vi "AlliGator.vi"() -> ()   [LabVIEW 2021, in "AlliGator GUI.lvlib"]
doc: "AlliGator main window.\nSpawned by AlliGator Launcher.vi.\nSpawns AlliGator Action Loop.vi, which handles UI requests from AlliGator.vi"
uses:
  AlliGator GUI.lvlib
  AlliGator Main Window Tabs.ctl
  Phasor/Phasor (g, s).ctl
  Source Image/AlliGator Displayed Image.ctl
  AlliGator State Indicator.ctl
  Phasor/Phasor (m, phi).ctl
  Phasor/Phasor Ratio Type.ctl
  Fits/IRF(X)PSED/Decay Fit Parameters & Derived Quantities List v2.ctl
  Phasor/Phasor Calibration Type.ctl
  Histograms/Linear Histogram Options.ctl
  Histograms/Histogram Bin Option.ctl
  Histograms/Histogram Bin Position.ctl
  Action Engine/AlliGator Q Element.ctl
  Action Engine/AlliGator Q Event.ctl
  AlliGator Dataset Ctrl Refnums.ctl
  AlliGator Other Ctrl Refnums.ctl
  AlliGator Registered Events Ctrl Refnums.ctl
  AlliGator Ctrl Refnums.ctl
  AlliGator Phasor Plot Ctrl Refnums.ctl
  AlliGator Phasor Graph Ctrl Refnums.ctl
  AlliGator Image Histogram Control Refnums.ctl
  Decay Fit Parameter Map/AlliGator Decay Fit Map Control Refnums.ctl
  Parameter Map/AlliGator Parameter Map Control Refnums.ctl
  Globals, Variables, Constants/AlliGator Refnums List.ctl
  Settings/AlliGator Settings List.ctl
  Rich Text Box/Text Format List.ctl
  Globals, Variables, Constants/AlliGator Variables List.ctl
  Palette/Image Palette Information.ctl
  Image/Image Display Palette Type.ctl
  Image/Image Display Event.ctl
  Image/Image Control Refnum.ctl
  <vilib>/Utility/miscctls.llb/LVPoint32TypeDef.ctl
  Decay Fit Parameter Map/AlliGator Decay Parameter Map Update Event Data.ctl
  Graphs/XY Graph/XY Graph Event.ctl
  Utilities/Read-Write.ctl
  Graphs/XY Graph/New Plot Information.ctl
  Graphs/Plot Scales.ctl
  Graphs/LabVIEW Plot Interpolation.ctl
  Graphs/Plot Point Style.ctl
  Graphs/XY Graph/XY Graph Mouse Click Event Data.ctl
  Graphs/XY Graph/XY Graph Refnum.ctl
  Parameter Map/AlliGator Parameter Map Update Event Data.ctl
  ROIs/AlliGator ROI Manager Actions.ctl
  AlliGator Image Mouse Up Event Data.ctl
  Image/Image ROI Descriptor.ctl
  Image/Image Contour Definition.ctl
  Image/Image Contour ID.ctl
  Image/Image ROI Type.ctl
  Parameter Map/AlliGator Parameter Map Display Range Mouse Move Data.ctl
  Image/Image Display User Event Data.ctl
  Action Engine/AlliGator Action Loop.vi
  Variant/Variant to Data/Variant to Boolean.vi
  Phasor/Phasor Abort Parallel Computation.vi
  Fits/Abort Fit Global.vi
  Image/Abort ROI Creation Global.vi
  Globals, Variables, Constants/AlliGator Abort.vi
  Variant/Variant to Data/Variant to [String].vi
  <vilib>/Utility/inputDevices.llb/keyboardAcquire.vi
  <vilib>/Utility/inputDevices.llb/mouseAcquire.vi
  Globals, Variables, Constants/AlliGator Globals.vi
  <vilib>/Utility/inputDevices.llb/closeKeyboard.vi
  <vilib>/Utility/inputDevices.llb/closeMouse.vi
  Action Engine/AlliGator Action Engine.lvlib
  Variant/Variant to Data/Variant to Data.lvlib
  Error/Error.lvlib
  Globals, Variables, Constants/AlliGator Globals, Variables & Constants.lvlib
  Image/Image.lvlib
  Palette/Palette.lvlib
  Notebook/Notebook.lvlib
  Graphs/XY Graph/XY Graph Add-Ons.lvlib
  Settings/AlliGator Settings.lvlib
  Phasor/Phasor.lvlib
  Fits/Fits.lvlib
  Phasor Calibration/AlliGator Phasor Calibration.lvlib
  Phasor Plot/AlliGator Phasor Plot.lvlib
  Source Image/AlliGator Source Image.lvlib
  Phasor Graph/AlliGator Phasor Graph.lvlib
  ROIs/AlliGator ROIs.lvlib
  GUI/GUI.lvlib
  Decay Fit Parameter Map/AlliGator Decay Fit Parameter Map.lvlib
  Python Plugins API/AlliGator Python Plugins.lvlib
  Sound/Sound.lvlib
  Graphs/Graphs.lvlib
  Decay Analysis/Decay Processing/AlliGator Decay Processing.lvlib
  Utilities/Utilities.lvlib
  Parameter Map/AlliGator Parameter Map.lvlib
  Histograms/Histogram Window.lvlib
panel:
  in  "Current ROI Analysis":bool
  in  "Scale Bar":bool
  in  "Refresh Image":bool
  in  "Clear Image Overlay":bool
  in  "Use ROI as Search Area":bool
  in  "Highlight Image ROI":bool
  in  "Phasor Overlay Color":u32(colorbox)=16777216
  in  "Gate Image Slide":u16(slide)=9 min=1 max=135 scale=1.0..201.0
  in  "Dataset File/Folder Path":path caption="File/Folder Path"
  out "Source Image":T1(plugin-control)
  out "True Pixel Value":dbl format="%#_5g"
  in  "Source Image ROI Selection":i32(c297)
  in  "Source Image ROI Color":u32(colorbox)=6618880 caption="ROI Color"
  in  "Time Point Slide":u16(slide)=65535 min=1 step=1 scale=1.0..1.1
  in  "Image Color Scale":dbl(ramp)
  in  "Channel Name":u16(ring) items=["Gate"]
  out "Current Time Stamp":dbl caption="Time Stamp" format="%#_5g"
  out "CPU":dbl[unit] format="%^#_4e"
  in  "Save Source Image":bool caption="Save Image"
  out "Current Data":string="Stained cancer cells" caption="Current Folder"
  in  "Displayed Image":T2=enum."Sum of All Gates"
  in  "Tab Control":T3=enum."Lifetime & Other Parameters"
  in  "Dataset File/Folder Path 2":path caption="File/Folder Path"
  in  "Histogram Lower Percentile":dbl=1.0 caption="Lower Percentile" min=0.0 max=100.0 format="%#.3f"
  in  "Histogram Upper Percentile":dbl=1.0 caption="100 - Upper Percentile" min=0.0 max=100.0 format="%#.3f"
  in  "Image Histogram Options":T4={"Bin Size"=1.0, "Bin Number"=256, "Bin Option"=enum."Bin Number", "Min Value"=-inf, "Max Value"=inf, "Filter NaN & Infinite Values"=TRUE, "Frequency Plot"=FALSE, "Align Bins"=TRUE, "Bin Location"=enum."Left", "Project Outside Values"=FALSE, "Max Histogram Size"=1000000} {"Max Histogram Size" format="%.0e"}
  in  "Auto-Adjust Contrast":bool=TRUE
  out "Lower Percentile":dbl=nan format="%#.3f"
  out "Upper Percentile":dbl=nan caption="100 - Upper Percentile" format="%#.3f"
  in  "Image Histogram Active":bool=TRUE
  in  "Use Image Histogram for Contrast":bool=TRUE
  out "Image Histogram":cluster{"X Array":dbl[], "Y Array":dbl[]}[](graph)
  in  "Dataset File/Folder Path 3":path caption="File/Folder Path"
  out "Decay Graph TipStrip":string caption="Lifetime Graph TipStrip"
  out "Decay Integrated Intensity":dbl=46949635.0 caption="Bkgd-subtracted Intensity" format="%#_5g"
  out "Decay Background":dbl caption="Background" format="%#_5g"
  out "Decay Lifetime":dbl[unit] caption="Lifetime" format="%#_5g"
  out "Decay Graph":cluster{"X Array":dbl[], "Y Array":dbl[]}[](graph)
  in  "Decay Graph Active":bool=TRUE
  in  "Dataset File/Folder Path 4":path caption="File/Folder Path"
  out "Decay Statistics TipStrip":string caption="Lifetime Graph TipStrip"
  out "Decay Statistics Graph":cluster{"X Array":dbl[], "Y Array":dbl[]}[](graph)
  in  "Decay Statistics Bin":i32=1 min=1
  in  "Dataset File/Folder Path 5":path caption="File/Folder Path"
  out "Intensity Time Trace TipStrip":string caption="Lifetime Graph TipStrip"
  in  "Intensity Correction File":path
  in  "Use Intensity Correction File":bool
  in  "Use File Timestamp":bool=TRUE
  out "Intensity Time Trace":cluster{"X Array":dbl[], "Y Array":dbl[]}[](graph)
  in  "Time Step":dbl[unit]=1.0 format="%#_5g"
  out "True Phasor Plot Value":i32
  in  "Dataset File/Folder Path 6":path caption="File/Folder Path"
  in  "Phasor ROI Decay":bool
  in  "Phasor Plot ROI Color":u32(colorbox)=6618880
  out "Phasor Plot Average Lifetime":dbl[unit]=nan caption="<tau>_a" format="%#_4e"
  out "Phasor Plot Phasor Ratio":dbl=nan caption="Amplitude Ratio (a1)" format="%#_4e"
  out "Phasor Plot Modulus Lifetime":dbl[unit]=nan caption="Modulus Lifetime" format="%#_4e"
  out "Phasor Plot Phase Lifetime":dbl[unit]=-9.431404035075279e-09 caption="Phase Lifetime" format="%#_4e"
  out "Phasor at cursor (m, phi)":T7={"m"=1.5330078000581284, "phi"=1.7786862539971595} caption="Phasor at Cursor (m, phi)" {"phi" format="%#_4e"; "m" format="%#_4e"}
  in  "Clear Phasor Overlay":bool
  in  "Phasor Plot ROI Selection":i32(c297)
  in  "Phasor Plot Active":bool
  in  "Phasor Plot Color Scale":dbl(ramp)
  out "Phasor at cursor (g, s)":T8={"g"=-0.31640625, "s"=1.5} caption="Phasor at Cursor" {"s" format="%#.3e"; "g" format="%#_4e"}
  in  "Phasor Plot Display Range":cluster{u32, u32}(slide)={0, 100} scale=0.0..987.0
  in  "Highlight Phasor in Source Image":bool caption="Highlight Phasor ROI"
  in  "Image Overlay Color":u32(colorbox)=16777216
  in  "Refresh Phasor Plot":bool caption="Refresh Phsor Plot"
  in  "Save Phasor Plot":bool
  out "Reference 2 Button":bool caption="Reference"
  out "Reference 1 Button":bool caption="Reference"
  in  "Phasor Plot Frequency":dbl[unit]=80000000.0 caption="Phasor Frequency"
  in  "Overlay Mode":u16(ring)
  out "Phasor Plot Image":T1(plugin-control)
  in  "Dataset File/Folder Path 7":path caption="File/Folder Path"
  out "Phasor Graph TipStrip":string caption="Lifetime Graph TipStrip"
  out "Average Lifetime SDV":dbl[unit]=nan caption="+/-" format="%#.3g"
  out "Phasor Ratio SDV":dbl=nan caption="+/-" format="%#.3g"
  out "Modulus Lifetime SDV":dbl[unit]=nan caption="+/-" format="%#.3g"
  out "Phase Lifetime SDV":dbl[unit]=nan caption="+/-" format="%#.3g"
  in  "Calibration Type":T9
  out "Phasor Graph Average Lifetime":dbl[unit]=nan caption="<tau>_a" format="%#.3g"
  in  "Phasor Graph Active":bool
  in  "Refresh SEPL":bool
  out "Phasor Graph Phasor Ratio":dbl=nan caption="Amplitude Ratio (a1)" format="%#.3g"
  out "Phasor Graph Modulus Lifetime":dbl[unit]=nan caption="Modulus Lifetime" format="%#.3g"
  in  "Phasor Reference 2 Control":dbl(c297)
  in  "Save Phasor Graph Image":bool
  in  "Current Phasor (m, phi)":T7={"m"=nan, "phi"=nan} {"phi" format="%#_4g"; "m" format="%#_4g"}
  in  "Phasor Reference 1 Control":dbl(c297)
  in  "Single Step Phasor":bool
  in  "Phasor Frame Slide":i32(slide) caption="Phasor Frame Slider" min=0 step=1 scale=1.0..1.1
  out "Phase Lifetime 2":dbl[unit]=nan format="%#.3g"
  out "Phase Lifetime 1":dbl[unit]=nan format="%#.3g"
  in  "Show Line":bool
  out "Phasor Graph Phase Lifetime":dbl[unit]=nan caption="Phase Lifetime" format="%#.3g"
  in  "Current Phasor (g, s)":T8={"g"=nan, "s"=nan} caption="Current Phasor" {"s" format="%#_4g"; "g" format="%#_4g"}
  out "Phasor Graph":cluster{"X Array":dbl[], "Y Array":dbl[]}[](graph)
  in  "Phasor Graph Frequency":dbl[unit]=80000000.0 caption="Phasor Frequency"
  in  "Calibration Lifetime":dbl[unit] min=0.0
  in  "Dataset File/Folder Path 8":path caption="File/Folder Path"
  out "Phasor Ratio Graph TipStrip":string caption="Lifetime Graph TipStrip"
  in  "Phasor Ratio Type":T10
  out "Phasor Ratio Graph":cluster{"X Array":dbl[], "Y Array":dbl[]}[](graph)
  in  "Dataset File/Folder Path 9":path caption="File/Folder Path"
  out "Lifetime & Other Parameters Graph TipStrip":string caption="Lifetime Graph TipStrip"
  out "Lifetime & Other Parameters Graph":cluster{"X Array":dbl[], "Y Array":dbl[]}[](graph)
  in  "Dataset File/Folder Path 10":path caption="File/Folder Path"
  in  "Decay Fit Parameter Map ROI Color":u32(colorbox)=6618880
  in  "Overlay Decay Fit Parameter Map":bool
  out "Decay Fit Max Parameter":dbl=1.0 caption="Max Parameter"
  out "Decay Fit Min Parameter":dbl caption="Min Parameter"
  in  "Refresh Decay Fit Parameter Map":bool
  in  "Decay Fit Parameter":T11
  in  "Decay Fit Parameter Map Color Scale":dbl(ramp)
  in  "Decay Fit Parameter Map Display Range":cluster{dbl, dbl}(slide)={0.0, 1.0} scale=0.0..1.0
  out "Decay Parameter Map Value":dbl caption="Map Value"
  out "Decay Parameter Map Y":i32 caption="Y"
  out "Decay Parameter Map X":i32 caption="X"
  out "Decay Fit Parameter Map Image":T1(plugin-control)
  out "Parameter Map X":i32 caption="X"
  out "Parameter Map Y":i32 caption="Y"
  out "Parameter Map Value":dbl caption="Map Value"
  in  "Parameter Map Set":u16(ring)
  in  "Map Parameter":u16(ring)
  in  "Dataset File/Folder Path 11":path caption="File/Folder Path"
  in  "Parameter Map ROI Color":u32(colorbox)=6618880 caption="Decay Fit Parameter Map ROI Color"
  in  "Overlay Parameter Map":bool
  out "Map Max Parameter":dbl=1.0 caption="Max Parameter"
  out "Map Min Parameter":dbl caption="Min Parameter"
  in  "Refresh Parameter Map":bool
  in  "Parameter Map Color Scale":dbl(ramp)
  in  "Parameter Map Display Range":cluster{dbl, dbl}(slide)={0.0, 1.0} scale=0.0..20.0
  out "Parameter Map Image":T1(plugin-control)
  out "Event LED":bool
  out "Message":string
  out "Progress Bar":dbl(slide) scale=0.0..100.0
  in  "Abort ROI Creation":bool
  in  "Abort Fit":bool
  in  "Abort":bool
  out "Animated Busy Icon":bool=TRUE
  out "State Indicators":T12
  # "Drop the content of this VI on AlliGator's diagram\nIn AlliGator, replace the subVI template by a new version"
  # "Drop the content of this VI on AlliGator's diagram\nIn AlliGator, replace the subVI template by a new version"
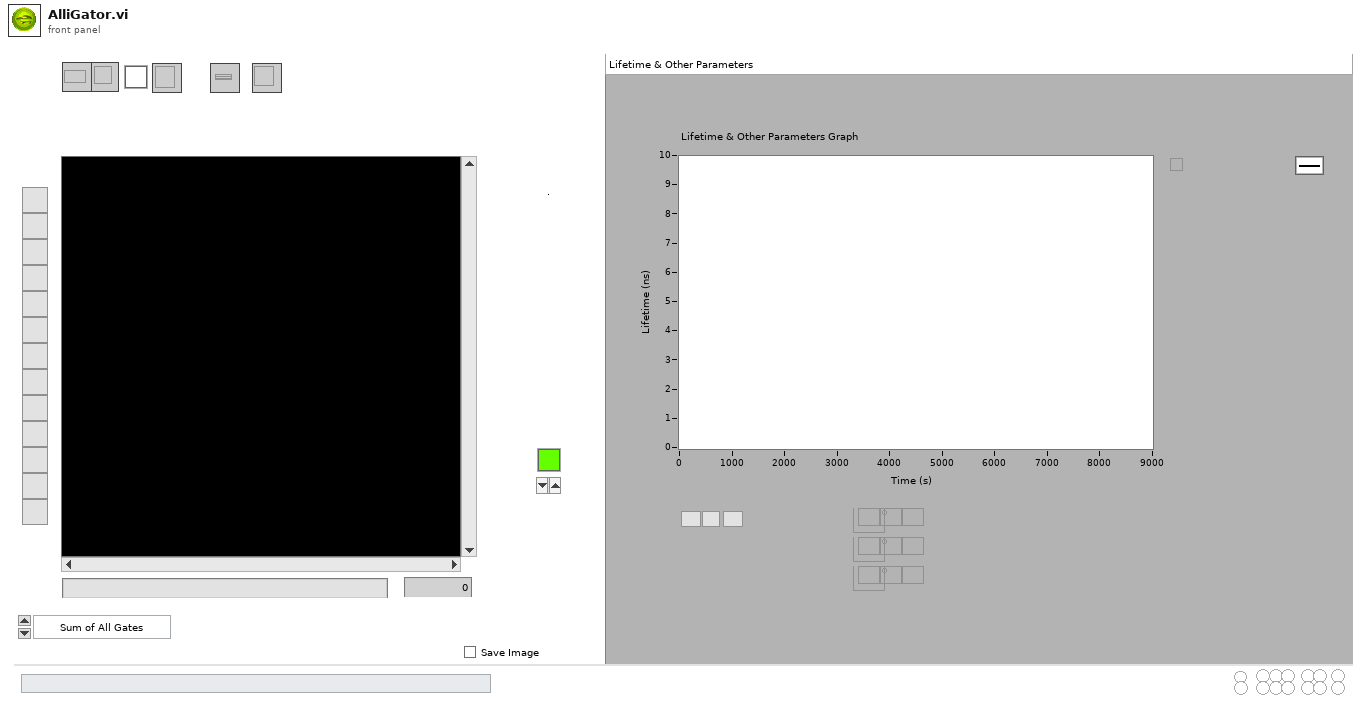
[diagram p1: front panel]
types:
  T1 = typedef "IMAQ Image.ctl" = refnum<image>
  T2 = typedef "AlliGator Source Image.lvlib/AlliGator Displayed Image.ctl" = enum16{"Single Gate", "Sum of All Gates", "Max of All Gates", "Min of All Gates", "-", "White Ligth Image", "Mask Image"}
  T3 = typedef "AlliGator GUI.lvlib/AlliGator Main Window Tabs.ctl" = enum32{"Image Histogram", "Fluorescence Decay", "Fluorescence Decay Statistics", "Intensity Time Trace", "Phasor Plot", "Phasor Graph", "Phasor Ratio", "Lifetime & Other Parameters", "Decay Fit Parameter Map", "Parameter Map"}
  T4 = typedef "Histogram Window.lvlib/Linear Histogram Options.ctl" = cluster{"Bin Size":dbl, "Bin Number":i32, "Bin Option":T5, "Min Value":dbl, "Max Value":dbl, "Filter NaN & Infinite Values":bool, "Frequency Plot":bool, "Align Bins":bool, "Bin Location":T6, "Project Outside Values":bool, "Max Histogram Size":i32}
  T5 = typedef "Histogram Window.lvlib/Histogram Bin Option.ctl" = enum32{"Bin Number", "Bin Size"}
  T6 = typedef "Histogram Window.lvlib/Histogram Bin Position.ctl" = enum16{"Left", "Center", "Right"}
  T7 = typedef "Phasor.lvlib/Phasor (m, phi).ctl" = cluster{"m":dbl, "phi":dbl}
  T8 = typedef "Phasor.lvlib/Phasor (g, s).ctl" = cluster{"g":dbl, "s":dbl}
  T9 = typedef "Phasor.lvlib/Phasor Calibration Type.ctl" = enum16{"None", "Single Phasor", "Phasor Series", "Phasor Map"}
  T10 = typedef "Phasor.lvlib/Phasor Ratio Type.ctl" = enum32{"Intensity-weighted", "Amplitude-weighted"}
  T11 = typedef "Fits.lvlib/Decay Fit Parameters & Derived Quantities List v2.ctl" = enum16{"Offset", "Baseline", "A_1", "tau_1", "A_2", "tau_2", "<tau>_a", "f1_a", "f2_a", "<tau>_i", "f1_i", "f2_i", "-", "R^2", "Chi^2"}
  T12 = typedef "AlliGator GUI.lvlib/AlliGator State Indicator.ctl" = cluster{"Phasor Calibration Defined":bool, "Phasor Calibration Series Defined":bool, "Phasor Calibration Map Defined":bool, "Phasor Ratio Reference 1 Defined":bool, "Phasor Ratio Reference 2 Defined":bool, "Phasor Ratio Lifetime Reference 1 Defined ":bool, "Phasor Ratio Lifetime Reference 2 Defined":bool, "Phasor Calibration Used":bool, "Phasor Calibration Series Used":bool, "Phasor Calibration Map Used":bool, "Dataset Update Needed":bool, "Phasor Plot Update Needed":bool, "Reference/IRF Defined":bool, "Individual IRFs Defined":bool}
  T13 = typedef "AlliGator Globals, Variables & Constants.lvlib/AlliGator Refnums List.ctl" = enum16{"---------- AlliGator Controls ----------", "AlliGator Tab Control Refnum", "---------- AlliGator Indicators ----------", "Source Image Display Refnum", "Phasor Plot Display Refnum", "Decay Fit Parameter Map Refnum", "---------- AlliGator VIs ----------", "AlliGator Refnum", "AlliGator Settings Refnum", "AlliGator Launcher Refnum"}
  T14 = typedef "AlliGator Parameter Map.lvlib/AlliGator Parameter Map Control Refnums.ctl" = cluster{"Parameter Map Color Scale":refnum<vi>, "Map Parameter":refnum<vi>, "Max Parameter":refnum<vi>, "Min Parameter":refnum<vi>, "Parameter Map Display":refnum<vi>, "Parameter Map Display Range":refnum<vi>, "Parameter Map Set":refnum<vi>, "Parameter Map X":refnum<vi>, "Parameter Map Y":refnum<vi>, "Parameter Map Value":refnum<vi>}
  T15 = enum32{"Invalid", "Standard", "Closed", "Hidden", "Minimized", "Maximized"}
  T16 = enum32{"Image Histogram", "Fluorescence Decay", "Fluorescence Decay Statistics", "Intensity Time Trace", "Phasor Plot", "Phasor Graph", "Phasor Ratio", "Lifetime & Other Parameters", "Decay Fit Parameters Map", "Parameter Map"}
  T17 = typedef "AlliGator Decay Fit Parameter Map.lvlib/AlliGator Decay Fit Map Control Refnums.ctl" = cluster{"Decay Fit Parameter Map Color Scale":refnum<vi>, "Decay Fit Parameter":refnum<vi>, "Max Parameter":refnum<vi>, "Min Parameter":refnum<vi>, "Decay Fit Parameter Map Display":refnum<vi>, "Decay Fit Parameter Map Display Range":refnum<vi>, "Decay Parameter Map X":refnum<vi>, "Decay Parameter Map Y":refnum<vi>, "Decay Parameter Map Value":refnum<vi>}
  T18 = typedef "AlliGator GUI.lvlib/AlliGator Image Histogram Control Refnums.ctl" = cluster{"Image Histogram":refnum<vi>, "Image Histogram Options":refnum<vi>, "Image Histogram Active":refnum<vi>, "Image Histogram Upper Percentile":refnum<vi>, "Image Histogram Lower Percentile":refnum<vi>, "Auto-Adjust Contrast":refnum<vi>}
  T19 = typedef "AlliGator GUI.lvlib/AlliGator Phasor Graph Ctrl Refnums.ctl" = cluster{"Phasor Ratio":refnum<vi>, "Modulus Lifetime":refnum<vi>, "Phasor at cursor (m, phi)":refnum<vi>, "Phase Lifetime":refnum<vi>, "Phasor at cursor (g, s)":refnum<vi>, "Phasor Graph Average Lifetime":refnum<vi>, "Phasor Graph Active":refnum<vi>, "Save Phasor Graph":refnum<vi>, "Phasor Frame Slide":refnum<vi>, "Single Step Phasor":refnum<vi>, "Calibration Type":refnum<vi>, "Show Line":refnum<vi>, "Phase Lifetime 1":refnum<vi>, "Phase Lifetime 2":refnum<vi>, "Phasor Graph Frequency":refnum<vi>, "Phasor Reference 1 Control":refnum<vi>, "Phasor Reference 2 Control":refnum<vi>, "Calibration Lifetime":refnum<vi>, "Phase Lifetime SDV":refnum<vi>, "Average Lifetime SDV":refnum<vi>, "Phasor Ratio SDV":refnum<vi>, "Modulus Lifetime SDV":refnum<vi>}
  T20 = typedef "AlliGator GUI.lvlib/AlliGator Phasor Plot Ctrl Refnums.ctl" = cluster{"Phasor Ratio":refnum<vi>, "Modulus Lifetime":refnum<vi>, "Phasor at cursor (m, phi)":refnum<vi>, "Phase Lifetime":refnum<vi>, "Phasor at cursor (g, s)":refnum<vi>, "Phasor Plor Average Lifetime":refnum<vi>, "Phasor Plot Active":refnum<vi>, "Save Phasor Plot":refnum<vi>, "Image Overlay Color":refnum<vi>, "Phasor Plot Color Scale":refnum<vi>, "Reference 1 Button":refnum<vi>, "Reference 2 Button":refnum<vi>, "True Phasor Plot Value":refnum<vi>}
  T21 = typedef "AlliGator GUI.lvlib/AlliGator Ctrl Refnums.ctl" = cluster{"Other AlliGator Ctrl Refnums":T22, "Phasor Plot Ctrl Refnums":T20, "Phasor Graph Ctrl Refnums":T19, "Dataset Control Refnums":T23, "Registered Events Ctrl Refnums":T24, "Image Histogram Ctrl Refnums":T18, "Decay Fit Map Ctrl Refnums":T17, "Parameter Map Ctrl Refnums":T14}
  T22 = typedef "AlliGator GUI.lvlib/AlliGator Other Ctrl Refnums.ctl" = cluster{"State Indicators":refnum<vi>, " Progress Bar":refnum<vi>, "Decay Graph Active":refnum<vi>, "Decay Statistics Bin":refnum<vi>, "Time Step":refnum<vi>, "Use File Timestamp":refnum<vi>, "Tab Control":refnum<vi>, "CPU":refnum<vi>, "Abort Fit":refnum<vi>, "Dataset File/Folder Path":refnum<vi>, "Abort ROI Creation":refnum<vi>, "Event LED":refnum<vi>, "Dataset File/Folder Path 2":refnum<vi>, "Dataset File/Folder Path 3":refnum<vi>, "Dataset File/Folder Path 4":refnum<vi>, "Dataset File/Folder Path 5":refnum<vi>, "Dataset File/Folder Path 6":refnum<vi>, "Dataset File/Folder Path 7":refnum<vi>, "Dataset File/Folder Path 8":refnum<vi>, "Dataset File/Folder Path 9":refnum<vi>, "Dataset File/Folder Path 10":refnum<vi>, "Dataset File/Folder Path 11":refnum<vi>}
  T23 = typedef "AlliGator GUI.lvlib/AlliGator Dataset Ctrl Refnums.ctl" = cluster{"Current Data":refnum<vi>, "Gate Image Slide":refnum<vi>, "Time Point Slide":refnum<vi>, "Current Time Stamp":refnum<vi>, "Save Image":refnum<vi>, "Displayed Image":refnum<vi>, "Overlay Mode":refnum<vi>, "Phasor Overlay Color":refnum<vi>, "Image Color Scale":refnum<vi>, "Use ROI as Search Area":refnum<vi>, "Source Image ROI Color":refnum<vi>, "True Pixel Value":refnum<vi>}
  T24 = typedef "AlliGator GUI.lvlib/AlliGator Registered Events Ctrl Refnums.ctl" = cluster{"Time Point Slider":refnum<vi>, "Phasor Plot Display Range":refnum<vi>, "Decay Graph":refnum<vi>, "Decay Statistics Graph":refnum<vi>, "Intensity Time Trace":refnum<vi>, "Phasor Graph":refnum<vi>, "Phasor Ratio Graph":refnum<vi>, "Lifetime Graph":refnum<vi>, "Phasor Plot Display":refnum<vi>, "Source Image Display":refnum<vi>, "Decay Fit Parameter Map Display Range":refnum<vi>, "Decay Fit Parameter Map Display":refnum<vi>, "Parameter Map Display Range":refnum<vi>, "Parameter Map Display":refnum<vi>, "Phasor Plot Display Range":refnum<vi>}
  T25 = typedef "AlliGator Action Engine.lvlib/AlliGator Q Event.ctl" = enum16{"---- Files ----", "Files:Set Batch Export Files To Save", "Files:Set Dataset Loading & Pre-processing Options", "Files:Check #Frames in Dataset", "Files:Increment Frame Index", "Files:Open Mask Image", "Files:Open White Light Image", "Files:Open Single Dataset", "Files:New Folder of Folders Selected", "Files:Load File (all Types)_Scriptable", "Files:Move Flattened Series to Folders Series", "Files:Select Folder", "Files:Load FLI Dataset", "Files:Load Swiss SPAD 1 Dataset", "Files:Load Swiss SPAD 2 Dataset", "Files:Load .sdt FLI Dataset", "Files:Load .ptu FLI Dataset", "Files:Load .bin FLI Dataset", "Files:Load Single Gate Image Folder", "Files:Load I/m/phi Dataset (deprecated)", "Files:Load Single Image", "Files:Subtract Background File", "Files:Export FLI Dataset", "Files:Load HDF5 FLI Dataset", "Files:Set Destination File Path", "Files:Save Mask Image", "Files:Batch Conversion", "Files:New Folder Selected", "Files:Close FLI Dataset", "Files:Close FLI Dataset Series", "Files:Close White Light Image", "Files:Close Mask Image", "---- FLI Dataset ----", "FLI Dataset:Channel Arithmetic", "FLI Dataset:Export Average Lifetime Map as ASCII", "FLI Dataset:Export User-Defined Quantity Map as ASCII", "FLI Dataset:Python Function FLI Dataset Event", "FLI Dataset:ROI Analysis", "FLI Dataset:Tilted Logistic Square Gated IRF Characteristics Map", "FLI Dataset:Logistic Square Gated IRF Characteristics Map", "FLI Dataset:Square Gated IRF Characteristics Map", "FLI Dataset:Multi-ROI Single-Pixel Phasor Analysis", "FLI Dataset:Multi-ROI Single-Pixel NLSF Analysis", "FLI Dataset:All ROIs IRF Extraction", "FLI Dataset:All ROIs Decay Fit Non-Interactive (Fast + Individual IRF)", "FLI Dataset:All ROIs Phasor Analysis", "FLI Dataset:All ROIs Decay Fit", "FLI Dataset:Fluorescence Decay Statistics", "FLI Dataset:Update Decay Statistics Graph", "FLI Dataset:Get Decay from ROI", "FLI Dataset:All ROIs Average Lifetimes", "FLI Dataset:Save/Load Local IRFs", "FLI Dataset:Clear Local IRFs", "FLI Dataset:Phasor Calibration Maps (# Gates Series) Script", "FLI Dataset:Calibrated Phasor Map Series", "---- FLI Dataset Series ----", "FLI Dataset Series:Sum All Datasets in Series", "FLI Dataset Series:Add Dataset to Accumulated Dataset", "FLI Dataset Series:Display Accumulated Dataset", "FLI Dataset Series:Clear Dataset Series Sum", "FLI Dataset Series:Time-Series Analysis (NLSF)", "FLI Dataset Series:Time-Series Analysis (Phasor)", "---- Image ----", "Image:Update Image Profile Plots", "Image:Image Histogram Cursor Move", "Image:Image Histogram", "Image:Image Contrast", "Image:Set Image Histogram Cursor Move Flag", "Image:Clear Image Overlay", "Image:Use ROI as Search Area", "Image:Set ROI Diameter", "Image:Save Image Data as TIFF", "Image:Save Displayed Image with Overlay", "Image:Save Image Overlay Only", "Image:Save Image as Hot Pixel Mask", "Image:Change Source Image Color Palette", "Image:Copy Image to Clipboard", "Image:Source Image ROI Selection", "Image:Delete All ROIs", "Image:Delete All Unselected ROIs", "Image:Delete ROI", "Image:Merge All ROIs", "Image:Store ROI", "Image:Source Image ROI Storage", "Image:Export ROI Description to Notebook", "Image:Save ROI", "Image:Load ROI", "Image:Paste ROI Definition", "Image:Clear ROI", "Image:Identify ROIs in Mask Image", "Image:Create Complementary ROI", "Image:Create Contour ROI", "Image:Create ROI(s) from Pixels with Peak above Min_Scriptable", "Image:Create ROI(s) from Pixels with Intensity above Min_Scriptable", "Image:Compute ROI Statistics", "Image:Delete ROI(s) based on ROI Characteristics", "Image:Create ROI Grid", "Image:ROI to Individual Pixel ROIs", "Image:Python Function Source Image Event", "Image:Show Phasor Calibration Map ROI Centers", "Image:Convert ROI to Mask Image", "Image:Mouse Move", "Image:Mouse Up", "Image:Set Source Image Mouse Move Flag", "Image:Add Scale Bar Overlay", "Image:Delete Existing ROIs Option", "Image:Overlay ROI Median", "Image:Check Current ROI", "Image:Update True Pixel Value", "---- Decay ----", "Decay:Clear IRF/Reference Plot", "Decay:Add Decay to Graph", "Decay:Smoothen Plot", "Decay:Smoothen Plot Tail", "Decay:Average Selected Plots", "Decay:Extract IRF", "Decay:Optimal IRF Extraction", "Decay:Threshold IRF", "Decay:Fit to Model IRF", "Decay:Fit IRF to Square Gate", "Decay:Fit IRF to Logistic Square Gate", "Decay:Fit IRF to Tilted Logistic Square Gate", "Decay:Create Bounding Cursors Set", "Decay:Export Bounding Cursors Definition to Notebook", "Decay:Denoise Plot", "Decay:Compute Cumulative Function", "Decay:Use as Reference Decay", "Decay:Show Reference Decay/IRF", "Decay:Extrapolate Decay", "Decay:Create Head & Tail Bounding Cursors", "Decay:Store Cursor-defined Head & Tail Fractions", "Decay:Rebin Plot", "Decay:1-Normalize Decay", "Decay:[0-1]-Normalize Plot", "Decay:Straighten Decay", "Decay:Shift Decay", "Decay:Fold Decay", "Decay:Fit Decay", "Decay:Global Fit of Selected Decays", "Decay:Post Global Fit Script", "Decay:Add Global Fit Parameters to Graph", "Decay:Add Decay Parameter(s) to Plot (Graph)", "Decay:Export Decay to Phasor Graph", "Decay:Compute Average Lifetime", "Decay:Plot Convolution", "Decay:Graph Tip Strip Update", "---- Decay Statistics ----", "Decay Statistics:Tip Strip Update", "---- Intensity Time Trace ----", "Intensity Time Trace:Use File Timestamp", "Intensity Time Trace:Load Intensity Corrections File", "Intensity Time Trace:Clear Intensity Corrections File", "Intensity Time Trace:Tip Strip Update", "---- Phasor Plot ----", "Phasor Plot:Build Phasor Plot", "Phasor Plot:Change Phasor Plot Color Palette", "Phasor Plot:Adjust Phasor Plot Display Range", "Phasor Plot:Highlight Image ROI in Phasor Plot", "Phasor Plot:Save Phasor Plot Image with Overlay", "Phasor Plot:Export Complex Phasor Map", "Phasor Plot:Export Phasor Ratio Map", "Phasor Plot:Export Average Lifetime Map", "Phasor Plot:Compute Phase Lifetime Histogram", "Phasor Plot:Compute Phasor Ratio Histogram", "Phasor Plot:Compute Phase Lifetime vs Intensity Scatter Plot", "Phasor Plot:Weber 2-Component Decomposition", "Phasor Plot:Update Phasor Color Map Vertices", "Phasor Plot:Clear Phasor Overlay", "Phasor Plot:Use Segment Extremities as References", "Phasor Plot:Use UC/Segment Intersections as References", "Phasor Plot:Use UC/Principal Axis Intersections as References", "Phasor Plot:Use UC/Linear Fit Intersections as References", "Phasor Plot:Update Phasor Plot Reference", "Phasor Plot:Show Local Phasor Info in Phasor Plot", "Phasor Plot:Update Phasor Plot State", "Phasor Plot:Phasor Plot ROI Storage", "Phasor Plot:Phasor Plot ROI Selection", "Phasor Plot:Python Function Phasor Plot Event", "Phasor Plot:Overlay Phasor ROI, Ratio or Map in Source Image", "Phasor Plot:Compute Decay of Selected Phasors", "Phasor Plot:Phasor at Image Pixel", "Phasor Plot:Mouse Move", "Phasor Plot:Mouse Up", "Phasor Plot:Display Range Mouse Move", "Phasor Plot:Set Mouse Move Flag", "Phasor Plot:Update True Phasor Plot Value", "---- Phasor Graph ----", "Phasor Graph:Get Phasor Value", "Phasor Graph:Create New Phasor Plot Dialog", "Phasor Graph:Update Last Phasor Value", "Phasor Graph:Update Phasor (m, phi)", "Phasor Graph:Remove Single Phasor from Plot", "Phasor Graph:Add Single Phasor to Plot", "Phasor Graph:Remove Phasor Plot", "Phasor Graph:Remove Selected Phasor Plots", "Phasor Graph:Clear Phasor Data", "Phasor Graph:Clear Phasor Graph", "Phasor Graph:Cursor Move", "Phasor Graph:Draw Cursor Connecting Line", "Phasor Graph:Clear Cursor Connecting Line", "Phasor Graph:Find UC Intersection", "Phasor Graph:Use UC/Cursor-Defined Line Intersections", "Phasor Graph:Use Selected Plots Fitted Line/UC Intersections", "Phasor Graph:Use Selected Plots Principal Axis/UC Intersections", "Phasor Graph:Show Single Phasor", "Phasor Graph:Save Single Phasor Plot", "Phasor Graph:Save All Phasor Plots", "Phasor Graph:Load Phasor Plot(s)", "Phasor Graph:Phasor Multiplication", "Phasor Graph:Compute Average Phasor", "Phasor Graph:Compute Multiple Average Phasors (Selected Plots)", "Phasor Graph:Export Single Phasor Plot Phase Lifetimes", "Phasor Graph:Parameter 2 vs Parameter 1 Scatter Plot", "Phasor Graph:Use Cursor n Location", "Phasor Graph:Set Reference n to Current Phase Lifetime Value", "Phasor Graph:Set Reference n to Lifetime Value", "Phasor Graph:Set Cursor n Location", "Phasor Graph:Save Phasor Graph Image", "Phasor Graph:Update SEPL Plot", "Phasor Graph:Export Single Phasor Plot Data", "Phasor Graph:Export Selected Phasor Plots Data", "Phasor Graph:Python Function Phasor Graph Event", "Phasor Graph:Tip Strip Update", "---- Calibration ----", "Calibration:Set Calibration Type", "Calibration:Load/Save Phasor Calibration", "Calibration:Load/Save Phasor Calibration Series", "Calibration:Load/Save Phasor Calibration Map", "Calibration:Use as Calibration", "Calibration:Compute Optimal Calibration from Phasor References", "Calibration:Clear Phasor Calibration", "Calibration:Single Phasor Calibration Information", "Calibration:Use as Calibration Series", "Calibration:Use as Calibration Map", "Calibration:Clear Calibration Series", "Calibration:Phasor Calibration Series Information", "Calibration:Clear Calibration Map", "Calibration:Phasor Calibration Map Information", "Calibration:Apply Phasor Calibration", "Calibration:Update Single Plot Calibration", "Calibration:Update Multiple Plots Calibration", "Calibration:Clear Single Plot Calibration", "Calibration:Clear All Plots Calibrations", "Calibration:Clear Plot(s) Calibration(s)?", "---- Phasor Ratio ----", "Phasor Ratio:Clear Reference n", "Phasor Ratio:Toggle Selected Plot(s)  Lock to Reference 1", "Phasor Ratio:Use as Reference n", "Phasor Ratio:Send Reference n to Notebook", "Phasor Ratio:Toggle Selected Plot(s)  Lock to Reference 2", "Phasor Ratio:Compute Phasor Ratio at Mouse Location", "Phasor Ratio:Compute Phasor Plot's Average Phasor Ratio", "Phasor Ratio:Compute Time-Series Phasor Ratios", "Phasor Ratio:Fit Line to Phasor Ratio Plot", "Phasor Ratio:Save References", "Phasor Ratio:Load References", "Phasor Ratio:Update Phasor Reference 1", "Phasor Ratio:Update Phasor Reference 2", "Phasor Ratio:Move Cursor n to Reference n", "Phasor Ratio:Use as Phasor Reference 1 Lifetime", "Phasor Ratio:Use as Phasor Reference 2 Lifetime", "Phasor Ratio:Export Phasor Ratio Map as ASCII", "Phasor Ratio:Tip Strip Update", "---- Lifetime & Other Parameters Graph ----", "Lifetime:Compute Sliced Mean, SDV and CV Plots", "Lifetime:Plot Decay Shifts", "Lifetime:Plot Histogram", "---- Decay Fit Parameter Map ----", "Decay Fit Parameter Map:Export ROI NLSF Data as ASCII", "Decay Fit Parameter Map:Set Decay Fit Parameter Map Selection", "Decay Fit Parameter Map:Build Decay Fit Parameter Map", "Decay Fit Parameter Map:Change Decay Fit Parameter Map Color Palette", "Decay Fit Parameter Map:Export Decay Fit Parameter Map Data as ASCII", "Decay Fit Parameter Map:Export All Decay Fit Parameter Maps Data as ASCII", "Decay Fit Parameter Map:Selected Parameter Scatterplot", "Decay Fit Parameter Map:Parameter 2 vs Parameter 1 Scatterplot", "Decay Fit Parameter Map:Save Decay Fit Parameter Map Image", "Decay Fit Parameter Map:Save-Load IRFs & Fit Data", "Decay Fit Parameter Map:Update Local Decay Plots", "Decay Fit Parameter Map:Python Function Decay Fit Parameters Map Event", "Decay Fit Parameter Map:Overlay Decay Fit Parameter Map in Source Image", "Decay Fit Parameter Map:Selected Parameter vs Intensity Scatterplot", "Decay Fit Parameter Map:Mouse Up", "Decay Fit Parameter Map:Mouse Move", "Decay Fit Parameter Map:Display Range Mouse Move", "Decay Fit Parameter Map:Change Map Resolution", "Decay Fit Parameter Map:Variance Significance Maps", "Decay Fit Parameter Map:Fit Result Constraints Window", "---- Parameter Map ----", "Parameter Map:Export ROI Parameters Data as ASCII", "Parameter Map:Delete Parameter Map Set", "Parameter Map:Update Parameter List", "Parameter Map:Build Parameter Map", "Parameter Map:Change Parameter Map Color Palette", "Parameter Map:Export Parameter Map Data as ASCII", "Parameter Map:Export All Parameter Maps Data as ASCII", "Parameter Map:Selected Parameter Scatterplot", "Parameter Map:Parameter 2 vs Parameter 1 Scatterplot", "Parameter Map:Selected Parameter vs Intensity Scatterplot", "Parameter Map:Save Parameter Map Image", "Parameter Map:Save-Load IRFs & Parameter Maps (TODO)", "Parameter Map:Set Parameter Map Selection", "Parameter Map:Python Function Parameter Map Event", "Parameter Map:Overlay Parameter Map in Source Image", "Parameter Map:Update Local Decay Plots", "Parameter Map:Mouse Up", "Parameter Map:Mouse Move", "Parameter Map:Display Range Mouse Move", "---- Generic Graph ----", "Generic Graph:Generic XY Graph Event", "Generic Graph:Python Function XY Graph Event", "Generic Graph:New Plot", "Generic Graph:Save Plot", "Generic Graph:XY Plot Histogram", "Generic Graph:Set XY Graph Plot Name", "Generic Graph:Set Last Cursor Style", "Generic Graph:Tip Strip Update", "---- GUI ----", "GUI:Start Script", "GUI:Type of Displayed Image Changed", "GUI:Gate Image Slide Changed", "GUI:Show Busy Icon", "GUI:Show Busy Icon & Abort Button", "GUI:Hide Busy Icon", "GUI:Hide Busy Icon & Abort Button", "GUI:Abort", "GUI:End Script", "GUI:Start Timing", "GUI:End Timing", "GUI:Set State Indicator", "GUI:Send Parameters JSON Strings to Clipboard", "GUI:Set Gate Step", "GUI:Idle", "GUI:Initialization", "GUI:Quit", "GUI:Increment Dataset Index", "GUI:Set Dataset Index to -1", "GUI:Time Series Slider Moved", "GUI:Time Series Slider Changed", "GUI:Toggle Playback or Loop", "GUI:Playback Script", "GUI:Set Phasor Frequency", "GUI:Open Window", "GUI:Start Test Script", "GUI:End Test Script", "GUI:Set Verbose Mode", "GUI:Set Verbose Settings Mode", "DEBUG"}
  T26 = typedef "AlliGator Action Engine.lvlib/AlliGator Q Element.ctl" = cluster{"AlliGator Q Event":T25, "Data":variant}
  T27 = typedef "AlliGator GUI.lvlib/AlliGator Events Registration.ctl" = cluster{"Phasor Plot Display Event":refnum<event-registration>, "Source Image Display Event":refnum<event-registration>, "Phasor Display Range Event":refnum<event-registration>, "Time Point Slider Event":refnum<event-registration>, "Other Events":refnum<event-registration>, "Decay Fit Parameter Map Display Range Event":refnum<event-registration>, "Decay Fit Parameter Map Display Event":refnum<event-registration>, "Parameter Map Display Range Event":refnum<event-registration>, "Parameter Map Display Event":refnum<event-registration>, "Phasor Plot Display Range Event":refnum<event-registration>, "Decay Graph TipStrip Event":refnum<event-registration>, "Decay Graph Statistics TipStrip Event":refnum<event-registration>, "Intensity Time Trace TipStrip Event":refnum<event-registration>, "Phasor Graph TipStrip Event":refnum<event-registration>, "Phasor Ratio Graph TipStrip Event":refnum<event-registration>, "Lifetime Graph TipStrip Event":refnum<event-registration>}
  T28 = typedef "AlliGator Progress Bar Q Element.ctl" = cluster{"Action":string, "Value":dbl}
  T29 = typedef "Notebook.lvlib/Text Format List.ctl" = enum16{"Message", "Result", "Error", "Setting", "Verbose", "Warning"}
  T30 = typedef "AlliGator Settings.lvlib/AlliGator Settings List.ctl" = enum16{"GUI:Visible Settings Tab", "GUI:Last Run Version", "Source Image:Use Image Histogram for Contrast", "Source Image:Low Count Pixels Rejection Options", "Source Image:High Count Pixels Rejection Options", "Source Image:Use Image Brightness", "Source Image:Blend Overlay with Image Background", "Source Image:Use Fixed ROI Diameter", "Source Image:ROI Diameter", "Source Image:ROI Center Color", "Source Image:Peak Threshold", "Source Image:Intensity Threshold", "Source Image:Image Binning Options", "Source Image:Image Smoothing Options", "Source Image:Image Histogram Active", "Source Image:Invert Binary Mask", "Source Image:Hot Pixel Removal", "Source Image:Overlay Analyzed ROI Center", "Source Image:Auto-Adjust Contrast", "Source Image:Histogram Lower Percentile", "Source Image:Histogram Upper Percentile", "Source Image:Save Source Image", "Source Image:Scale Bar Options", "Source Image:Image Resolution (Pixel Size)", "Source Image:Flatfield Correction", "Source Image:Show Dead Left Columns Correction", "Source Image:Dead Left Columns Correction", "Source Image:Image Pre-Processing Operations Order", "Source Image:Overlay ROI Median", "Source Image:Median Overlay Color", "Data Information:Gate Width", "Data Information:Nanotime Gate Separation", "Data Information:Macrotime Gate Separation", "Data Information:Gate Step", "Data Information:# Gates", "Data Information:Gate Image Exposure", "Data Information:Gate Image Integration", "Data Information:Gates to Skip", "Data Information:Gates to Keep", "Data Information:Define Gates to", "Data Information:Channel Name", "Data Information:Available Channel Names", "Data Information:Channel Arithmetic", "Data Information:Background File Subtraction", "Data Information:Background File", "Data Information:Background Scaling Factor", "Data Information:Background Pile-up Correction", "Data Information:Background Pixel Well Capacity", "Data Information:Laser Period", "Data Information:SYNC Period", "Data Information:Pile-up Correction", "Data Information:Pixel Well Capacity", "Data Information:Dataset Scaling Factor", "Fluorescence Decay_Decay Pre-Processing:Reverse Gates", "Fluorescence Decay_Decay Pre-Processing:Verbose Decay Pre-Processing", "Fluorescence Decay_Decay Pre-Processing:Use Decay Pre-Processing", "Fluorescence Decay_Decay Pre-Processing:Background Subtraction", "Fluorescence Decay_Decay Pre-Processing:Background Definition Range", "Fluorescence Decay_Decay Pre-Processing:Baseline Subtraction Method", "Fluorescence Decay_Decay Pre-Processing:Decay Pre-Processing Operations Order", "Fluorescence Decay_Decay Pre-Processing:Smoothing Parameter", "Fluorescence Decay_Decay Pre-Processing:Shift Decay", "Fluorescence Decay_Decay Pre-Processing:Decay Shift Parameters", "Fluorescence Decay_Decay Pre-Processing:Fold Decay", "Fluorescence Decay_Decay Pre-Processing:# Folds", "Fluorescence Decay_Decay Pre-Processing:1-Normalize Decay", "Fluorescence Decay_Decay Pre-Processing:[0-1]-Normalize Decay", "Fluorescence Decay_Decay Pre-Processing:Smoothen Decay", "Fluorescence Decay_Decay Pre-Processing:Extrapolate Decay", "Fluorescence Decay_Decay Pre-Processing:Use Periodicity", "Fluorescence Decay_Decay Pre-Processing:Use Cursors", "Fluorescence Decay_Decay Pre-Processing:Tail Fraction", "Fluorescence Decay_Decay Pre-Processing:Head Fraction", "Fluorescence Decay_Decay Pre-Processing:Additional Points", "Fluorescence Decay_Decay Pre-Processing:Straighten Decay", "Fluorescence Decay_Decay Pre-Processing:Constant Background", "Fluorescence Decay_Decay Pre-Processing:Pixel-Normalize Decay", "Fluorescence Decay_Advanced Analysis:Extract IRF instead of Decay", "Fluorescence Decay_Advanced Analysis:IRF Extraction Options", "Fluorescence Decay_Advanced Analysis:IRF Optimization Options", "Fluorescence Decay_Advanced Analysis:Square Pulse Options", "Fluorescence Decay_Advanced Analysis:IRF Order", "Fluorescence Decay_Advanced Analysis:IRF Time Constants", "Fluorescence Decay_Advanced Analysis:Wavelet Analysis Options", "Fluorescence Decay_Advanced Analysis:Average Lifetime Options", "Fluorescence Decay_Fit Options:Fit Options", "Fluorescence Decay_Fit Options:Use Legacy Fitting Approach", "Fluorescence Decay_Fit Options:Use Data Information Laser Period", "Fluorescence Decay_Fit Parameters:Displayed Fit Parameters", "Fluorescence Decay_Fit Parameters:Fit Parameter Constraints", "Fluorescence Decay_Fit Parameters:Export Tabulated Results", "Fluorescence Decay_Fit Parameters:MLE Baseline Offset Type", "Fluorescence Decay_Fit Parameters:MLE Baseline Offset", "Fluorescence Decay_Fit Parameters:Guess Parameter Names", "Fluorescence Decay_Fit Parameters:Guess Parameter Values", "Fluorescence Decay_Fit Parameters:Guess Parameters Options", "Fluorescence Decay_Fit Parameters:Optimal Offset Selection Criterion", "Fluorescence Decay_Styles:Show Last Decay Only", "Fluorescence Decay_Styles:Decay Graph Color Array", "Fluorescence Decay:Decay Graph Active", "Fluorescence Decay Statistics:Min Peak Value", "Fluorescence Decay Statistics:Reject Low Decay Peak Pixels", "Fluorescence Decay Statistics:Reject High Decay Peak Pixels", "Fluorescence Decay Statistics:Max Peak Value", "Time Traces:Use File Timestamp", "Time Traces:Time Step", "Time Traces:Use Intensity Correction File", "Time Traces:Intensity Correction File", "Phasor Plot:Phasor Plot Smoothing Options", "Phasor Plot:Phasor Plot Size", "Phasor Plot:Phasor Plot Graphics Options", "Phasor Plot:Cumulative Phasor Plot", "Phasor Plot:Use Phasor Brightness", "Phasor Plot:Blend Overlay with Phasor Background", "Phasor Plot:Save Phasor Plot", "Phasor Plot:Show References", "Phasor Plot:Phasor Ratio Decay Range", "Phasor Plot:Exponential Fading", "Phasor Plot:Phasor Ratio Reference Colors", "Phasor Plot:Reference Radius", "Phasor Plot:Show Color Map Vertices", "Phasor Plot:Phasor Plot Active", "Phasor Plot:Phasor Ratio Color Map Type", "Phasor Plot:Phasor Ratio Color Map", "Phasor Plot:Phasor Ratio Display Range", "Phasor Plot:Selected Image ROI(s)", "Phasor Plot:All Image ROIs", "Phasor Plot:Selected Phasor Plot ROI(s)", "Phasor Plot:All Phasor Plot ROIs", "Phasor Plot:Phasor Ratio Color-Coded Quantity", "Phasor Plot:Store Phasor Harmonics", "Phasor Plot:Draw Reference Segment", "Phasor Plot:User-Defined Quantity", "Phasor Plot:Color Scale High Color", "Phasor Plot:Color Scale Low Color", "Phasor Plot:Intensity-weighted Phasor Plot", "Phasor Graph:Phasor Frequency", "Phasor Graph:Phasor Ratio Type", "Phasor Graph:Pixel-level Phasor Computation", "Phasor Graph:Save Phasor Graph", "Phasor Graph:Phasor Graph Active", "Phasor Graph:Phasor SDV Options", "Phasor Graph:Intensity-weighted Phasor Graph", "Phasor Graph:Define Shortest Lifetime as", "Phasor Calibration:Use Backup Calibration if needed", "Phasor Calibration:Backup Calibration Type", "Phasor Calibration:Calibration Type", "Phasor Calibration:Calibration Lifetime", "Phasor Calibration:Calibration Map Algorithm", "Single-Exponential Phasor Locus (SEPL):Gate Parameters", "Single-Exponential Phasor Locus (SEPL):User-defined Gate", "Single-Exponential Phasor Locus (SEPL):User-defined IRF", "Single-Exponential Phasor Locus (SEPL):Phasor Parameters", "Single-Exponential Phasor Locus (SEPL):Decay & IRF Parameters", "Single-Exponential Phasor Locus (SEPL):Display Parameters", "Lifetime Analysis:Decay Analysis Parameters", "Lifetime Analysis:Lifetime Map Active", "Plugins:Python Settings", "Miscellaneous:Verbose Mode", "Miscellaneous:Beep after Script", "Miscellaneous:Saved Image File Format", "Miscellaneous:Exported Gate Image Settings", "Miscellaneous:Include Loading in Timing", "Miscellaneous:Verbose Settings Mode", "Miscellaneous:Histogram Options", "Miscellaneous:Beep on Error", "Miscellaneous:# Logical Processors Used", "Miscellaneous:ROI Description Max Characters", "Miscellaneous:Verbose Error Mode", "Miscellaneous:Transparent Mask Color"}
  T31 = typedef "Palette.lvlib/Image Palette Information.ctl" = cluster{"Palette Name [# Colors,int?,inv?]":string, "Palette Type":T32, "Palette Colors":u32[], "Interpolate?":bool}
  T32 = typedef "Image.lvlib/Image Display Palette Type.ctl" = u32
  T33 = typedef "AlliGator Globals, Variables & Constants.lvlib/AlliGator Variables List.ctl" = enum16{"---- GUI ----", "GUI:Initialization Status", "GUI:State Indicators Refnum", "GUI:Original AlliGator Menu Items", "GUI:Current Action Loop State", "GUI:Script in progress", "GUI:Playback", "GUI:Loop Playback", "GUI:Search ROI Used", "GUI:Search ROI", "Decay Graph Max Legend Size", "Intensity Graph Max Legend Size", "Decay Statistics Graph Max Legend Size", "Phasor Graph Max Legend Size", "Phasor Ratio Graph Max Legend Size", "Lifetime Graph Max Legend Size", "---- Files ----", "Files:Export Dataset Frames as Individual Files", "Files:Show Batch Export Help Balloons", "Files:Frames in Dataset", "Files:ptu File Frame Start Indices", "Files:Current Frame in Dataset", "Files:Current Frame Timestamp", "Files:Dataset Loaded", "Files:Dataset Metadata", "Files:Dataset Channel", "Files:Dataset Data Description", "Files:Background Dataset Metadata", "Files:Background Dataset Channel", "Files:Background Dataset Data Description", "Files:Background File Subtraction", "Files:Background File Path", "Files:Background File Pile-up Correction", "Files:Background File Pixel Well Capacity", "Files:Background File Scaling Factor", "Files:Current Dataset Load Settings", "Files:Dataset Path", "Files:ICCD-specific Information", "Files:Macrotime Gate Separation", "------ Python Plugins ------", "Python Plugins:Information", "Python Plugins:Python Session", "Python Plugins:Valid Python Session?", "---- Source Image ----", "Source Image:ROIs", "Source Image:Current ROI", "Source Image:ROI Event Refnum", "X_Source Image:Display Range", "X_Source Image:Palette Information", "X_Source Image:Type of Displayed Image", "X_Time Gate Slider", "Source Image:Palette List", "Source Image:Scale", "Source Image:ROI Overlay Color", "Source Image:Overlay to Erase", "Source Image:Is Displayed Image Accumulated", "Source Image:White Light Image Modified", "Source Image:Mask Image Modified", "---- Image Profile Window ----", "Image Profile:Window Event Refnum", "Image Profile:IntensityType", "Image Profile:Intensity Average Type", "Image Profile:Intensity-weighted SDV", "Image Profile:Box Profile Type", "Image Profile:Window Open", "Image Profile:Plotted Fit Parameter", "------ Phasor Graph -------", "Phasor Graph:Show Line", "---- Phasor Plot ---", "Phasor Plot:Parameters Changed", "Phasor Plot:FLI Dataset Modified since last Calculation", "Phasor Harmonics Data", "Selected Phasor Harmonics", "Phasor Harmonic Manager Event Refnum", "Phasor Plot:ROIs", "Phasor Plot:Current ROI", "Phasor Plot:ROI Event Refnum", "Phasor Plot:Image Reference Points", "Phasor Plot:Computed", "Phasor Plot:Palette Information", "Phasor Plot:Palette List", "Phasor Plot:Phasor Ratio Palette Information", "Phasor Plot:Phasor Ratio Palette List", "Phasor Plot:Image Scale", "Phasor Plot:Image Overlay to Erase", "Phasor Plot:Image Elements to Update", "Phasor Plot:Current Calculation Parameters", "Phasor Plot:Current Calibration Options", "Phasor Plot:Reset Cumulated Phasor Plot", "Phasor Plot:Reference 1", "Phasor Plot:Lifetime Reference 1", "Phasor Plot:Reference 1 Frequency", "Phasor Plot:Reference 2", "Phasor Plot:Lifetime Reference 2", "Phasor Plot:Reference 2 Frequency", "---- Decay Analysis ----", "Number of Selected Decays to Fit", "LS Fit Results", "LAR Fit Results", "BS Fit Results", "Last Decay Max - Min", "Best Fit Parameters", "Best Fit Parameter Names", "Actual Size X", "Actual Size Y", "Binning X", "Binning Y", "Actual # Gates", "Dataset Number", "Gates to...", "Gates Skipped", "Gates to keep", "Gate Step", "Gate Separation", "Reversed Gates", "Pile-up Correction", "Pixel Well Capacity", "Background Subtracted", "Background Subtraction Method", "Background Definition Range", "Background File (deprecated)", "Number of Dataset Accumulated", "Array of Accumulated Dataset Paths", "Do Averaged Datasets", "Destination File Path", "Process Plot Target", "Use 1/D as Phasor Frequency", "---- Decay Fit Parameter Map -----", "Decay Fit Parameter Map:Palette Information", "Decay Fit Parameter Map:Palette List", "Decay Fit Parameter Map:X Resolution", "Decay Fit Parameter Map:Y Resolution", "Decay Fit Parameter Map:Use Decay Fit Result Constraints", "Decay Fit Parameter Map:Decay Fit Result Constraints", "Decay Fit Parameter Map:Decay Fit Result Constraints Applied", "---- Parameter Map ----", "Parameter Map:Palette Information", "Parameter Map:Palette List", "------- Local Decay Window ---------", "Local Decay Graph Window:Event Refnum", "Local Decay Graph Window:Use normalized IRF for convolution", "----- Miscellaneous ----", "Misc:Skippable Dialog Windows Status"}
  T34 = enum16{"0", "1", "2", "3", "4", "5", "6", "7", "8", "9", "A", "B", "C", "D", "E", "F", "G", "H", "I", "J", "K", "L", "M", "N", "O", "P", "Q", "R", "S", "T", "U", "V", "W", "X", "Y", "Z", "F1", "F2", "F3", "F4", "F5", "F6", "F7", "F8", "F9", "F10", "F11", "F12", "F13", "F14", "F15", "ADD", "BACK", "BACKSLASH", "CAPITAL", "COMMA", "DECIMAL", "DELETE", "DIVIDE", "DOWN", "END", "EQUALS", "ESCAPE", "GRAVE (`)", "HOME", "INSERT", "LBRACKET", "LCONTROL", "LEFT", "L ALT", "LSHIFT", "LWIN", "MINUS", "MULTIPLY", "NEXT", "NUMLOCK", "NUMPAD_0", "NUMPAD_1", "NUMPAD_2", "NUMPAD_3", "NUMPAD_4", "NUMPAD_5", "NUMPAD_6", "NUMPAD_7", "NUMPAD_8", "NUMPAD_9", "PAUSE", "PERIOD", "PRIOR (PG UP)", "RBRACKET", "RCONTROL", "RETURN", "RIGHT", "R ALT", "RSHIFT", "RWIN", "SCROLL", "SEMICOLON", "SLASH", "SPACE", "SUBTRACT", "TAB", "UP", "ENTER (num pad)", "' (quote)"}
  T35 = typedef "Image.lvlib/Image Display Event.ctl" = cluster{"Item Tag":string, "Image Control Refnum":T36, "Coords":T37, "Item Path":string}
  T36 = typedef "Image.lvlib/Image Control Refnum.ctl" = refnum<vi>
  T37 = typedef "LVPoint32TypeDef.ctl" = cluster{"Horizontal":i32, "Vertical":i32}
  T38 = typedef "AlliGator Decay Fit Parameter Map.lvlib/AlliGator Decay Parameter Map Update Event Data.ctl" = cluster{"Parameter":T11, "Parameter changed":bool}
  T39 = typedef "XY Graph Add-Ons.lvlib/XY Graph Event.ctl" = cluster{"Item Tag":string, "XY Graph Refnum":refnum<vi>, "Coords":T37, "Item Path":string}
  T40 = typedef "Utilities.lvlib/Read-Write.ctl" = enum16{"Read", "Write"}
  T41 = typedef "XY Graph Add-Ons.lvlib/XY Graph Mouse Click Event Data.ctl" = cluster{"Multiplot XY Graph":T42, "Mouse Coordinates":T37}
  T42 = typedef "XY Graph Add-Ons.lvlib/XY Graph Refnum.ctl" = refnum<vi>
  T43 = typedef "AlliGator Parameter Map.lvlib/AlliGator Parameter Map Update Event Data.ctl" = cluster{"Parameter":u16, "Parameter changed":bool, "Map Set":u16}
  T44 = typedef "AlliGator ROIs.lvlib/AlliGator ROI Manager Actions.ctl" = enum16{"Undefined", "Delete Current ROI", "Delete All Unselected ROIs", "Delete Multiple ROIs", "Delete All ROIs", "Swap ROIs", "Insert ROI", "Update Current ROI Descriptor", "Rename Current ROI", "Store New ROI", "Store Multiple ROIs", "Select Next ROI", "Select Previous ROI", "Find Selected ROI", "Show All ROIs", "Update ROI Manager Window", "Merge All ROIs", "Unmerge ROI", "Set Selected ROI by ID"}
  T45 = typedef "AlliGator GUI.lvlib/AlliGator Image Mouse Up Event Data.ctl" = cluster{"Current ROI Tool":u32, "ROI Descriptor":T46, "Shift":bool, "Alt":bool, "Image Display Refnum":T36}
  T46 = typedef "Image.lvlib/Image ROI Descriptor.ctl" = cluster{"Global Rectangle":i32[], "Contours":T47[]}
  T47 = typedef "Image.lvlib/Image Contour Definition.ctl" = cluster{"Contour Type":T48, "ROI Type":T49, "Points":i32[]}
  T48 = typedef "Image.lvlib/Image Contour ID.ctl" = enum32{"External", "Internal"}
  T49 = typedef "Image.lvlib/Image ROI Type.ctl" = enum16{"No Selection", "Point", "Line", "Rectangle", "Oval", "Polygon", "Freehand Region", "Annulus", "Unused2", "Unused3", "Broken Line", "Freehand Line", "Rotated Rectangle"}
  T50 = typedef "AlliGator Parameter Map.lvlib/AlliGator Parameter Map Display Range Mouse Move Data.ctl" = cluster{"Parameter Map Set":u16, "Map Parameter":u16}
  T51 = typedef "Image.lvlib/Image Display User Event Data.ctl" = cluster{"Image Control Refnum":T36, "Coords":T37, "button info":cluster{"button 1":bool, "button 2":bool, "button 3":bool, "button 4":bool}, "keys pressed":enum16{"0", "1", "2", "3", "4", "5", "6", "7", "8", "9", "A", "B", "C", "D", "E", "F", "G", "H", "I", "J", "K", "L", "M", "N", "O", "P", "Q", "R", "S", "T", "U", "V", "W", "X", "Y", "Z", "F1", "F2", "F3", "F4", "F5", "F6", "F7", "F8", "F9", "F10", "F11", "F12", "F13", "F14", "F15", "ADD", "BACK", "BACKSLASH", "CAPITAL", "COMMA", "DECIMAL", "DELETE", "DIVIDE", "DOWN", "END", "EQUALS", "ESCAPE", "GRAVE (`)", "HOME", "INSERT", "LBRACKET", "LCONTROL", "LEFT", "L ALT", "LSHIFT", "LWIN", "MINUS", "MULTIPLY", "NEXT", "NUMLOCK", "NUMPAD_0", "NUMPAD_1", "NUMPAD_2", "NUMPAD_3", "NUMPAD_4", "NUMPAD_5", "NUMPAD_6", "NUMPAD_7", "NUMPAD_8", "NUMPAD_9", "PAUSE", "PERIOD", "PRIOR (PG UP)", "RBRACKET", "RCONTROL", "RETURN", "RIGHT", "R ALT", "RSHIFT", "RWIN", "SCROLL", "SEMICOLON", "SLASH", "SPACE", "SUBTRACT", "TAB", "UP", "ENTER (num pad)", "' (quote)"}[]}
  T52 = enum16{"0", "1", "2", "3", "4", "5", "6", "7", "8", "9", "A", "B", "C", "D", "E", "F", "G", "H", "I", "J", "K", "L", "M", "N", "O", "P", "Q", "R", "S", "T", "U", "V", "W", "X", "Y", "Z", "F1", "F2", "F3", "F4", "F5", "F6", "F7", "F8", "F9", "F10", "F11", "F12", "F13", "F14", "F15", "ADD", "BACK", "BACKSLASH", "CAPITAL", "COMMA", "DECIMAL", "DELETE", "DIVIDE", "DOWN", "END", "EQUALS", "ESCAPE", "GRAVE (`)", "HOME", "INSERT", "LBRACKET", "LCONTROL", "LEFT", "L ALT", "LSHIFT", "LWIN", "MINUS", "MULTIPLY", "NEXT", "NUMLOCK", "NUMPAD_0", "NUMPAD_1", "NUMPAD_2", "NUMPAD_3", "NUMPAD_4", "NUMPAD_5", "NUMPAD_6", "NUMPAD_7", "NUMPAD_8", "NUMPAD_9", "PAUSE", "PERIOD", "PRIOR (PG UP)", "RBRACKET", "RCONTROL", "RETURN", "RIGHT", "R ALT", "RSHIFT", "RWIN", "SCROLL", "SEMICOLON", "SLASH", "SPACE", "SUBTRACT", "TAB", "UP", "ENTER (num pad)", "' (quote)"}[]
  T53 = typedef "XY Graph Add-Ons.lvlib/New Plot Information.ctl" = cluster{"Multiplot XY Graph":refnum<vi>, "Plot Name":string, "Plot Scales":T54, "Plot Interpolation":T55, "Point Style":T56, "Plot Color":u32, "Plot Metadata":variant}
  T54 = typedef "XY Graph Add-Ons.lvlib/Plot Scales.ctl" = cluster{"X Scale":u32, "Y Scale":u32}
  T55 = typedef "Graphs.lvlib/LabVIEW Plot Interpolation.ctl" = enum16{"Point (.)", "Stepwise Right (--.)", "Line + Point (\\. /)", "Stepwise Left (.--)", "Stepwise Centered (-.-)", "Stepwise Vertical (|.|)", "Line (-)", "Use Previous Plot's Style"}
  T56 = typedef "Graphs.lvlib/Plot Point Style.ctl" = enum16{"not defined", "None", "Empty Circle", "Filled Circle", "Thick Circle", "Dotted Circle", "Empty Square", "Filled Square", "Thick Square", "Dotted Square", "Small Filled Square", "Dot", "Cross", "Tiny Cross", "Large X", "Small x", "Diamond", "Small Empty Square"}
  T57 = cluster{"Global Rectangle":i32[], "Contours":cluster{"Contour Type":u32, "ROI Type":u32, "Points":i32[]}[]}
  T58 = typedef "AlliGator Settings.lvlib/AlliGator Settings Window Messages.ctl" = enum16{"Idle", "Subscribe", "Unsubscribe", "Refresh Parameter", "Refresh All Parameters", "Quit"}
  T59 = typedef "AlliGator Phasor Plot Color Map.lvlib/AlliGator Phasor Color Map User Event List.ctl" = enum16{"Init", "Vertex Update", "Color Change"}
  T60 = cluster{"button 1":bool, "button 2":bool, "button 3":bool, "button 4":bool}
  T61 = typedef "Rich Text Box.lvlib/Text Formatting.ctl" = cluster{"Font":string, "Text Color":T62, "Background Color":T62, "Style":T63, "Font Size":dbl, "Alignment":T64}
  T62 = typedef "Rich Text Box.lvlib/Text Colors.ctl" = enum16{"Unchanged", "Black", "Blue", "Cyan", "Maroon", "Gray", "Violet", "Green", "Light Green", "Orange", "Yellow", "Magenta", "Red", "White"}
  T63 = typedef "Rich Text Box.lvlib/Text Style.ctl" = enum16{"Regular", "Bold", "Italic", "Underline", "Strikeout"}
  T64 = typedef "Rich Text Box.lvlib/Text Alignment.ctl" = enum16{"Left", "Right", "Center"}
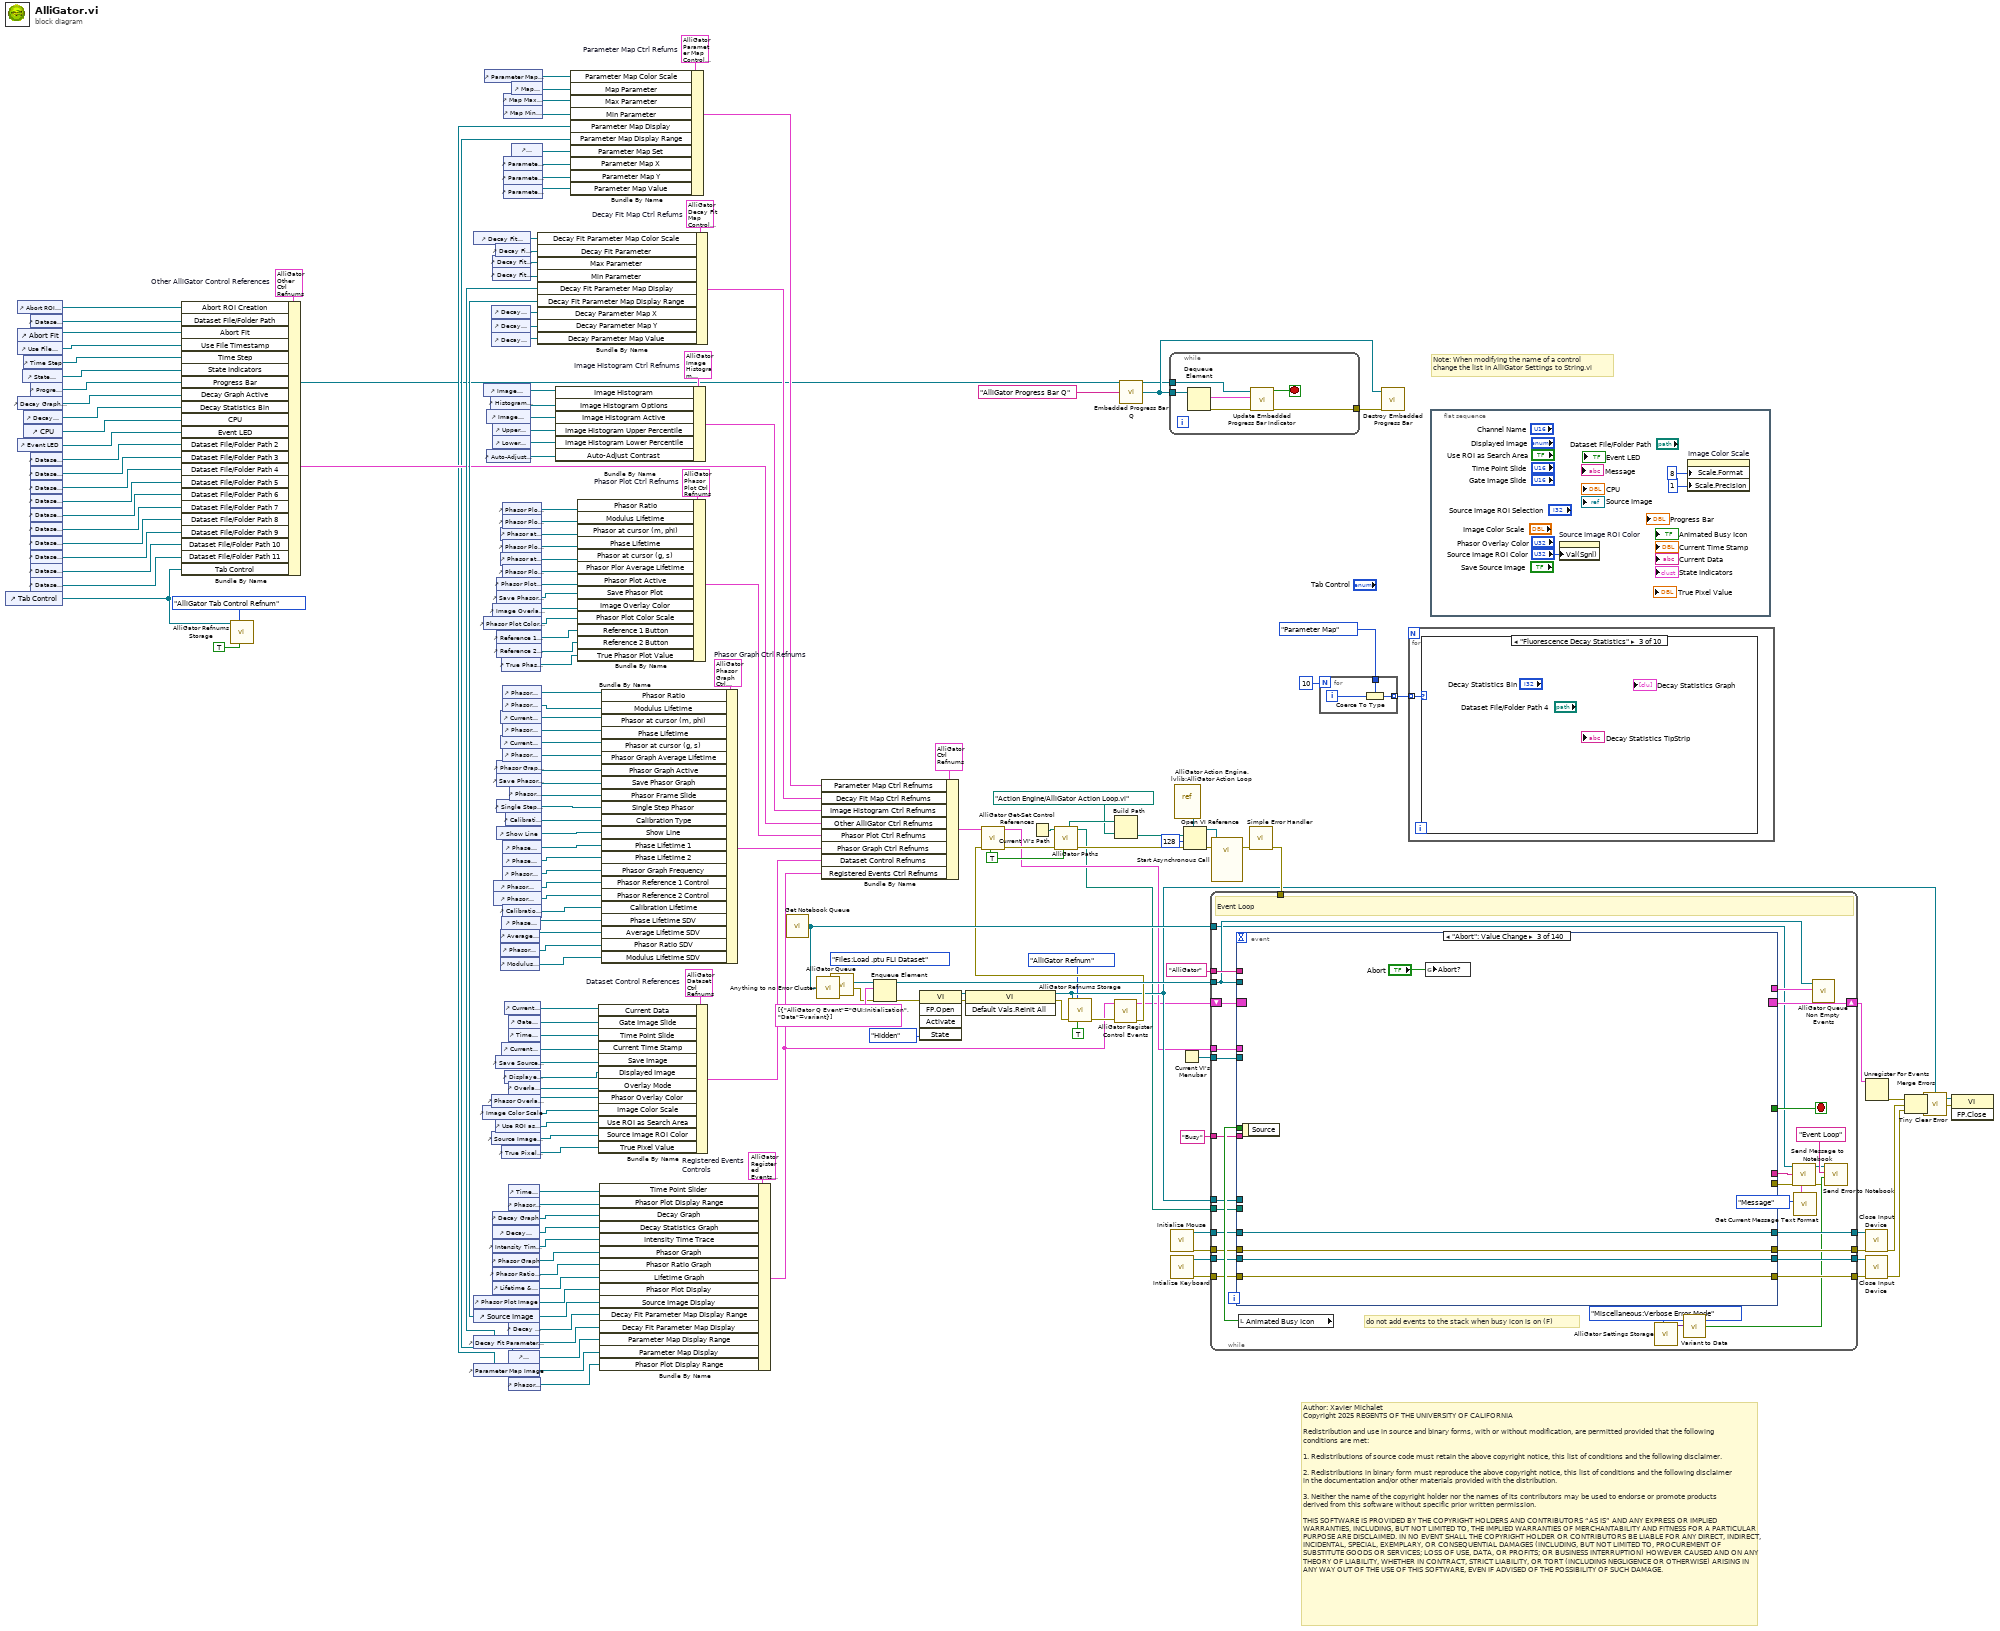
[diagram p0: block diagram]
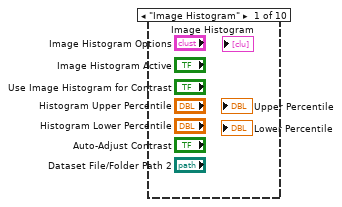
[diagram p2: hidden frame]
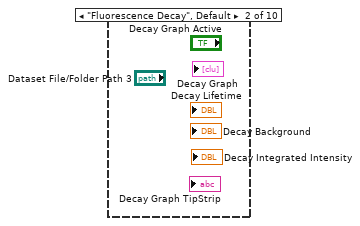
[diagram p3: hidden frame]
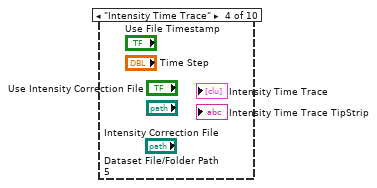
[diagram p4: hidden frame]
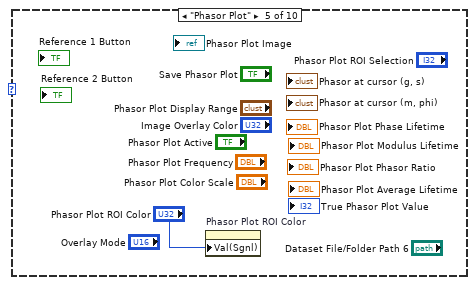
[diagram p5: hidden frame]
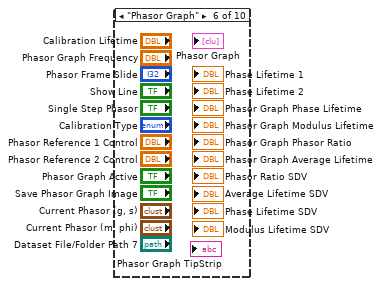
[diagram p6: hidden frame]
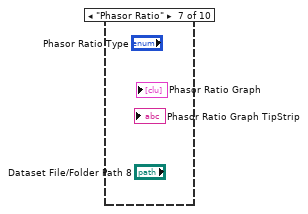
[diagram p7: hidden frame]
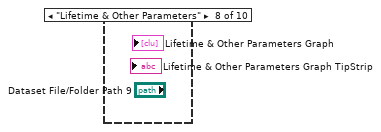
[diagram p8: hidden frame]
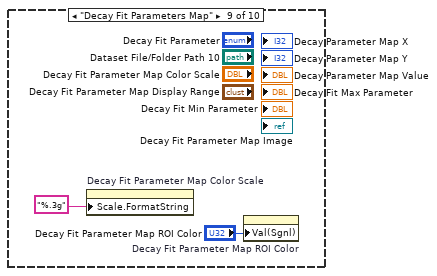
[diagram p9: hidden frame]
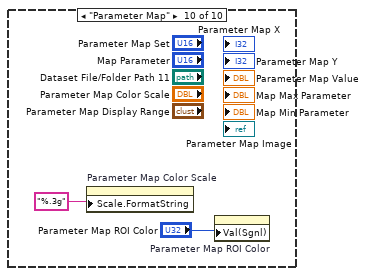
[diagram p10: hidden frame]
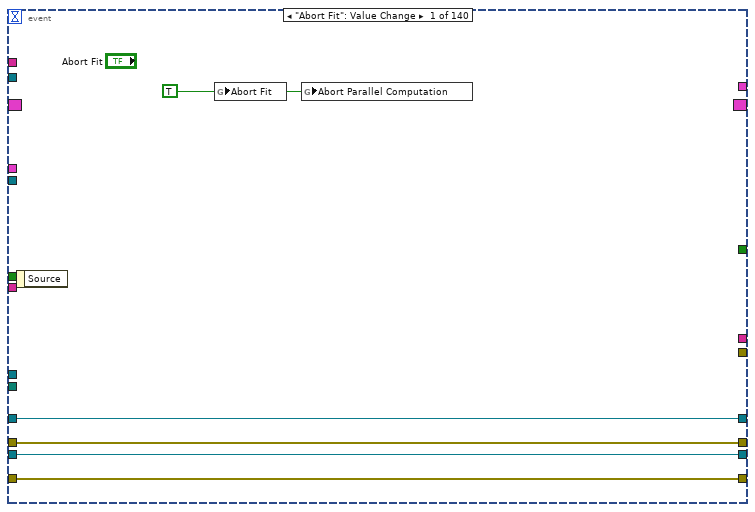
[diagram p11: hidden frame]
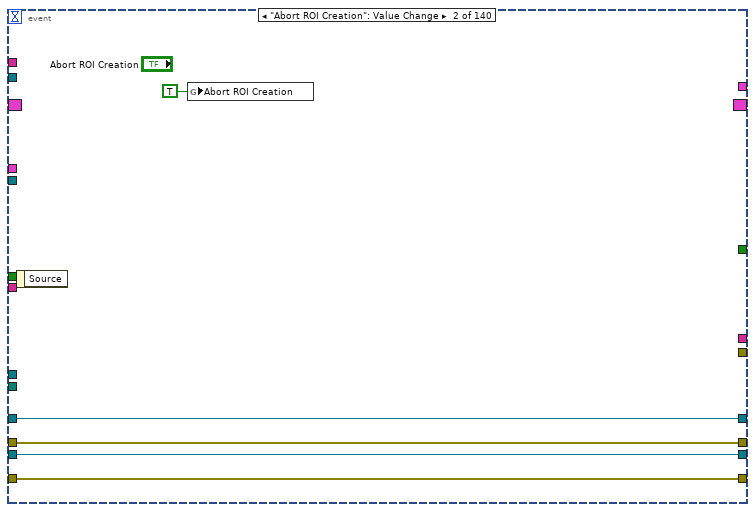
[diagram p12: hidden frame]
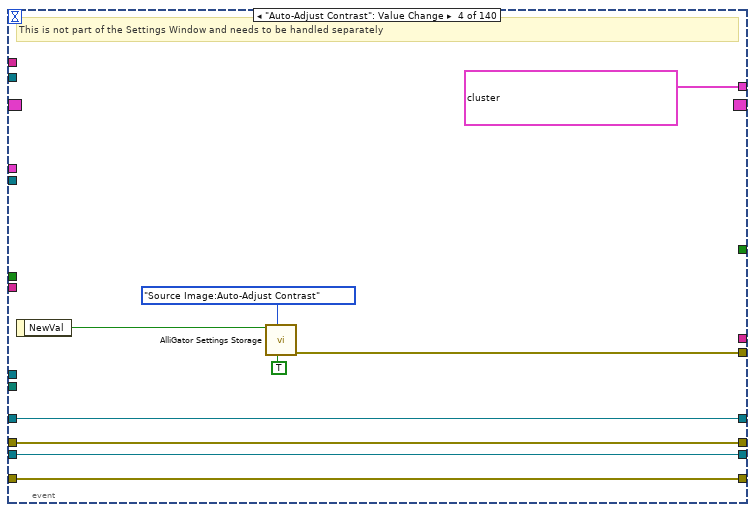
[diagram p13: hidden frame]
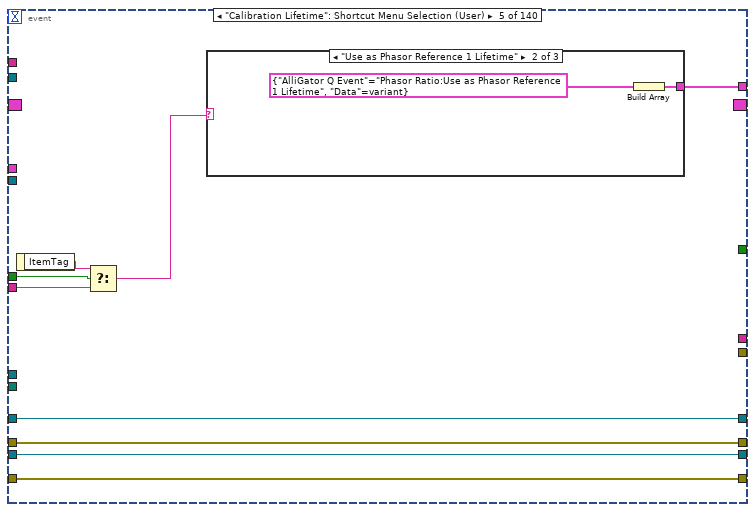
[diagram p14: hidden frame]
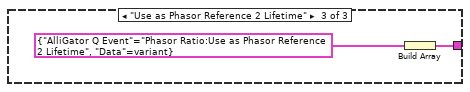
[diagram p16: hidden frame]
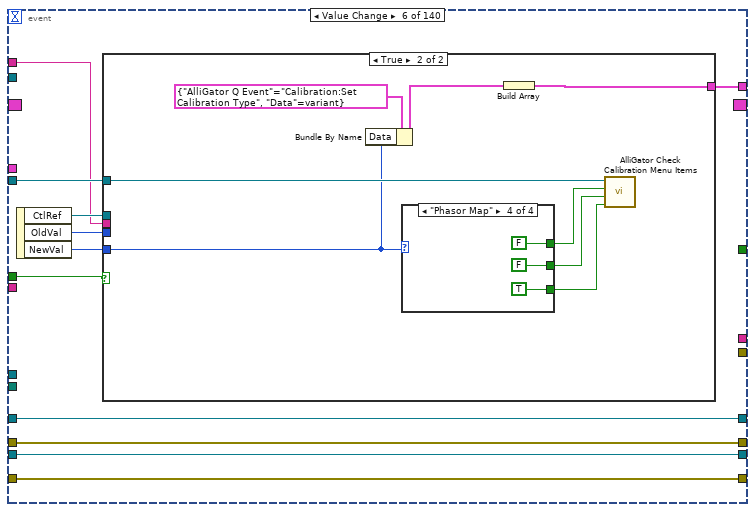
[diagram p17: hidden frame]
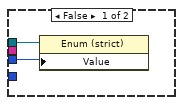
[diagram p18: hidden frame]
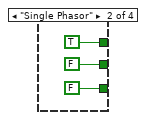
[diagram p20: hidden frame]
diagram:
  w28 = T14 {"Parameter Map Color Scale"=refnum, "Map Parameter"=refnum, "Max Parameter"=refnum, "Min Parameter"=refnum, "Parameter Map Display"=refnum, "Parameter Map Display Range"=refnum, "Parameter Map Set"=refnum, "Parameter Map X"=refnum, "Parameter Map Y"=refnum, "Parameter Map Value"=refnum}  # Parameter Map Ctrl Refums
  w20 = TRUE ("Get(F)/Set")
  w93 = T17 {"Decay Fit Parameter Map Color Scale"=refnum, "Decay Fit Parameter"=refnum, "Max Parameter"=refnum, "Min Parameter"=refnum, "Decay Fit Parameter Map Display"=refnum, "Decay Fit Parameter Map Display Range"=refnum, "Decay Parameter Map X"=refnum, "Decay Parameter Map Y"=refnum, "Decay Parameter Map Value"=refnum}  # Decay Fit Map Ctrl Refums
  w97 = T18 {"Image Histogram"=refnum, "Image Histogram Options"=refnum, "Image Histogram Active"=refnum, "Image Histogram Upper Percentile"=refnum, "Image Histogram Lower Percentile"=refnum, "Auto-Adjust Contrast"=refnum}  # Image Histogram Ctrl Refnums
  w116 = T19 {"Phasor Ratio"=refnum, "Modulus Lifetime"=refnum, "Phasor at cursor (m, phi)"=refnum, "Phase Lifetime"=refnum, "Phasor at cursor (g, s)"=refnum, "Phasor Graph Average Lifetime"=refnum, "Phasor Graph Active"=refnum, "Save Phasor Graph"=refnum, "Phasor Frame Slide"=refnum, "Single Step Phasor"=refnum, "Calibration Type"=refnum, "Show Line"=refnum, "Phase Lifetime 1"=refnum, "Phase Lifetime 2"=refnum, "Phasor Graph Frequency"=refnum, "Phasor Reference 1 Control"=refnum, "Phasor Reference 2 Control"=refnum, "Calibration Lifetime"=refnum, "Phase Lifetime SDV"=refnum, "Average Lifetime SDV"=refnum, "Phasor Ratio SDV"=refnum, "Modulus Lifetime SDV"=refnum}  # Phasor Graph Ctrl Refnums
  w117 = T20 {"Phasor Ratio"=refnum, "Modulus Lifetime"=refnum, "Phasor at cursor (m, phi)"=refnum, "Phase Lifetime"=refnum, "Phasor at cursor (g, s)"=refnum, "Phasor Plor Average Lifetime"=refnum, "Phasor Plot Active"=refnum, "Save Phasor Plot"=refnum, "Image Overlay Color"=refnum, "Phasor Plot Color Scale"=refnum, "Reference 1 Button"=refnum, "Reference 2 Button"=refnum, "True Phasor Plot Value"=refnum}  # Phasor Plot Ctrl Refnums
  (unwired) AlliGator_Q_Event."Files:Load .ptu FLI Dataset" ("AlliGator Q Event")
  w160 = T24 {"Time Point Slider"=refnum, "Phasor Plot Display Range"=refnum, "Decay Graph"=refnum, "Decay Statistics Graph"=refnum, "Intensity Time Trace"=refnum, "Phasor Graph"=refnum, "Phasor Ratio Graph"=refnum, "Lifetime Graph"=refnum, "Phasor Plot Display"=refnum, "Source Image Display"=refnum, "Decay Fit Parameter Map Display Range"=refnum, "Decay Fit Parameter Map Display"=refnum, "Parameter Map Display Range"=refnum, "Parameter Map Display"=refnum, "Phasor Plot Display Range"=refnum}  # Registered Events Controls
  w142 = T22 {"State Indicators"=refnum, " Progress Bar"=refnum, "Decay Graph Active"=refnum, "Decay Statistics Bin"=refnum, "Time Step"=refnum, "Use File Timestamp"=refnum, "Tab Control"=refnum, "CPU"=refnum, "Abort Fit"=refnum, "Dataset File/Folder Path"=refnum, "Abort ROI Creation"=refnum, "Event LED"=refnum, "Dataset File/Folder Path 2"=refnum, "Dataset File/Folder Path 3"=refnum, "Dataset File/Folder Path 4"=refnum, "Dataset File/Folder Path 5"=refnum, "Dataset File/Folder Path 6"=refnum, "Dataset File/Folder Path 7"=refnum, "Dataset File/Folder Path 8"=refnum, "Dataset File/Folder Path 9"=refnum, "Dataset File/Folder Path 10"=refnum, "Dataset File/Folder Path 11"=refnum}  # Other AlliGator Control References
  w168 = T23 {"Current Data"=refnum, "Gate Image Slide"=refnum, "Time Point Slide"=refnum, "Current Time Stamp"=refnum, "Save Image"=refnum, "Displayed Image"=refnum, "Overlay Mode"=refnum, "Phasor Overlay Color"=refnum, "Image Color Scale"=refnum, "Use ROI as Search Area"=refnum, "Source Image ROI Color"=refnum, "True Pixel Value"=refnum}  # Dataset Control References
  # "Author: Xavier Michalet\nCopyright 2025 REGENTS OF THE UNIVERSITY OF CALIFORNIA\n\nRedistribution and use in source and binary forms, with or without modification, are permitted provided that the following conditions are met:\n\n1. Redistributions of source code must retain the above copyright notice, this list of conditions and the following disclaimer.\n\n2. Redistributions in binary form must reproduce the above copyright notice, this list of conditions and the following disclaimer in the documentation and/or other materials provided with the distribution.\n\n3. Neither the name of the copyright holder nor the names of its contributors may be used to endorse or promote products derived from this software without specific prior written permission.\n\nTHIS SOFTWARE IS PROVIDED BY THE COPYRIGHT HOLDERS AND CONTRIBUTORS “AS IS” AND ANY EXPRESS OR IMPLIED WARRANTIES, INCLUDING, BUT NOT LIMITED TO, THE IMPLIED WARRANTIES OF MERCHANTABILITY AND FITNESS FOR A PARTICULAR PURPOSE ARE DISCLAIMED. IN NO EVENT SHALL THE COPYRIGHT HOLDER OR CONTRIBUTORS BE LIABLE FOR ANY DIRECT, INDIRECT, INCIDENTAL, SPECIAL, EXEMPLARY, OR CONSEQUENTIAL DAMAGES (INCLUDING, BUT NOT LIMITED TO, PROCUREMENT OF SUBSTITUTE GOODS OR SERVICES; LOSS OF USE, DATA, OR PROFITS; OR BUSINESS INTERRUPTION) HOWEVER CAUSED AND ON ANY THEORY OF LIABILITY, WHETHER IN CONTRACT, STRICT LIABILITY, OR TORT (INCLUDING NEGLIGENCE OR OTHERWISE) ARISING IN ANY WAY OUT OF THE USE OF THIS SOFTWARE, EVEN IF ADVISED OF THE POSSIBILITY OF SUCH DAMAGE."
  # "Note: When modifying the name of a control\nchange the list in AlliGator Settings to String.vi"
  n1 = control-ref of="Tab Control"() -> (w33:refnum<vi>)
  n2 = control-ref of="Abort ROI Creation"() -> (w102:refnum<vi>)
  n3 = control-ref of="Abort Fit"() -> (w105:refnum<vi>)
  n4 = control-ref of="Use File Timestamp"() -> (w118:refnum<vi>)
  n5 = control-ref of="Decay Graph Active"() -> (w126:refnum<vi>)
  n6 = control-ref of="Event LED"() -> (w61:refnum<vi>)
  n7 = control-ref of="State Indicators"() -> (w143:refnum<vi>)
  n8 = control-ref of="Time Step"() -> (w119:refnum<vi>)
  n9 = control-ref of="Decay Statistics Bin"() -> (w121:refnum<vi>)
  n10 = control-ref of="CPU"() -> (w106:refnum<vi>)
  n11 = control-ref of="Dataset File/Folder Path"() -> (w104:refnum<vi>)
  n12 = control-ref of="Progress Bar"() -> (w3:refnum<vi>)
  n13 = control-ref of="Dataset File/Folder Path 2"() -> (w45:refnum<vi>)
  n14 = control-ref of="Dataset File/Folder Path 3"() -> (w44:refnum<vi>)
  n15 = control-ref of="Dataset File/Folder Path 4"() -> (w43:refnum<vi>)
  n16 = control-ref of="Dataset File/Folder Path 5"() -> (w42:refnum<vi>)
  n17 = control-ref of="Dataset File/Folder Path 6"() -> (w41:refnum<vi>)
  n18 = control-ref of="Dataset File/Folder Path 7"() -> (w40:refnum<vi>)
  n19 = control-ref of="Dataset File/Folder Path 8"() -> (w39:refnum<vi>)
  n20 = control-ref of="Dataset File/Folder Path 9"() -> (w38:refnum<vi>)
  n21 = control-ref of="Dataset File/Folder Path 10"() -> (w37:refnum<vi>)
  n22 = control-ref of="Dataset File/Folder Path 11"() -> (w34:refnum<vi>)
  n23 = Bundle By Name(cluster=w142, "Abort ROI Creation"=w102, "Dataset File/Folder Path"=w104, "Abort Fit"=w105, "Use File Timestamp"=w118, "Time Step"=w119, "State Indicators"=w143, "Progress Bar"=w3, "Decay Graph Active"=w126, "Decay Statistics Bin"=w121, "CPU"=w106, "Event LED"=w61, "Dataset File/Folder Path 2"=w45, "Dataset File/Folder Path 3"=w44, "Dataset File/Folder Path 4"=w43, "Dataset File/Folder Path 5"=w42, "Dataset File/Folder Path 6"=w41, "Dataset File/Folder Path 7"=w40, "Dataset File/Folder Path 8"=w39, "Dataset File/Folder Path 9"=w38, "Dataset File/Folder Path 10"=w37, "Dataset File/Folder Path 11"=w34, "Tab Control"=w33) -> (w36:T22)
  n24 = call "AlliGator Refnums Storage.vi"("Get(F)/Set"=TRUE, "AlliGator Refnum List"=AlliGator_Refnums_List."AlliGator Tab Control Refnum", "Data in"=w33) -> ()  [unwired: 7 in, 2 out]
  n25 = control-ref of="Decay Fit Parameter Map Color Scale"() -> (w92:refnum<vi>)
  n26 = control-ref of="Phasor Plot Image"() -> (w173:refnum<vi>)
  n27 = control-ref of="Source Image"() -> (w172:refnum<vi>)
  n28 = control-ref of="Decay Fit Parameter Map Display"() -> (w90:refnum<vi>)
  n29 = control-ref of="Parameter Map Image"() -> (w25:refnum<vi>)
  n30 = control-ref of="Image Color Scale"() -> (w108:refnum<vi>)
  n31 = control-ref of="Image Histogram"() -> (w101:refnum<vi>)
  n32 = control-ref of="Phasor Plot Color Scale"() -> (w109:refnum<vi>)
  n33 = control-ref of="Parameter Map Color Scale"() -> (w29:refnum<vi>)
  n34 = control-ref of="Image Histogram Active"() -> (w100:refnum<vi>)
  n35 = control-ref of="Auto-Adjust Contrast"() -> (w57:refnum<vi>)
  n36 = control-ref of="Histogram Options"() -> (w54:refnum<vi>)
  n37 = control-ref of="Decay Parameter Map X"() -> (w6:refnum<vi>)
  n38 = control-ref of="Decay Parameter Map Y"() -> (w5:refnum<vi>)
  n39 = control-ref of="Decay Parameter Map Value"() -> (w4:refnum<vi>)
  n40 = control-ref of="Phasor Overlay Color"() -> (w122:refnum<vi>)
  n41 = control-ref of="Source Image ROI Color"() -> (w58:refnum<vi>)
  n42 = control-ref of="Decay Fit Max Parameter"() -> (w87:refnum<vi>)
  n43 = control-ref of="Decay Fit Min Parameter"() -> (w88:refnum<vi>)
  n44 = control-ref of="Upper Percentile"() -> (w99:refnum<vi>)
  n45 = control-ref of="Lower Percentile"() -> (w98:refnum<vi>)
  n46 = control-ref of="Image Overlay Color"() -> (w120:refnum<vi>)
  n47 = control-ref of="Decay Graph"() -> (w165:refnum<vi>)
  n48 = control-ref of="Decay Statistics Graph"() -> (w164:refnum<vi>)
  n49 = control-ref of="Intensity Time Trace"() -> (w163:refnum<vi>)
  n50 = control-ref of="Phasor Graph"() -> (w75:refnum<vi>)
  n51 = control-ref of="Phasor Ratio Graph"() -> (w162:refnum<vi>)
  n52 = control-ref of="Lifetime & Other Parameters Graph"() -> (w161:refnum<vi>)
  n53 = control-ref of="Phasor Reference 1 Control"() -> (w107:refnum<vi>)
  n54 = control-ref of="Phasor Reference 2 Control"() -> (w95:refnum<vi>)
  n55 = control-ref of="Decay Fit Parameter"() -> (w91:refnum<vi>)
  n56 = control-ref of="Save Source Image"() -> (w131:refnum<vi>)
  n57 = control-ref of="Use ROI as Search Area"() -> (w103:refnum<vi>)
  n58 = control-ref of="Phasor Plot Active"() -> (w134:refnum<vi>)
  n59 = control-ref of="Save Phasor Plot"() -> (w79:refnum<vi>)
  n60 = control-ref of="Reference 1 Button"() -> (w49:refnum<vi>)
  n61 = control-ref of="Reference 2 Button"() -> (w48:refnum<vi>)
  n62 = control-ref of="Phasor Graph Active"() -> (w133:refnum<vi>)
  n63 = control-ref of="Save Phasor Graph Image"() -> (w132:refnum<vi>)
  n64 = control-ref of="Single Step Phasor"() -> (w114:refnum<vi>)
  n65 = control-ref of="Show Line"() -> (w113:refnum<vi>)
  n66 = control-ref of="Phasor at cursor (m, phi)"() -> (w151:refnum<vi>)
  n67 = control-ref of="Phasor at cursor (g, s)"() -> (w149:refnum<vi>)
  n68 = control-ref of="Current Phasor (m, phi)"() -> (w146:refnum<vi>)
  n69 = control-ref of="Current Phasor (g, s)"() -> (w144:refnum<vi>)
  n70 = control-ref of="Average Lifetime SDV"() -> (w52:refnum<vi>)
  n71 = control-ref of="Phasor Ratio SDV"() -> (w51:refnum<vi>)
  n72 = control-ref of="Modulus Lifetime SDV"() -> (w50:refnum<vi>)
  n73 = control-ref of="True Phasor Plot Value"() -> (w1:refnum<vi>)
  n74 = control-ref of="Phase Lifetime SDV"() -> (w53:refnum<vi>)
  n75 = control-ref of="Current Time Stamp"() -> (w154:refnum<vi>)
  n76 = control-ref of="True Pixel Value"() -> (w2:refnum<vi>)
  n77 = control-ref of="Phasor Plot Phasor Ratio"() -> (w153:refnum<vi>)
  n78 = control-ref of="Phasor Plot Modulus Lifetime"() -> (w152:refnum<vi>)
  n79 = control-ref of="Phasor Plot Phase Lifetime"() -> (w150:refnum<vi>)
  n80 = control-ref of="Phasor Plot Average Lifetime"() -> (w135:refnum<vi>)
  n81 = control-ref of="Phasor Graph Phasor Ratio"() -> (w148:refnum<vi>)
  n82 = control-ref of="Phasor Graph Modulus Lifetime"() -> (w147:refnum<vi>)
  n83 = control-ref of="Phasor Graph Phase Lifetime"() -> (w145:refnum<vi>)
  n84 = control-ref of="Phasor Graph Average Lifetime"() -> (w136:refnum<vi>)
  n85 = control-ref of="Phase Lifetime 1"() -> (w112:refnum<vi>)
  n86 = control-ref of="Phase Lifetime 2"() -> (w111:refnum<vi>)
  n87 = control-ref of="Phasor Graph Frequency"() -> (w110:refnum<vi>)
  n88 = control-ref of="Calibration Lifetime"() -> (w94:refnum<vi>)
  n89 = control-ref of="Map Max Parameter"() -> (w32:refnum<vi>)
  n90 = control-ref of="Map Min Parameter"() -> (w31:refnum<vi>)
  n91 = control-ref of="Parameter Map X"() -> (w9:refnum<vi>)
  n92 = control-ref of="Parameter Map Y"() -> (w8:refnum<vi>)
  n93 = control-ref of="Parameter Map Value"() -> (w7:refnum<vi>)
  n94 = control-ref of="Current Data"() -> (w170:refnum<vi>)
  n95 = control-ref of="Displayed Image"() -> (w130:refnum<vi>)
  n96 = control-ref of="Calibration Type"() -> (w63:refnum<vi>)
  n97 = control-ref of="Time Point Slide"() -> (w167:refnum<vi>)
  n98 = control-ref of="Phasor Plot Display Range"() -> (w166:refnum<vi>)
  n99 = control-ref of="Decay Fit Parameter Map Display Range"() -> (w86:refnum<vi>)
  n100 = control-ref of="Parameter Map Display Range"() -> (w26:refnum<vi>)
  n101 = control-ref of="Gate Image Slide"() -> (w169:refnum<vi>)
  n102 = control-ref of="Time Point Slide"() -> (w155:refnum<vi>)
  n103 = control-ref of="Overlay Mode"() -> (w123:refnum<vi>)
  n104 = control-ref of="Phasor Plot Display Range"() -> (w19:refnum<vi>)
  n105 = control-ref of="Phasor Frame Slide"() -> (w115:refnum<vi>)
  n106 = control-ref of="Map Parameter"() -> (w30:refnum<vi>)
  n107 = control-ref of="Parameter Map Set"() -> (w27:refnum<vi>)
  n108 = Bundle By Name(cluster=w93, "Decay Fit Parameter Map Color Scale"=w92, "Decay Fit Parameter"=w91, "Max Parameter"=w87, "Min Parameter"=w88, "Decay Fit Parameter Map Display"=w90, "Decay Fit Parameter Map Display Range"=w86, "Decay Parameter Map X"=w6, "Decay Parameter Map Y"=w5, "Decay Parameter Map Value"=w4) -> (w89:T17)
  n109 = Bundle By Name(cluster=w97, "Image Histogram"=w101, "Image Histogram Options"=w54, "Image Histogram Active"=w100, "Image Histogram Upper Percentile"=w99, "Image Histogram Lower Percentile"=w98, "Auto-Adjust Contrast"=w57) -> (w96:T18)
  n110 = Bundle By Name(cluster=w28, "Parameter Map Color Scale"=w29, "Map Parameter"=w30, "Max Parameter"=w32, "Min Parameter"=w31, "Parameter Map Display"=w25, "Parameter Map Display Range"=w26, "Parameter Map Set"=w27, "Parameter Map X"=w9, "Parameter Map Y"=w8, "Parameter Map Value"=w7) -> (w24:T14)
  n111 = Bundle By Name(cluster=w117, "Phasor Ratio"=w153, "Modulus Lifetime"=w152, "Phasor at cursor (m, phi)"=w151, "Phase Lifetime"=w150, "Phasor at cursor (g, s)"=w149, "Phasor Plor Average Lifetime"=w135, "Phasor Plot Active"=w134, "Save Phasor Plot"=w79, "Image Overlay Color"=w120, "Phasor Plot Color Scale"=w109, "Reference 1 Button"=w49, "Reference 2 Button"=w48, "True Phasor Plot Value"=w1) -> (w129:T20)
  n112 = Bundle By Name(cluster=w168, "Current Data"=w170, "Gate Image Slide"=w169, "Time Point Slide"=w155, "Current Time Stamp"=w154, "Save Image"=w131, "Displayed Image"=w130, "Overlay Mode"=w123, "Phasor Overlay Color"=w122, "Image Color Scale"=w108, "Use ROI as Search Area"=w103, "Source Image ROI Color"=w58, "True Pixel Value"=w2) -> (w128:T23)
  n113 = Bundle By Name(cluster=w160, "Time Point Slider"=w167, "Phasor Plot Display Range"=w166, "Decay Graph"=w165, "Decay Statistics Graph"=w164, "Intensity Time Trace"=w163, "Phasor Graph"=w75, "Phasor Ratio Graph"=w162, "Lifetime Graph"=w161, "Phasor Plot Display"=w173, "Source Image Display"=w172, "Decay Fit Parameter Map Display Range"=w86, "Decay Fit Parameter Map Display"=w90, "Parameter Map Display Range"=w26, "Parameter Map Display"=w25, "Phasor Plot Display Range"=w19) -> (w12:T24)
  n114 = Bundle By Name(cluster=w116, "Phasor Ratio"=w148, "Modulus Lifetime"=w147, "Phasor at cursor (m, phi)"=w146, "Phase Lifetime"=w145, "Phasor at cursor (g, s)"=w144, "Phasor Graph Average Lifetime"=w136, "Phasor Graph Active"=w133, "Save Phasor Graph"=w132, "Phasor Frame Slide"=w115, "Single Step Phasor"=w114, "Calibration Type"=w63, "Show Line"=w113, "Phase Lifetime 1"=w112, "Phase Lifetime 2"=w111, "Phasor Graph Frequency"=w110, "Phasor Reference 1 Control"=w107, "Phasor Reference 2 Control"=w95, "Calibration Lifetime"=w94, "Phase Lifetime SDV"=w53, "Average Lifetime SDV"=w52, "Phasor Ratio SDV"=w51, "Modulus Lifetime SDV"=w50) -> (w64:T19)
  n115 = call "Get Notebook Queue.vi"() -> ("Notebook Queue"=w82:refnum<queue>)  [unwired: 9 in]
  n116 = call "Anything to no Error Cluster.vi"("Variant"=w82) -> ("Error Out"=w81:errorcluster)  [unwired: 8 in]
  n117 = Bundle By Name(cluster=T21 {"Other AlliGator Ctrl Refnums"={"State Indicators"=refnum, " Progress Bar"=refnum, "Decay Graph Active"=refnum, "Decay Statistics Bin"=refnum, "Time Step"=refnum, "Use File Timestamp"=refnum, "Tab Control"=refnum, "CPU"=refnum, "Abort Fit"=refnum, "Dataset File/Folder Path"=refnum, "Abort ROI Creation"=refnum, "Event LED"=refnum, "Dataset File/Folder Path 2"=refnum, "Dataset File/Folder Path 3"=refnum, "Dataset File/Folder Path 4"=refnum, "Dataset File/Folder Path 5"=refnum, "Dataset File/Folder Path 6"=refnum, "Dataset File/Folder Path 7"=refnum, "Dataset File/Folder Path 8"=refnum, "Dataset File/Folder Path 9"=refnum, "Dataset File/Folder Path 10"=refnum, "Dataset File/Folder Path 11"=refnum}, "Phasor Plot Ctrl Refnums"={"Phasor Ratio"=refnum, "Modulus Lifetime"=refnum, "Phasor at cursor (m, phi)"=refnum, "Phase Lifetime"=refnum, "Phasor at cursor (g, s)"=refnum, "Phasor Plor Average Lifetime"=refnum, "Phasor Plot Active"=refnum, "Save Phasor Plot"=refnum, "Image Overlay Color"=refnum, "Phasor Plot Color Scale"=refnum, "Reference 1 Button"=refnum, "Reference 2 Button"=refnum, "True Phasor Plot Value"=refnum}, "Phasor Graph Ctrl Refnums"={"Phasor Ratio"=refnum, "Modulus Lifetime"=refnum, "Phasor at cursor (m, phi)"=refnum, "Phase Lifetime"=refnum, "Phasor at cursor (g, s)"=refnum, "Phasor Graph Average Lifetime"=refnum, "Phasor Graph Active"=refnum, "Save Phasor Graph"=refnum, "Phasor Frame Slide"=refnum, "Single Step Phasor"=refnum, "Calibration Type"=refnum, "Show Line"=refnum, "Phase Lifetime 1"=refnum, "Phase Lifetime 2"=refnum, "Phasor Graph Frequency"=refnum, "Phasor Reference 1 Control"=refnum, "Phasor Reference 2 Control"=refnum, "Calibration Lifetime"=refnum, "Phase Lifetime SDV"=refnum, "Average Lifetime SDV"=refnum, "Phasor Ratio SDV"=refnum, "Modulus Lifetime SDV"=refnum}, "Dataset Control Refnums"={"Current Data"=refnum, "Gate Image Slide"=refnum, "Time Point Slide"=refnum, "Current Time Stamp"=refnum, "Save Image"=refnum, "Displayed Image"=refnum, "Overlay Mode"=refnum, "Phasor Overlay Color"=refnum, "Image Color Scale"=refnum, "Use ROI as Search Area"=refnum, "Source Image ROI Color"=refnum, "True Pixel Value"=refnum}, "Registered Events Ctrl Refnums"={"Time Point Slider"=refnum, "Phasor Plot Display Range"=refnum, "Decay Graph"=refnum, "Decay Statistics Graph"=refnum, "Intensity Time Trace"=refnum, "Phasor Graph"=refnum, "Phasor Ratio Graph"=refnum, "Lifetime Graph"=refnum, "Phasor Plot Display"=refnum, "Source Image Display"=refnum, "Decay Fit Parameter Map Display Range"=refnum, "Decay Fit Parameter Map Display"=refnum, "Parameter Map Display Range"=refnum, "Parameter Map Display"=refnum, "Phasor Plot Display Range"=refnum}, "Image Histogram Ctrl Refnums"={"Image Histogram"=refnum, "Image Histogram Options"=refnum, "Image Histogram Active"=refnum, "Image Histogram Upper Percentile"=refnum, "Image Histogram Lower Percentile"=refnum, "Auto-Adjust Contrast"=refnum}, "Decay Fit Map Ctrl Refnums"={"Decay Fit Parameter Map Color Scale"=refnum, "Decay Fit Parameter"=refnum, "Max Parameter"=refnum, "Min Parameter"=refnum, "Decay Fit Parameter Map Display"=refnum, "Decay Fit Parameter Map Display Range"=refnum, "Decay Parameter Map X"=refnum, "Decay Parameter Map Y"=refnum, "Decay Parameter Map Value"=refnum}, "Parameter Map Ctrl Refnums"={"Parameter Map Color Scale"=refnum, "Map Parameter"=refnum, "Max Parameter"=refnum, "Min Parameter"=refnum, "Parameter Map Display"=refnum, "Parameter Map Display Range"=refnum, "Parameter Map Set"=refnum, "Parameter Map X"=refnum, "Parameter Map Y"=refnum, "Parameter Map Value"=refnum}} ("AlliGator Ctrl Refnums"), "Parameter Map Ctrl Refnums"=w24, "Decay Fit Map Ctrl Refnums"=w89, "Image Histogram Ctrl Refnums"=w96, "Other AlliGator Ctrl Refnums"=w36, "Phasor Plot Ctrl Refnums"=w129, "Phasor Graph Ctrl Refnums"=w64, "Dataset Control Refnums"=w128, "Registered Events Ctrl Refnums"=w12) -> (w84:T21)
  n118 = call "AlliGator Queue.vi"("Error In"=w81) -> ("Error Out"=w171:errorcluster, "AlliGator Q"=w179:refnum<queue>)  [unwired: 7 in]
  n119 = Enqueue Element(queue=w179, element=T26[] [{"AlliGator Q Event"=enum."GUI:Initialization", "Data"=variant}] ("Named Q Element"), error in (no error)=w171) -> (queue out=w178:refnum<queue>, error out=w73:errorcluster)  [unwired: 1 in, 1 out]
  n120 = invoke class="VI" method="FP.Open"(error in=w73, "State"=T15."Hidden" ("Front Panel Window:State")) -> (reference out=w65:refnum<vi>, error out=w56:errorcluster)  [unwired: 3 in, 3 out]
  n121 = invoke class="VI" method="Default Vals.Reinit All"(reference=w65, error in=w56) -> (reference out=w18:refnum<vi>, error out=w17:errorcluster)  [unwired: 1 in, 1 out]
  n122 = Current VI's Path() -> (path=w70:path)
  n123 = call "AlliGator Refnums Storage.vi"("Get(F)/Set"=TRUE, "AlliGator Refnum List"=AlliGator_Refnums_List."AlliGator Refnum", "Error In"=w17, "Data in"=w18) -> ("Error Out"=w16:errorcluster)  [unwired: 6 in, 1 out]
  n124 = call "AlliGator Register Control Events.vi"("Error In"=w16, "AlliGator Control References"=w12) -> ("Error Out"=w46:errorcluster, "AlliGator Events Registration"=w10:T27)  [unwired: 8 in]
  n125 = call "AlliGator Get-Set Control References.vi"("Get(F)/Set"=w20, "Error In"=w46, "AlliGator Ctrl Refnums in"=w84) -> ("Error Out"=w47:errorcluster, "AlliGator Ctrl Refnums out"=w13:T21)  [unwired: 7 in]
  n126 = call "AlliGator Paths.vi"("Get(F)/Set"=w20, "error in (no error)"=w47, "AlliGator.vi Path"=w70) -> ("error out"=w68:errorcluster, "GUI Folder"=w11:path, "AlliGator Folder"=w23:path)  [unwired: 4 in, 2 out]
  n127 = Build Path(base path=w23, name or relative path=path "Action Engine/AlliGator Action Loop.vi") -> (appended path=w21:path)
  n128 = call "Embedded Progress Bar Q.vi"("Progress Bar Queue Name"="AlliGator Progress Bar Q") -> ("Progress Bar Queue"=w59:refnum<queue>)  [unwired: 6 in]
  n129 = while {
    tunnel: w59 -> [w185]
    tunnel: w3 -> [w183]
    tunnel: [w180] -> w60
    stop <- w181 stop-if-true
    n130 = Dequeue Element(queue=w185) -> (element=w184:T28, error out=w182:errorcluster)  [unwired: 2 in, 2 out]
    n131 = call "Update Embedded Progress Bar Indicator.vi"("Error In"=w182, "Progress Bar Event"=w184, "Progress Bar Refnum"=w183) -> ("Error Out"=w180:errorcluster, "Quit?"=w181:bool)  [unwired: 7 in]
  }
  n132 = call <vilib>:"Initialize Mouse.vi"() -> ("error out"=w158:errorcluster, "device ID"=w159:refnum<k1>)  [unwired: 10 in]
  n133 = call <vilib>:"Intialize Keyboard.vi"() -> ("error out"=w139:errorcluster, "device ID"=w140:refnum<k1>)  [unwired: 10 in]
  n134 = vi-ref "AlliGator Action Engine.lvlib:AlliGator Action Loop.vi"() -> (w69:refnum<vi>)
  n135 = Current VI's Menubar() -> (w176:refnum<k9>)
  n136 = Open VI Reference(type specifier VI Refnum (for type only)=w69, vi path=w21, options=128, error in (no error)=w68) -> (vi reference=w35:refnum<vi>, error out=w85:errorcluster)  [unwired: 2 in]
  n137 = call-by-ref "Start Asynchronous Call"(reference=w35, error in=w85) -> (error out=w62:errorcluster)  [unwired: 11 in, 2 out]
  n138 = while {
    tunnel: w178 -> [w190]
    tunnel: w176 -> [w216]
    shift-right: [w215] -> w175
    shift-left: w10 -> [w214]
    tunnel: "AlliGator" ("Sender") -> [w213]
    tunnel: w82 -> [w189]
    tunnel: w159 -> [w211]
    tunnel: w158 -> [w210]
    tunnel: [w209] -> w157
    tunnel: [w208] -> w156
    tunnel: w140 -> [w207]
    tunnel: w139 -> [w206]
    tunnel: [w205] -> w138
    tunnel: [w204] -> w137
    tunnel: w62 -> [_]
    tunnel: w18 -> [w199]
    tunnel: "Busy" ("t") -> [w191]
    tunnel: w13 -> [w188]
    tunnel: w11 -> [w187]
    stop <- w192 stop-if-true
    # "do not add events to the stack when busy icon is on (F)"
    # "Event Loop"
    n139 = local read "Animated Busy Icon"() -> (w212:bool)
    n140 = event shown="[2] \"Abort\": Value Change" {
      selector: w214 -> [_ _ _ _ _ _ _ _ _ _ _ _ _ _ _ _ _ _ _ _ _ _ _ _ _ _ _ _ _ _ _ _ _ _ _ _ _ _ _ _ _ _ _ _ _ _ _ _ _ _ _ _ _ _ _ _ _ _ _ _ _ _ _ _ _ _ _ _ _ _ _ _ _ _ _ _ _ _ _ _ _ _ w1509 w1526 _ _ w1574 w1585 w1591 w1606 w1614 _ w1632 w1640 _ w1658 w1666 _ w1684 w1692 _ _ _ w1768 w1785 _ _ w1833 w1844 w1850 w1874 w1880 w1899 w1904 w1912 _ w1936 w1964 w1981 _ w2058 w2098 w2109 w2115 w2128 w2136 _ w2158 w2186 w2203 _ w2269 w2297 _ w2333 _ _ _ _ _]
      dyn-events: [_ _ _ _ _ _ _ _ _ _ _ _ _ _ _ _ _ _ _ _ _ _ _ _ _ _ _ _ _ _ _ _ _ _ _ _ _ _ _ _ _ _ _ _ _ _ _ _ _ _ _ _ _ _ _ _ _ _ _ _ _ _ _ _ _ _ _ _ _ _ _ _ _ _ _ _ _ _ _ _ _ _ w1510 w1527 _ _ w1575 w1586 w1591 w1604 w1612 _ w1630 w1638 _ w1656 w1664 _ w1682 w1690 _ _ _ w1769 w1786 _ _ w1834 w1845 w1850 w1875 w1880 w1900 w1902 w1910 _ w1935 w1965 w1982 _ w2057 w2099 w2110 w2115 w2126 w2134 _ w2159 w2187 w2204 _ w2268 w2298 _ w2334 _ _ _ _ _] -> w215
      timeout: _ -> [_ _ _ _ _ _ _ _ _ _ _ _ _ _ _ _ _ _ _ _ _ _ _ _ _ _ _ _ _ _ _ _ _ _ _ _ _ _ _ _ _ _ _ _ _ _ _ _ _ _ _ _ _ _ _ _ _ _ _ _ _ _ _ _ _ _ _ _ _ _ _ _ _ _ _ _ _ _ _ _ _ _ _ _ _ _ _ _ _ _ _ _ _ _ _ _ _ _ _ _ _ _ _ _ _ _ _ _ _ _ _ _ _ _ _ _ _ _ _ _ _ _ _ _ _ _ _ _ _ _ _ _ _ _ _ _ _ _ _ _]
      tunnel: [_ _ _ _ _ _ _ _ _ _ _ _ _ _ _ _ _ _ _ _ _ _ _ _ _ _ _ _ _ _ _ _ _ _ _ _ _ _ _ _ _ _ _ _ _ _ _ _ _ _ _ _ _ _ _ _ _ _ _ _ _ _ _ _ _ _ _ _ _ _ _ _ _ _ _ _ _ _ _ _ _ _ _ _ _ _ _ _ _ _ _ _ _ _ _ _ _ _ _ _ _ _ _ _ _ _ _ _ _ _ _ _ _ _ _ _ _ _ _ _ _ _ _ _ _ _ _ _ _ _ _ _ _ _ _ _ w2381 _ _ w2407] -> w192
      tunnel: w190 -> [_ _ _ _ _ _ _ _ _ _ _ _ _ _ _ _ _ _ _ _ _ _ _ _ _ _ _ _ _ _ _ _ _ _ _ _ _ _ _ _ _ _ _ _ _ _ _ _ _ _ _ _ _ _ _ _ _ _ _ w1148 w1165 _ w1186 w1200 w1209 _ _ _ _ _ _ _ _ _ _ _ _ _ _ _ _ w1495 _ _ _ _ _ _ _ _ _ _ _ _ _ _ _ _ _ _ _ _ _ _ _ _ _ _ _ _ _ _ _ _ _ _ _ _ _ _ _ _ _ _ _ _ _ _ _ _ _ _ _ _ _ _ _ _ _ _]
      tunnel: w216 -> [_ _ _ _ _ w264 _ _ _ _ _ _ _ _ _ _ _ _ _ _ _ _ _ _ _ _ _ _ _ _ _ _ _ _ _ _ _ _ _ _ _ _ _ _ _ _ _ _ _ _ _ _ _ _ _ _ _ _ _ _ _ _ _ _ _ _ _ _ _ _ _ _ _ _ _ _ _ _ _ _ _ _ _ _ _ _ _ _ _ _ _ _ _ _ _ _ _ _ _ _ _ _ _ _ _ _ _ _ _ _ _ _ _ _ _ _ _ _ _ _ _ _ _ _ _ _ _ _ _ _ _ _ _ _ _ _ _ _ _ _]
      tunnel: w213 -> [_ _ _ _ _ w261 _ _ _ _ _ _ _ _ _ _ _ _ _ _ _ _ _ _ _ _ _ _ _ _ _ _ _ _ w625 _ _ _ _ _ _ _ _ _ _ w851 _ _ _ _ _ _ _ _ _ _ _ _ _ _ _ _ _ _ _ _ _ _ _ _ w1264 _ _ _ _ _ _ _ w1431 _ w1464 _ _ _ _ _ _ _ _ _ _ _ _ _ _ _ _ _ _ _ _ w1713 _ _ _ _ _ _ _ _ _ _ _ _ _ _ _ _ _ _ _ _ _ _ _ _ _ _ _ _ _ _ _ _ _ _ _ _ _ w2413]
      tunnel: w212 -> [_ _ _ _ w249 w260 _ _ w301 _ _ w320 w330 w337 w353 w360 w366 _ _ w410 _ w464 _ w484 w508 w519 w534 w549 w556 _ w580 _ w596 _ w623 _ w676 w720 w735 w742 _ w772 w810 w826 _ _ _ w930 w947 w961 _ _ _ w1006 _ w1047 _ _ w1109 w1146 w1163 w1173 w1185 w1199 w1208 _ _ w1236 w1244 w1252 w1262 w1284 _ w1313 _ _ w1373 w1411 _ w1444 w1461 w1493 w1508 w1525 w1541 w1553 _ _ w1594 _ _ _ _ _ _ _ _ _ _ _ _ _ w1756 w1767 w1784 w1800 w1812 _ _ w1853 _ w1883 _ _ _ _ w1927 w1957 w1980 w1994 w2060 _ _ w2118 _ _ _ w2152 w2179 w2202 w2220 w2262 w2296 w2314 w2332 w2354 w2378 _ _ w2414]
      tunnel: w191 -> [_ _ _ _ w246 _ _ _ _ _ _ _ w327 _ w351 _ _ _ _ _ _ _ _ _ _ _ _ _ _ _ _ _ _ _ _ _ w674 _ _ _ _ _ _ _ _ _ _ _ _ _ _ _ _ _ _ _ _ _ w1107 _ _ _ _ _ _ _ _ _ _ _ _ _ _ _ _ _ _ _ _ _ _ _ _ _ _ _ _ _ _ _ _ _ _ _ _ _ _ _ _ _ _ _ _ _ _ _ _ _ _ _ _ _ _ _ _ _ _ _ _ _ _ _ _ _ _ _ _ _ _ _ _ _ _ _ _ _ w2391 _ _ _]
      tunnel: w211 -> [w221 w225 w231 w237 w245 w258 w288 w294 w300 w307 w313 w319 w326 w336 w350 w359 w371 w380 w393 w420 w457 w463 w477 w500 w505 w516 w531 w548 w555 w566 w579 w587 w595 w608 w622 w657 w673 w719 w734 w741 w755 w782 w815 w823 w838 w853 w914 w935 w946 w963 w981 w990 w997 w1005 w1020 w1050 w1088 w1095 w1106 w1143 w1160 w1178 w1184 w1198 w1207 w1222 w1229 w1235 w1243 w1251 w1260 w1281 w1305 w1310 w1335 w1348 w1376 w1409 w1428 w1441 w1459 w1490 w1506 w1523 w1537 w1549 w1571 w1582 w1593 w1611 w1620 w1628 w1637 w1646 w1654 w1663 w1672 w1680 w1689 w1698 w1706 w1712 w1755 w1765 w1782 w1796 w1808 w1830 w1841 w1852 w1869 w1882 w1896 w1909 w1918 w1926 w1932 w1962 w1978 w2001 w2055 w2095 w2106 w2117 w2133 w2142 w2150 w2156 w2184 w2200 w2223 w2267 w2294 w2313 w2330 w2353 w2390 w2397 w2406 w2412]
      tunnel: w210 -> [w220 w224 w230 w236 w244 w257 w287 w293 w299 w306 w312 w318 w325 w335 w349 w358 w370 w379 w392 w419 w456 w462 w476 w499 w504 w515 w530 w547 w554 w565 w578 w586 w594 w607 w621 w656 w672 w718 w733 w740 w754 w781 w814 w822 w837 w852 w913 w934 w945 w962 w980 w989 w996 w1004 w1019 w1049 w1087 w1094 w1105 w1142 w1159 w1177 w1183 w1197 w1206 w1221 w1228 w1234 w1242 w1250 w1259 w1280 w1304 w1309 w1334 w1347 w1375 w1408 w1427 w1440 w1458 w1489 w1505 w1522 w1536 w1548 w1570 w1581 w1592 w1610 w1619 w1627 w1636 w1645 w1653 w1662 w1671 w1679 w1688 w1697 w1705 w1711 w1754 w1764 w1781 w1795 w1807 w1829 w1840 w1851 w1868 w1881 w1895 w1908 w1917 w1925 w1931 w1961 w1977 w2002 w2054 w2094 w2105 w2116 w2132 w2141 w2149 w2155 w2183 w2199 w2222 w2266 w2293 w2312 w2329 w2352 w2389 w2396 w2405 w2411]
      tunnel: [w221 w225 w231 w237 w245 w258 w288 w294 w300 w307 w313 w319 w326 w336 w350 w359 w371 w380 w393 w420 w457 w463 w477 w500 w505 w516 w531 w548 w555 w566 w579 w587 w595 w608 w622 w657 w673 w719 w734 w741 w755 w782 w815 w823 w838 w853 w914 w935 w946 w963 w981 w990 w997 w1005 w1020 w1050 w1088 w1095 w1106 w1143 w1160 w1178 w1184 w1198 w1207 w1222 w1229 w1235 w1243 w1251 w1260 w1281 w1305 w1310 w1335 w1348 w1376 w1409 w1428 w1441 w1459 w1490 w1506 w1523 w1537 w1549 w1571 w1582 w1593 w1611 w1620 w1628 w1637 w1646 w1654 w1663 w1672 w1680 w1689 w1698 w1706 w1712 w1755 w1765 w1782 w1796 w1808 w1830 w1841 w1852 w1869 w1882 w1896 w1909 w1918 w1926 w1932 w1962 w1978 w2000 w2055 w2095 w2106 w2117 w2133 w2142 w2150 w2156 w2184 w2200 w2223 w2267 w2294 w2313 w2330 w2353 w2390 w2397 w2406 w2412] -> w209
      tunnel: [w220 w224 w230 w236 w244 w257 w287 w293 w299 w306 w312 w318 w325 w335 w349 w358 w370 w379 w392 w419 w456 w462 w476 w499 w504 w515 w530 w547 w554 w565 w578 w586 w594 w607 w621 w656 w672 w718 w733 w740 w754 w781 w814 w822 w837 w852 w913 w934 w945 w962 w980 w989 w996 w1004 w1019 w1049 w1087 w1094 w1105 w1142 w1159 w1177 w1183 w1197 w1206 w1221 w1228 w1234 w1242 w1250 w1259 w1280 w1304 w1309 w1334 w1347 w1375 w1408 w1427 w1440 w1458 w1489 w1505 w1522 w1536 w1548 w1570 w1581 w1592 w1610 w1619 w1627 w1636 w1645 w1653 w1662 w1671 w1679 w1688 w1697 w1705 w1711 w1754 w1764 w1781 w1795 w1807 w1829 w1840 w1851 w1868 w1881 w1895 w1908 w1917 w1925 w1931 w1961 w1977 w1999 w2054 w2094 w2105 w2116 w2132 w2141 w2149 w2155 w2183 w2199 w2222 w2266 w2293 w2312 w2329 w2352 w2389 w2396 w2405 w2411] -> w208
      tunnel: [_ _ _ w233 _ _ w284 w290 _ w303 w309 _ _ _ _ _ _ _ w382 w408 _ _ w473 w482 _ _ _ _ _ w562 _ w583 _ _ w618 w651 _ _ _ _ w744 w770 _ _ w834 w845 w910 _ _ w950 w977 w985 _ _ w1013 w1039 _ _ _ _ _ _ _ _ _ w1218 w1225 _ _ _ w1256 _ _ _ _ w1338 w1364 w1405 w1434 w1437 w1455 _ w1502 w1519 _ _ w1565 w1576 _ _ _ _ _ _ _ _ _ _ _ _ _ w1710 _ w1761 w1778 _ _ w1824 w1835 _ w1865 _ w1890 _ _ _ w1930 w1958 w1974 _ w2052 w2090 w2100 _ _ _ _ w2151 w2180 w2196 _ w2259 w2290 _ w2326 w2349 w2375 _ _ _] -> w196
      tunnel: w207 -> [w218 w223 w229 w235 w243 w256 w286 w292 w298 w305 w311 w317 w324 w334 w348 w357 w368 w377 w391 w414 w454 w460 w475 w494 w503 w514 w529 w546 w553 w564 w577 w585 w592 w610 w620 w655 w671 w717 w732 w739 w753 w776 w812 w821 w836 w849 w912 w933 w944 w955 w979 w988 w995 w1003 w1018 w1044 w1085 w1092 w1104 w1141 w1158 w1175 w1182 w1196 w1205 w1220 w1227 w1233 w1241 w1249 w1258 w1279 w1302 w1308 w1333 w1346 w1370 w1407 w1426 w1439 w1457 w1488 w1504 w1521 w1540 w1552 w1567 w1578 w1590 w1608 w1617 w1625 w1634 w1643 w1651 w1660 w1669 w1677 w1686 w1695 w1703 w1709 w1753 w1763 w1780 w1799 w1811 w1826 w1837 w1849 w1867 w1879 w1892 w1906 w1915 w1923 w1929 w1960 w1976 w1995 w2051 w2092 w2102 w2114 w2130 w2139 w2147 w2154 w2182 w2198 w2216 w2265 w2292 w2310 w2328 w2351 w2387 w2394 w2403 w2410]
      tunnel: w206 -> [w217 w222 w228 w234 w242 w255 w285 w291 w297 w304 w310 w316 w323 w333 w347 w356 w369 w378 w390 w415 w455 w459 w474 w492 w502 w513 w528 w545 w552 w563 w576 w584 w593 w609 w619 w654 w670 w716 w731 w738 w752 w777 w813 w820 w835 w848 w911 w932 w943 w956 w978 w987 w994 w1002 w1017 w1045 w1086 w1093 w1103 w1140 w1157 w1176 w1181 w1195 w1204 w1219 w1226 w1232 w1240 w1248 w1257 w1278 w1303 w1307 w1332 w1345 w1368 w1406 w1425 w1438 w1456 w1487 w1503 w1520 w1539 w1551 w1566 w1577 w1589 w1609 w1618 w1626 w1635 w1644 w1652 w1661 w1670 w1678 w1687 w1696 w1704 w1708 w1752 w1762 w1779 w1798 w1810 w1825 w1836 w1848 w1866 w1878 w1891 w1907 w1916 w1924 w1928 w1959 w1975 w1997 w2050 w2091 w2101 w2113 w2131 w2140 w2148 w2153 w2181 w2197 w2219 w2264 w2291 w2309 w2327 w2350 w2386 w2395 w2404 w2409]
      tunnel: [w217 w222 w228 w234 w242 w255 w285 w291 w297 w304 w310 w316 w323 w333 w347 w356 w369 w378 w390 w413 w455 w459 w474 w493 w502 w513 w528 w545 w552 w563 w576 w584 w593 w609 w619 w654 w670 w716 w731 w738 w752 w775 w813 w820 w835 w848 w911 w932 w943 w953 w978 w987 w994 w1002 w1017 w1041 w1086 w1093 w1103 w1140 w1157 w1176 w1181 w1195 w1204 w1219 w1226 w1232 w1240 w1248 w1257 w1278 w1303 w1307 w1332 w1345 w1369 w1406 w1425 w1438 w1456 w1487 w1503 w1520 w1539 w1551 w1566 w1577 w1589 w1609 w1618 w1626 w1635 w1644 w1652 w1661 w1670 w1678 w1687 w1696 w1704 w1708 w1752 w1762 w1779 w1798 w1810 w1825 w1836 w1848 w1866 w1878 w1891 w1907 w1916 w1924 w1928 w1959 w1975 w1998 w2050 w2091 w2101 w2113 w2131 w2140 w2148 w2153 w2181 w2197 w2218 w2264 w2291 w2309 w2327 w2350 w2385 w2395 w2404 w2409] -> w205
      tunnel: [w218 w223 w229 w235 w243 w256 w286 w292 w298 w305 w311 w317 w324 w334 w348 w357 w368 w377 w391 w412 w454 w460 w475 w495 w503 w514 w529 w546 w553 w564 w577 w585 w592 w610 w620 w655 w671 w717 w732 w739 w753 w774 w812 w821 w836 w849 w912 w933 w944 w954 w979 w988 w995 w1003 w1018 w1043 w1085 w1092 w1104 w1141 w1158 w1175 w1182 w1196 w1205 w1220 w1227 w1233 w1241 w1249 w1258 w1279 w1302 w1308 w1333 w1346 w1371 w1407 w1426 w1439 w1457 w1488 w1504 w1521 w1540 w1552 w1567 w1578 w1590 w1608 w1617 w1625 w1634 w1643 w1651 w1660 w1669 w1677 w1686 w1695 w1703 w1709 w1753 w1763 w1780 w1799 w1811 w1826 w1837 w1849 w1867 w1879 w1892 w1906 w1915 w1923 w1929 w1960 w1976 w1996 w2051 w2092 w2102 w2114 w2130 w2139 w2147 w2154 w2182 w2198 w2217 w2265 w2292 w2310 w2328 w2351 w2384 w2394 w2403 w2410] -> w204
      tunnel: w199 -> [_ _ _ _ _ _ _ _ _ _ _ _ _ _ _ _ _ _ _ _ _ _ _ _ _ _ _ _ _ _ _ _ _ _ _ _ _ _ _ _ _ _ _ _ _ _ _ _ _ _ _ _ _ _ _ _ _ _ _ _ _ _ _ _ _ _ _ _ _ _ _ _ _ _ _ _ _ _ _ _ _ _ _ _ _ _ _ _ _ _ _ _ _ _ _ _ _ _ _ _ _ w1707 _ _ _ _ _ _ _ _ _ _ _ _ _ _ _ _ _ _ _ _ _ _ _ _ _ _ _ _ _ _ _ _ _ w2348 w2371 _ _ _]
      tunnel: [_ _ _ T26[] [{"AlliGator Q Event"=enum."Image:Image Histogram", "Data"=variant}, {"AlliGator Q Event"=enum."Image:Image Contrast", "Data"=variant}] ("AlliGator Actions") w241 w254 _ _ w296 _ _ w315 w322 w332 w344 w355 w367 w374 _ w417 _ w458 _ w491 w501 w512 w527 w544 w551 T26[] [{"AlliGator Q Event"=enum."Image:Image Histogram", "Data"=variant}, {"AlliGator Q Event"=enum."Image:Image Contrast", "Data"=variant}] ("AlliGator Actions") w575 T26[] [{"AlliGator Q Event"=enum."Image:Image Histogram", "Data"=variant}] ("AlliGator Actions") w591 w606 w617 _ w667 w715 w730 w737 _ w779 w809 w819 _ w846 _ w931 w942 w949 _ _ _ w1001 _ w1046 _ w1089 w1100 w1139 w1156 w1174 w1180 w1194 w1203 _ _ w1231 w1239 w1247 w1255 w1277 _ w1306 _ _ w1366 w1404 _ w1436 w1454 w1486 _ _ w1538 w1550 _ _ w1588 _ _ _ _ _ _ _ _ _ _ _ _ _ w1751 _ _ w1797 w1809 _ _ w1847 _ w1876 _ _ _ _ _ _ _ w1993 w2049 _ _ w2112 _ _ _ _ _ _ w2221 w2263 _ w2308 w2325 _ w2370 _ _ w2408] -> w198
      tunnel: [_ _ _ _ _ _ _ _ _ _ _ _ _ _ _ _ _ _ _ w409 _ _ _ w481 _ _ _ _ _ _ _ _ _ _ w616 _ _ _ _ _ _ w771 _ _ _ w844 _ _ _ w951 _ _ _ _ _ w1040 _ _ _ _ _ _ _ _ _ _ _ _ _ _ _ _ _ _ _ _ w1365 _ w1421 _ w1453 _ _ _ _ _ _ _ _ _ _ _ _ _ _ _ _ _ _ _ _ _ _ _ _ _ _ _ _ _ _ _ _ _ _ _ _ _ _ _ _ _ _ _ _ _ _ _ _ _ _ _ _ _ _ _ w2379 _ _ _] -> w193
      tunnel: w188 -> [_ _ _ _ _ _ _ _ _ _ _ _ _ _ _ _ _ _ _ _ _ _ _ _ _ _ _ _ _ _ _ _ _ _ _ _ _ _ _ _ _ _ _ _ _ _ _ _ _ _ _ _ _ _ _ _ _ _ _ _ _ _ _ _ _ _ _ _ _ _ _ _ _ _ _ _ _ _ _ _ _ _ _ _ _ _ _ _ _ _ _ _ _ _ _ _ _ _ _ _ _ _ _ _ _ _ _ _ _ _ _ _ _ _ _ _ _ _ _ _ _ _ _ _ _ _ _ _ _ _ _ _ _ _ _ _ _ w2393 w2398 _]
      tunnel: w187 -> [_ _ _ _ _ _ _ _ _ _ _ _ _ _ _ _ _ _ _ _ _ _ _ _ _ _ _ _ _ _ _ _ _ _ _ _ _ _ _ _ _ _ _ _ _ _ _ _ _ _ _ _ _ _ _ _ _ _ _ _ _ _ _ _ _ _ _ _ _ _ _ _ _ _ _ _ _ _ _ _ _ _ _ _ _ _ _ _ _ _ _ _ _ _ _ _ _ _ _ _ _ _ _ _ _ _ _ _ _ _ _ _ _ _ _ _ _ _ _ _ _ _ _ _ _ _ _ _ _ _ _ _ _ _ _ w2347 _ _ _ _]
      event "Abort Fit": Value Change {
        w219 = TRUE ("Abort?")
        n141 = event-data() -> ()  [unwired: 1 in, 1 out]
        n142 = global write "Abort Fit Global.vi" "Abort Fit"(w219) -> ()
        n143 = global write "Phasor Abort Parallel Computation.vi" "Abort Parallel Computation"(w219) -> ()
      }
      event "Abort ROI Creation": Value Change {
        n144 = event-data() -> ()  [unwired: 1 in, 1 out]
        n145 = global write "Abort ROI Creation Global.vi" "Abort ROI Creation"(TRUE ("Abort?")) -> ()
      }
      event "Abort": Value Change {
        n146 = event-data() -> ()  [unwired: 1 in, 1 out]
        n147 = global write "AlliGator Abort.vi" "Abort?"("Abort") -> ()
      }
      event "Auto-Adjust Contrast": Value Change {
        # "This is not part of the Settings Window and needs to be handled separately"
        n148 = event-data() -> ("NewVal"=w240:bool)  [unwired: 1 in]
        n149 = call "AlliGator Settings Storage.vi"("Get(F)/Set"=TRUE, "AlliGator Settings List"=AlliGator_Settings_List."Source Image:Auto-Adjust Contrast", "Variant Data in"=w240) -> ("Error Out"=w233:errorcluster)  [unwired: 7 in, 1 out]
      }
      event "Calibration Lifetime": Shortcut Menu Selection (User) {
        n150 = event-data() -> ("ItemTag"=w247:string)  [unwired: 1 in]
        n151 = Select(t=w247, s=w249, f=w246) -> (s? t:f=w248:string)
        n152 = case shown="\"Use as Phasor Reference 1 Lifetime\"" w248 {
          tunnel: [_ w250 w252] -> w241
          frame Default {
          }
          frame "Use as Phasor Reference 1 Lifetime" {
            n153 = Build Array(T26 {"AlliGator Q Event"=enum."Phasor Ratio:Use as Phasor Reference 1 Lifetime", "Data"=variant} ("element")) -> (w250:T26[])
          }
          frame "Use as Phasor Reference 2 Lifetime" {
            n154 = Build Array(T26 {"AlliGator Q Event"=enum."Phasor Ratio:Use as Phasor Reference 2 Lifetime", "Data"=variant} ("element")) -> (w252:T26[])
          }
        }
      }
      event Value Change {
        n155 = event-data() -> ("CtlRef"=w263:refnum<vi>, "OldVal"=w262:T9, "NewVal"=w259:T9)  [unwired: 1 in]
        n156 = case shown="True" w260 {
          tunnel: w264 -> [_ w274]
          tunnel: w263 -> [w266 _]
          tunnel: w262 -> [w265 _]
          tunnel: w261 -> [_ _]
          tunnel: w259 -> [_ w271]
          tunnel: [_ w267] -> w254
          frame False {
            n157 = property class="Enum (strict)"(reference=w266, "Value"=w265) -> ()  [unwired: 1 in, 2 out]
          }
          frame True {
            n158 = Bundle By Name(cluster=T26 {"AlliGator Q Event"=enum."Calibration:Set Calibration Type", "Data"=variant} ("element"), "Data"=w271) -> (w272:T26)
            n159 = case shown="\"Phasor Map\"" w271 {
              tunnel: [_ TRUE ("Use Calibration Phasor") FALSE ("Use Calibration Phasor") FALSE ("Use Calibration Phasor")] -> w270
              tunnel: [_ FALSE ("Use Calibration Phasor Curve") TRUE ("Use Calibration Phasor Curve") FALSE ("Use Calibration Phasor Curve")] -> w269
              tunnel: [_ FALSE ("Use Calibration Phasor Map") FALSE ("Use Calibration Phasor Map") TRUE ("Use Calibration Phasor Map")] -> w268
              frame "None", Default {
              }
              frame "Single Phasor" {
              }
              frame "Phasor Series" {
              }
              frame "Phasor Map" {
              }
            }
            n160 = Build Array(w272) -> (w267:T26[])
            n161 = call "AlliGator Check Calibration Menu Items.vi"("Use Calibration Phasor Map"=w268, "Use Calibration Phasor Curve"=w269, "Use Calibration Phasor"=w270, "Menu in"=w274) -> ()  [unwired: 7 in, 1 out]
          }
        }
      }
      event "Clear Image Overlay": Shortcut Menu Activation? {
        n162 = event-data() -> ("MenuRef"=w289:refnum<k9>)  [unwired: 1 in]
        n163 = call "AlliGator Set Check Marks in Source Image Overlay to Erase Button Menu.vi"("Menu in"=w289) -> ("Error Out"=w284:errorcluster)  [unwired: 10 in]
        n164 = event-data() -> ()  [unwired: 2 in, 1 out]
      }
      event "Clear Image Overlay": Shortcut Menu Selection (User) {
        n165 = event-data() -> ("ItemTag"=w295:string)  [unwired: 1 in]
        n166 = call "AlliGator Update Checkmarks in Source Image Overlay to Erase Button Menu.vi"("Source Image Overlay to Erase"=w295) -> ("Error Out"=w290:errorcluster)  [unwired: 10 in]
      }
      event "Clear Image Overlay": Value Change {
        n167 = event-data() -> ()  [unwired: 1 in, 1 out]
        n168 = case shown="True" w301 {
          tunnel: [_ T26[] [{"AlliGator Q Event"=enum."Image:Clear Image Overlay", "Data"=variant}, {"AlliGator Q Event"=enum."Image:Image Contrast", "Data"=variant}] ("element")] -> w296
          frame False {
          }
          frame True {
          }
        }
      }
      event "Clear Phasor Overlay": Shortcut Menu Activation? {
        n169 = event-data() -> ("MenuRef"=w308:refnum<k9>)  [unwired: 1 in]
        n170 = call "AlliGator Set Checkmarks in Phasor Overlay to Erase Button Menu.vi"("Menu in"=w308) -> ("Error Out"=w303:errorcluster)  [unwired: 10 in]
        n171 = event-data() -> ()  [unwired: 2 in, 1 out]
      }
      event "Clear Phasor Overlay": Shortcut Menu Selection (User) {
        n172 = event-data() -> ("ItemTag"=w314:string)  [unwired: 1 in]
        n173 = call "AlliGator Update Checkmarks in Phasor Overlay to Erase Button Menu.vi"("Phasor Plot Overlay to Erase"=w314) -> ("Error Out"=w309:errorcluster)  [unwired: 10 in]
      }
      event "Clear Phasor Overlay": Value Change {
        n174 = event-data() -> ()  [unwired: 1 in, 1 out]
        n175 = case shown="True" w320 {
          tunnel: [_ T26[] [{"AlliGator Q Event"=enum."Phasor Plot:Clear Phasor Overlay", "Data"=variant}] ("element")] -> w315
          frame False {
          }
          frame True {
          }
        }
      }
      event Shortcut Menu Selection (User) {
        n176 = event-data() -> ("ItemTag"=w328:string)  [unwired: 1 in]
        n177 = local read "Current Phasor (g, s)"() -> (w331:T8)
        n178 = Select(t=w328, s=w330, f=w327) -> (s? t:f=w329:string)
        n179 = call "AlliGator Current Phasor (g, s) Custom Menu Actions.vi"("Menu Item Tag"=w329, "Current Phasor"=w331) -> ("AlliGator Actions"=w322:T26[])  [unwired: 9 in]
      }
      event Value Change {
        n180 = event-data() -> ("NewVal"=w338:T8)  [unwired: 1 in]
        n181 = case shown="True" w337 {
          tunnel: w338 -> [_ w341]
          tunnel: [_ w340] -> w332
          frame False {
          }
          frame True {
            n182 = Build Array(w341) -> (w339:T8[])
            n183 = Bundle By Name(cluster=T26 {"AlliGator Q Event"=enum."Phasor Graph:Update Last Phasor Value", "Data"=variant} ("element"), "Data"=w339) -> (w342:T26)
            n184 = Build Array(w342) -> (w340:T26[])
          }
        }
      }
      event Shortcut Menu Selection (User) {
        n185 = event-data() -> ("ItemTag"=w352:string)  [unwired: 1 in]
        n186 = local read "Current Phasor (m, phi)"() -> (w354:T7)
        n187 = Select(t=w352, s=w353, f=w351) -> (s? t:f=w345:string)
        n188 = call "Phasor Convert (m, phi) to (g,s).vi"("Phasor (m, phi)"=w354) -> ("Phasor (g, s)"=w346:T8)  [unwired: 8 in]
        n189 = call "AlliGator Current Phasor (g, s) Custom Menu Actions.vi"("Menu Item Tag"=w345, "Current Phasor"=w346) -> ("AlliGator Actions"=w344:T26[])  [unwired: 9 in]
      }
      event Value Change {
        n190 = event-data() -> ("NewVal"=w361:T7)  [unwired: 1 in]
        n191 = case shown="True" w360 {
          tunnel: w361 -> [_ w363]
          tunnel: [_ w362] -> w355
          frame False {
          }
          frame True {
            n192 = Bundle By Name(cluster=T26 {"AlliGator Q Event"=enum."Phasor Graph:Update Phasor (m, phi)", "Data"=variant} ("element"), "Data"=w363) -> (w364:T26)
            n193 = Build Array(w364) -> (w362:T26[])
          }
        }
      }
      event "Current ROI Analysis": Value Change {
        n194 = event-data() -> ()  [unwired: 1 in, 1 out]
        n195 = case shown="True" w366 {
          tunnel: [_ T26[] [{"AlliGator Q Event"=enum."FLI Dataset:ROI Analysis", "Data"=variant}] ("element")] -> w367
          frame False {
          }
          frame True {
          }
        }
      }
      event "Dataset File/Folder Path", "Dataset File/Folder Path 2", "Dataset File/Folder Path 3", "Dataset File/Folder Path 4", "Dataset File/Folder Path 5", "Dataset File/Folder Path 6", "Dataset File/Folder Path 7", "Dataset File/Folder Path 8", "Dataset File/Folder Path 9", "Dataset File/Folder Path 10", "Dataset File/Folder Path 11": Value Change {
        n196 = event-data() -> ("NewVal"=w375:path)  [unwired: 1 in]
        n197 = Bundle By Name(cluster=T26 {"AlliGator Q Event"=enum."Files:Load File (all Types)_Scriptable", "Data"=variant} ("element"), "Data"=w375) -> (w373:T26)
        n198 = Build Array(w373) -> (w374:T26[])
        n199 = flat-sequence {
          tunnel: w373 -> [_]
          frame #0 {
            w381 = path "" ("File/Folder Path")
            n200 = local write "Dataset File/Folder Path 2"(w381) -> ()
            n201 = local write "Dataset File/Folder Path 3"(w381) -> ()
            n202 = local write "Dataset File/Folder Path 4"(w381) -> ()
            n203 = local write "Dataset File/Folder Path 5"(w381) -> ()
            n204 = local write "Dataset File/Folder Path 6"(w381) -> ()
            n205 = local write "Dataset File/Folder Path 7"(w381) -> ()
            n206 = local write "Dataset File/Folder Path 8"(w381) -> ()
            n207 = local write "Dataset File/Folder Path 9"(w381) -> ()
            n208 = local write "Dataset File/Folder Path 10"(w381) -> ()
            n209 = local write "Dataset File/Folder Path 11"(w381) -> ()
            n210 = local write "Dataset File/Folder Path"(w381) -> ()
          }
        }
      }
      event "Decay Fit Parameter Map Image": Shortcut Menu Activation? {
        w394 = AlliGator_Variables_List."Decay Fit Parameter Map:Palette List" ("Alligator Variable")
        n211 = event-data() -> ("CtlRef"=w385:refnum<vi>, "MenuRef"=w407:refnum<k9>)  [unwired: 1 in]
        n212 = call "Alligator Variables Storage.vi"("Get(F)/Set"=FALSE, "AlliGator Variable"=AlliGator_Variables_List."Decay Fit Parameter Map:Palette Information" ("Alligator Variable")) -> ("Error Out"=w403:errorcluster, "Data out"=w404:variant)  [unwired: 7 in, 1 out]
        n213 = call "Alligator Variables Storage.vi"("Get(F)/Set"=FALSE, "AlliGator Variable"=w394) -> ("Error Out"=w387:errorcluster, "Data out"=w398:variant)  [unwired: 7 in, 1 out]
        n214 = Variant To Data(error in=w403, type=T31 {"Palette Name [# Colors,int?,inv?]"="", "Palette Type"=0, "Palette Colors"=[], "Interpolate?"=FALSE} ("Image Display Palette Information"), Variant=w404) -> (data=w402:T31, error out=w389:errorcluster)
        n215 = call-poly "Variant to Data.vi"("Variant"=w398) -> ("String Array"=w397:string[])  [unwired: 8 in]
        n216 = Unbundle By Name(w402) -> ("Palette Name [# Colors,int?,inv?]"=w400:string)
        n217 = Merge Errors(w389, w387) -> (w388:errorcluster)
        n218 = call "Check Selected Palette in Menu.vi"("Error In"=w388, "Palette List"=w397, "Checked Palette"=w400, "Menu in"=w407) -> ("Error Out"=w386:errorcluster, "Stored Palette List"=w395:string[], "menu reference out"=w384:refnum<k9>)  [unwired: 5 in]
        n219 = call "Alligator Variables Storage.vi"("Get(F)/Set"=TRUE, "AlliGator Variable"=w394, "Error In"=w386, "Data in"=w395) -> ("Error Out"=w383:errorcluster)  [unwired: 5 in, 2 out]
        n220 = call "AlliGator Add Python Functions to Object Menu.vi"("error in (no error)"=w383, "Menu in"=w384, "Object Refnum"=w385) -> ("error out"=w382:errorcluster)  [unwired: 6 in, 2 out]
        n221 = event-data() -> ()  [unwired: 2 in, 1 out]
      }
      event "Decay Fit Parameter Map Image": Shortcut Menu Selection (User) {
        n222 = event-data() -> ("CtlRef"=w422:refnum<vi>, "ItemTag"=w418:string, "ItemPath"=w421:string, "Coords"=w416:T37)  [unwired: 1 in]
        n223 = call-poly <vilib>:"Acquire Input Data.vi"("device ID"=w414, "error in (no error)"=w415) -> ("device ID"=w412:refnum<k1>, "keys pressed"=w411:T52, "error out"=w413:errorcluster)  [unwired: 15 in]
        n224 = case shown="True" w410 {
          tunnel: w422 -> [_ w433]
          tunnel: w421 -> [_ w432]
          tunnel: w418 -> [_ w431]
          tunnel: [_ w430] -> w417
          tunnel: w416 -> [_ w429]
          tunnel: w411 -> [_ w425]
          tunnel: [_ w424] -> w409
          tunnel: [_ w423] -> w408
          frame False {
          }
          frame True {
            n225 = Index Array(array=w425) -> (element=w428:T34)  [unwired: 1 in]
            n226 = Equal?(x=w428, y=T34."H" ("element")) -> (x = y?=w426:bool)
            n227 = case shown="False" w426 {
              tunnel: w433 -> [w440 w446]
              tunnel: w432 -> [w438 _]
              tunnel: w431 -> [w439 w445]
              tunnel: [w442 _] -> w430
              tunnel: w429 -> [w437 _]
              tunnel: [_ w444] -> w424
              tunnel: [w435 w443] -> w423
              frame False {
                n228 = local read "Decay Fit Parameter"() -> (w434:T11)
                n229 = Bundle By Name(cluster=T35 {"Item Tag"="", "Image Control Refnum"=refnum, "Coords"={"Horizontal"=0, "Vertical"=0}, "Item Path"=""} ("Image Event Data"), "Image Control Refnum"=w440, "Item Tag"=w439, "Item Path"=w438, "Coords"=w437) -> (w436:T35)
                n230 = call "AlliGator Decay Fit Parameter Map Context Menu Handler.vi"("Decay Fit Parameter"=w434, "Image Event Data"=w436) -> ("Error Out"=w435:errorcluster, "AlliGator Actions"=w442:T26[])  [unwired: 8 in]
              }
              frame True {
                n231 = property class="ImageControl"(reference=w446) -> ("Label.Text"=w447:string)  [unwired: 1 in, 2 out]
                n232 = call "AlliGator Send Python Function Doc String to Notebook.vi"("Item Tag"=w445, "Target"=w447) -> ("Error Out"=w443:errorcluster, "Message"=w444:string)  [unwired: 8 in]
              }
            }
          }
        }
      }
      event "Decay Fit Parameter Map ROI Color": Value Change {
        n233 = event-data() -> ("NewVal"=w448:u32)  [unwired: 1 in]
        n234 = call <vilib>:"Color to RGB.vi"("Color"=w448) -> ("R"=w451:u8, "G"=w452:u8, "B"=w453:u8)  [unwired: 1 out]
        n235 = Bundle By Name(cluster=cluster{"Red":u8, "Green":u8, "Blue":u8} {"Red"=0, "Green"=0, "Blue"=0} ("ROI Color"), "Red"=w451, "Green"=w452, "Blue"=w453) -> (w450:cluster{"Red":u8, "Green":u8, "Blue":u8})
        n236 = property on="Decay Fit Parameter Map Image" class="ImageControl"("ROI Color"=w450) -> ()  [unwired: 2 in, 2 out]
      }
      event Value Change {
        n237 = event-data() -> ("NewVal"=w461:T11)  [unwired: 1 in]
        n238 = case shown="True" w464 {
          tunnel: w461 -> [_ w470]
          tunnel: [_ w465] -> w458
          frame False {
          }
          frame True {
            w467 = TRUE  # Parameter changed
            n239 = Bundle(cluster=T38 {"Parameter"=enum."Offset", "Parameter changed"=FALSE} ("output cluster"), "Parameter"=w470, "Parameter changed"=w467) -> (w468:T38)
            n240 = Bundle By Name(cluster=T26 {"AlliGator Q Event"=enum."Decay Fit Parameter Map:Build Decay Fit Parameter Map", "Data"=variant} ("Time-Gated Phasor Q Element"), "Data"=w468) -> (w471:T26)
            n241 = Build Array(w471, T26 {"AlliGator Q Event"=enum."Image:Update Image Profile Plots", "Data"=variant} ("Time-Gated Phasor Q Element")) -> (w465:T26[])
          }
        }
      }
      event "Decay Graph Active": Value Change {
        n242 = event-data() -> ("NewVal"=w480:bool)  [unwired: 1 in]
        n243 = call "AlliGator Settings Storage.vi"("Get(F)/Set"=TRUE, "AlliGator Settings List"=AlliGator_Settings_List."Fluorescence Decay:Decay Graph Active", "Variant Data in"=w480) -> ("Error Out"=w473:errorcluster)  [unwired: 7 in, 1 out]
      }
      event "Decay Graph", "Decay Statistics Graph", "Intensity Time Trace", "Image Histogram": Shortcut Menu Selection (User) {
        # "Shortcut Menu (User)"
        n244 = event-data() -> ("CtlRef"=w486:refnum<vi>, "Coords"=w489:T37, "ItemTag"=w488:string, "ItemPath"=w487:string)  [unwired: 1 in]
        n245 = call-poly <vilib>:"Acquire Input Data.vi"("device ID"=w494, "error in (no error)"=w492) -> ("device ID"=w495:refnum<k1>, "keys pressed"=w496:T52, "error out"=w493:errorcluster)  [unwired: 15 in]
        n246 = Index Array(array=w496) -> (element=w498:T34)  [unwired: 1 in]
        n247 = Equal?(x=w498, y=T34."H" ("element")) -> (x = y?=w483:bool)
        n248 = Bundle By Name(cluster=T39 {"Item Tag"="", "XY Graph Refnum"=refnum, "Coords"={"Horizontal"=0, "Vertical"=0}, "Item Path"=""} ("XY Graph Event"), "XY Graph Refnum"=w486, "Coords"=w489, "Item Tag"=w488, "Item Path"=w487) -> (w485:T39)
        n249 = call "AlliGator Special Graph Menu Actions.vi"("Help?"=w483, "Animated Busy Icon"=w484, "XY Graph Event"=w485) -> ("Error Out"=w482:errorcluster, "Message"=w481:string, "AlliGator Actions"=w491:T26[])  [unwired: 6 in]
      }
      event "Decay Statistics Bin": Value Change {
        n250 = event-data() -> ("CtlRef"=w507:refnum<vi>, "OldVal"=w506:i32)  [unwired: 1 in]
        n251 = case shown="True" w508 {
          tunnel: w507 -> [w510 _]
          tunnel: w506 -> [w509 _]
          tunnel: [_ T26[] [{"AlliGator Q Event"=enum."FLI Dataset:Update Decay Statistics Graph", "Data"=variant}] ("element")] -> w501
          frame False {
            n252 = property class="DigNum (strict)"(reference=w510, "Value"=w509) -> ()  [unwired: 1 in, 2 out]
          }
          frame True {
          }
        }
      }
      event Value Change {
        n253 = event-data() -> ("CtlRef"=w517:refnum<vi>, "NewVal"=w518:T2)  [unwired: 1 in]
        n254 = case shown="True" w519 {
          tunnel: w518 -> [w521 w523]
          tunnel: w517 -> [w520 _]
          tunnel: [_ w522] -> w512
          frame False {
            n255 = property class="Enum (strict)"(reference=w520, "Value"=w521) -> ()  [unwired: 1 in, 2 out]
          }
          frame True {
            n256 = Bundle By Name(cluster=T26 {"AlliGator Q Event"=enum."GUI:Type of Displayed Image Changed", "Data"=variant} ("array"), "Data"=w523) -> (w524:T26)
            n257 = Build Array (concatenate)(w524, T26[] [{"AlliGator Q Event"=enum."Image:Image Histogram", "Data"=variant}, {"AlliGator Q Event"=enum."Image:Image Contrast", "Data"=variant}] ("element")) -> (w522:T26[])
          }
        }
      }
      event "Gate Image Slide": Value Change {
        n258 = event-data() -> ("CtlRef"=w533:refnum<vi>, "OldVal"=w532:u16, "NewVal"=w535:u16)  [unwired: 1 in]
        n259 = case shown="False" w534 {
          tunnel: w535 -> [_ w539]
          tunnel: w533 -> [w537 _]
          tunnel: w532 -> [w536 _]
          tunnel: [_ w538] -> w527
          frame False {
            n260 = property class="Slide (strict)"(reference=w537, "Value"=w536) -> ()  [unwired: 1 in, 2 out]
          }
          frame True {
            n261 = Bundle By Name(cluster=T26 {"AlliGator Q Event"=enum."GUI:Gate Image Slide Changed", "Data"=variant} ("element"), "Data"=w539) -> (w540:T26)
            n262 = Build Array(w540, T26 {"AlliGator Q Event"=enum."Image:Image Histogram", "Data"=variant} ("element"), T26 {"AlliGator Q Event"=enum."Image:Image Contrast", "Data"=variant} ("element")) -> (w538:T26[])
          }
        }
      }
      event "Highlight Image ROI": Value Change {
        n263 = event-data() -> ()  [unwired: 1 in, 1 out]
        n264 = case shown="True" w549 {
          tunnel: [_ T26[] [{"AlliGator Q Event"=enum."Phasor Plot:Highlight Image ROI in Phasor Plot", "Data"=variant}] ("element")] -> w544
          frame False {
          }
          frame True {
          }
        }
      }
      event "Highlight Phasor in Source Image": Value Change {
        n265 = event-data() -> ()  [unwired: 1 in, 1 out]
        n266 = case shown="True" w556 {
          tunnel: [_ T26[] [{"AlliGator Q Event"=enum."Phasor Plot:Overlay Phasor ROI, Ratio or Map in Source Image", "Data"=variant}] ("element")] -> w551
          frame False {
          }
          frame True {
          }
        }
      }
      event "Histogram Upper Percentile", "Histogram Lower Percentile": Value Change {
        # "This is not part of the Settings Window and needs to be handled separately"
        n267 = event-data() -> ("CtlRef"=w561:refnum<vi>, "NewVal"=w559:dbl)  [unwired: 1 in]
        n268 = property class="DigNum (strict)"(reference=w561) -> ("Label.Text"=w560:string)  [unwired: 1 in, 2 out]
        n269 = case shown="\"Histogram Upper Percentile\"" w560 {
          tunnel: [_ w568 w572] -> w562
          tunnel: w559 -> [_ w567 w571]
          frame "", Default {
          }
          frame "Histogram Lower Percentile" {
            n270 = local write "Lower Percentile"(w567) -> ()
            n271 = call "AlliGator Settings Storage.vi"("Get(F)/Set"=TRUE, "AlliGator Settings List"=AlliGator_Settings_List."Source Image:Histogram Lower Percentile", "Variant Data in"=w567) -> ("Error Out"=w568:errorcluster)  [unwired: 7 in, 1 out]
          }
          frame "Histogram Upper Percentile" {
            n272 = local write "Upper Percentile"(w571) -> ()
            n273 = call "AlliGator Settings Storage.vi"("Get(F)/Set"=TRUE, "AlliGator Settings List"=AlliGator_Settings_List."Source Image:Histogram Upper Percentile", "Variant Data in"=w571) -> ("Error Out"=w572:errorcluster)  [unwired: 7 in, 1 out]
          }
        }
      }
      event "Image Color Scale": Mouse Up {
        n274 = event-data() -> ()  [unwired: 1 in, 1 out]
        n275 = case shown="True" w580 {
          tunnel: [_ T26[] [{"AlliGator Q Event"=enum."Image:Image Contrast", "Data"=variant}] ("element")] -> w575
          frame False {
          }
          frame True {
          }
        }
      }
      event "Image Histogram Active": Value Change {
        n276 = event-data() -> ("NewVal"=w590:bool)  [unwired: 1 in]
        n277 = call "AlliGator Settings Storage.vi"("Get(F)/Set"=TRUE, "AlliGator Settings List"=AlliGator_Settings_List."Source Image:Image Histogram Active", "Variant Data in"=w590) -> ("Error Out"=w583:errorcluster)  [unwired: 7 in, 1 out]
      }
      event Value Change {
        n278 = event-data() -> ()  [unwired: 1 in, 1 out]
        n279 = case shown="True" w596 {
          tunnel: [_ w597] -> w591
          frame False {
          }
          frame True {
            n280 = Build Array(T26 {"AlliGator Q Event"=enum."Image:Image Histogram", "Data"=variant} ("element")) -> (w597:T26[])
          }
        }
      }
      event "Image Histogram": Cursor Move {
        w600 = T26 {"AlliGator Q Event"=enum."Image:Image Histogram Cursor Move", "Data"=variant} ("Time-Gated Phasor Q Element")
        n281 = event-data() -> ("Time"=w599:u32)  [unwired: 1 in]
        n282 = property on="Auto-Adjust Contrast" class="Bool (strict)"() -> ("Value"=w602:bool)  [unwired: 2 in, 2 out]
        n283 = case shown="True" w602 {
          frame False {
          }
          frame True {
            n284 = property on="Auto-Adjust Contrast" class="Bool (strict)"("Val(Sgnl)"=FALSE ("Auto-Adjust Contrast")) -> ()  [unwired: 2 in, 2 out]
          }
        }
        n285 = call "AlliGator Filter Event.vi"("Time"=w599, "Time-Gated Phasor Q Element"=w600) -> ("Filter Event?"=w601:bool)  [unwired: 8 in, 1 out]
        n286 = call "AlliGator Image Contrast Status.vi"("Read/Write"=Read-Write."Read") -> ("Flag (out)"=w603:bool)  [unwired: 8 in]
        n287 = Or(x=w601, y=w603) -> (x .or. y?=w604:bool)
        n288 = case shown="False" w604 {
          tunnel: w600 -> [w615 _]
          tunnel: [w614 _] -> w606
          frame False {
            # "event not filtered out"
            n289 = call "AlliGator Image Contrast Status.vi"("Flag (in)"=TRUE, "Read/Write"=Read-Write."Write") -> ()  [unwired: 7 in, 1 out]
            n290 = Build Array(w615) -> (w614:T26[])
          }
          frame True {
          }
        }
      }
      event "Intensity Correction File": Value Change {
        n291 = event-data() -> ("NewVal"=w626:path, "CtlRef"=w624:refnum<vi>)  [unwired: 1 in]
        n292 = case shown="True" w623 {
          tunnel: w626 -> [_ w629]
          tunnel: w625 -> [_ w634]
          tunnel: w624 -> [_ w632]
          tunnel: [_ w630] -> w618
          tunnel: [_ w628] -> w617
          tunnel: [_ w627] -> w616
          frame False {
          }
          frame True {
            n293 = property class="Path"(reference=w632) -> (reference out=w635:refnum<vi>, error out=w633:errorcluster, "Label.Text"=w636:string)  [unwired: 1 in]
            n294 = Empty String/Path?(string/path=w629) -> (empty?=w637:bool)
            n295 = case shown="False" w637 {
              selector: w637 -> [_ w643]
              tunnel: w629 -> [w639 _]
              tunnel: [w638 _] -> w628
              frame False {
                n296 = Bundle By Name(cluster=T26 {"AlliGator Q Event"=enum."Intensity Time Trace:Load Intensity Corrections File", "Data"=variant} ("Time-Gated Phasor Q Element"), "Data"=w639) -> (w640:T26)
                n297 = Build Array(w640) -> (w638:T26[])
              }
              frame True {
                n298 = Not(x=w643) -> (.not. x?=w642:bool)
                n299 = property on="Use Intensity Correction File" class="Bool (strict)"("Val(Sgnl)"=w642) -> ()  [unwired: 2 in, 2 out]
              }
            }
            n300 = call "AlliGator Get Control Notebook String.vi"("error in (no error)"=w633, "Value"=w629, "Control Label"=w636) -> ("error out"=w631:errorcluster, "Notebook String"=w627:string)  [unwired: 7 in]
            n301 = call "AlliGator Update Settings & Control.vi"("Error In"=w631, "Value"=w629, "Sender"=w634, "CtlRef"=w635) -> ("Error Out"=w630:errorcluster)  [unwired: 7 in]
          }
        }
      }
      event "Lifetime & Other Parameters Graph", "Phasor Ratio Graph", "Decay Graph", "Phasor Graph", "Decay Statistics Graph", "Intensity Time Trace", "Image Histogram": Shortcut Menu Activation? {
        # "Shortcut Menu Activation"
        n302 = event-data() -> ("CtlRef"=w659:refnum<vi>, "MenuRef"=w658:refnum<k9>)  [unwired: 1 in]
        n303 = call "XY Graph Check-Uncheck Menu Items.vi"("Menu in"=w658, "XY Graph Refnum"=w659) -> ("Error Out (dup)"=w653:errorcluster, "Menu out"=w647:refnum<k9>, "XY Graph Refnum dup"=w645:T42)  [unwired: 6 in, 1 out]
        n304 = call "XY Graph Get Label.vi"("XYGraph"=w645) -> ("Graph Label"=w644:string)  [unwired: 8 in]
        n305 = case shown="\"Decay Graph\"" w644 {
          tunnel: w653 -> [w660 w666]
          tunnel: [w660 w665] -> w648
          tunnel: w647 -> [w661 w664]
          tunnel: [w661 w663] -> w646
          frame "", Default {
          }
          frame "Decay Graph" {
            n306 = call "AlliGator Decay Graph Get-Set Process Plot Target.vi"("Get (F)/Set"=FALSE, "Error In"=w666, "Menu"=w664) -> ("Error Out (dup)"=w665:errorcluster, "Menu"=w663:refnum<k9>)  [unwired: 6 in, 1 out]
          }
        }
        n307 = call "AlliGator Add Python Functions to Object Menu.vi"("error in (no error)"=w648, "Menu in"=w646, "Object Refnum"=w645) -> ("error out"=w652:errorcluster, "Menu out"=w650:refnum<k9>, "Object Refnum dup"=w649:refnum<vi>)  [unwired: 6 in]
        n308 = call "AlliGator Grayed out Menu Items.vi"("error in (no error)"=w652, "Menu in"=w650, "Object Refnum"=w649) -> ("error out"=w651:errorcluster)  [unwired: 7 in, 1 out]
        n309 = event-data() -> ()  [unwired: 2 in, 1 out]
      }
      event "Lifetime & Other Parameters Graph": Shortcut Menu Selection (User) {
        n310 = event-data() -> ("ItemPath"=w668:string, "CtlRef"=w678:refnum<vi>, "Coords"=w677:T37, "ItemTag"=w669:string)  [unwired: 1 in]
        n311 = Select(t=w669, s=w676, f=w674) -> (s? t:f=w675:string)
        n312 = case shown="\"Plot Histogram\"" w675 {
          selector: w675 -> [_ w681 _ _ _ _ _]
          tunnel: w678 -> [_ w683 _ _ _ w704 w711]
          tunnel: w677 -> [_ w682 _ _ _ w703 w710]
          tunnel: w668 -> [_ w680 _ _ _ _ _]
          tunnel: [_ w679 _ w689 w699 w706 w713] -> w667
          frame "", "Busy" {
          }
          frame Default {
            n313 = Bundle By Name(cluster=T39 {"Item Tag"="", "XY Graph Refnum"=refnum, "Coords"={"Horizontal"=0, "Vertical"=0}, "Item Path"=""} ("XY Graph Event"), "Item Path"=w680, "XY Graph Refnum"=w683, "Coords"=w682, "Item Tag"=w681) -> (w686:T39)
            n314 = Bundle By Name(cluster=T26 {"AlliGator Q Event"=enum."Generic Graph:Generic XY Graph Event", "Data"=variant} ("element"), "Data"=w686) -> (w684:T26)
            n315 = Build Array(w684) -> (w679:T26[])
          }
          frame "-----------------" {
          }
          frame "New Plot" {
            w688 = T53 {"Multiplot XY Graph"=refnum, "Plot Name"="", "Plot Scales"={"X Scale"=0, "Y Scale"=0}, "Plot Interpolation"=enum."Use Previous Plot's Style", "Point Style"=enum."not defined", "Plot Color"=15781887, "Plot Metadata"=variant} ("New Plot Information")
            w693 = T26 {"AlliGator Q Event"=enum."Generic Graph:New Plot", "Data"=variant} ("Time-Gated Phasor Q Element")
            n316 = control-ref of="Lifetime & Other Parameters Graph"() -> (w690:refnum<vi>)
            n317 = control-ref of="Phasor Ratio Graph"() -> (w691:refnum<vi>)
            n318 = Bundle By Name(cluster=w688, "Multiplot XY Graph"=w691, "Plot Name"="Phasor Ratio") -> (w697:T53)
            n319 = Bundle By Name(cluster=w688, "Multiplot XY Graph"=w690, "Plot Name"="Lifetime") -> (w694:T53)
            n320 = Bundle By Name(cluster=w693, "Data"=w697) -> (w698:T26)
            n321 = Bundle By Name(cluster=w693, "Data"=w694) -> (w692:T26)
            n322 = Build Array(w698, w692) -> (w689:T26[])
          }
          frame "Plot Decay Shifts" {
            n323 = Build Array(T26 {"AlliGator Q Event"=enum."Lifetime:Plot Decay Shifts", "Data"=variant} ("element")) -> (w699:T26[])
          }
          frame "Compute Sliced Mean, SDV and CV Plots" {
            n324 = Bundle By Name(cluster=T41 {"Multiplot XY Graph"=refnum, "Mouse Coordinates"={"Horizontal"=0, "Vertical"=0}} ("Mouse Click Event Data"), "Multiplot XY Graph"=w704, "Mouse Coordinates"=w703) -> (w701:T41)
            n325 = Bundle By Name(cluster=T26 {"AlliGator Q Event"=enum."Lifetime:Compute Sliced Mean, SDV and CV Plots", "Data"=variant} ("element"), "Data"=w701) -> (w705:T26)
            n326 = Build Array(w705) -> (w706:T26[])
          }
          frame "Plot Histogram" {
            n327 = Bundle By Name(cluster=T41 {"Multiplot XY Graph"=refnum, "Mouse Coordinates"={"Horizontal"=0, "Vertical"=0}} ("Mouse Click Event Data"), "Multiplot XY Graph"=w711, "Mouse Coordinates"=w710) -> (w708:T41)
            n328 = Bundle By Name(cluster=T26 {"AlliGator Q Event"=enum."Lifetime:Plot Histogram", "Data"=variant} ("element"), "Data"=w708) -> (w712:T26)
            n329 = Build Array(w712) -> (w713:T26[])
          }
        }
      }
      event "Map Parameter", "Parameter Map Set": Value Change {
        n330 = event-data() -> ()  [unwired: 1 in, 1 out]
        n331 = case shown="True" w720 {
          tunnel: [_ w723] -> w715
          frame False {
          }
          frame True {
            w725 = TRUE  # Parameter changed
            n332 = local read "Parameter Map Set"() -> (w722:u16)
            n333 = local read "Map Parameter"() -> (w721:u16)
            n334 = Bundle By Name(cluster=T43 {"Parameter"=0, "Parameter changed"=FALSE, "Map Set"=0} ("output cluster"), "Parameter"=w721, "Parameter changed"=w725, "Map Set"=w722) -> (w726:T43)
            n335 = Bundle By Name(cluster=T26 {"AlliGator Q Event"=enum."Parameter Map:Build Parameter Map", "Data"=variant} ("Time-Gated Phasor Q Element"), "Data"=w726) -> (w728:T26)
            n336 = Build Array(w728, T26 {"AlliGator Q Event"=enum."Image:Update Image Profile Plots", "Data"=variant} ("Time-Gated Phasor Q Element")) -> (w723:T26[])
          }
        }
      }
      event "Overlay Decay Fit Parameter Map": Value Change {
        n337 = event-data() -> ()  [unwired: 1 in, 1 out]
        n338 = case shown="True" w735 {
          tunnel: [_ T26[] [{"AlliGator Q Event"=enum."Decay Fit Parameter Map:Overlay Decay Fit Parameter Map in Source Image", "Data"=variant}] ("element")] -> w730
          frame False {
          }
          frame True {
          }
        }
      }
      event "Overlay Parameter Map": Value Change {
        n339 = event-data() -> ()  [unwired: 1 in, 1 out]
        n340 = case shown="True" w742 {
          tunnel: [_ T26[] [{"AlliGator Q Event"=enum."Parameter Map:Overlay Parameter Map in Source Image", "Data"=variant}] ("element")] -> w737
          frame False {
          }
          frame True {
          }
        }
      }
      event "Parameter Map Image": Shortcut Menu Activation? {
        w756 = AlliGator_Variables_List."Parameter Map:Palette List" ("Alligator Variable")
        n341 = event-data() -> ("CtlRef"=w747:refnum<vi>, "MenuRef"=w769:refnum<k9>)  [unwired: 1 in]
        n342 = call "Alligator Variables Storage.vi"("Get(F)/Set"=FALSE, "AlliGator Variable"=AlliGator_Variables_List."Parameter Map:Palette Information" ("Alligator Variable")) -> ("Error Out"=w765:errorcluster, "Data out"=w766:variant)  [unwired: 7 in, 1 out]
        n343 = call "Alligator Variables Storage.vi"("Get(F)/Set"=FALSE, "AlliGator Variable"=w756) -> ("Error Out"=w749:errorcluster, "Data out"=w760:variant)  [unwired: 7 in, 1 out]
        n344 = Variant To Data(error in=w765, type=T31 {"Palette Name [# Colors,int?,inv?]"="", "Palette Type"=0, "Palette Colors"=[], "Interpolate?"=FALSE} ("Image Display Palette Information"), Variant=w766) -> (data=w764:T31, error out=w751:errorcluster)
        n345 = call-poly "Variant to Data.vi"("Variant"=w760) -> ("String Array"=w759:string[])  [unwired: 8 in]
        n346 = Unbundle By Name(w764) -> ("Palette Name [# Colors,int?,inv?]"=w762:string)
        n347 = Merge Errors(w751, w749) -> (w750:errorcluster)
        n348 = call "Check Selected Palette in Menu.vi"("Error In"=w750, "Palette List"=w759, "Checked Palette"=w762, "Menu in"=w769) -> ("Error Out"=w748:errorcluster, "Stored Palette List"=w757:string[], "menu reference out"=w746:refnum<k9>)  [unwired: 5 in]
        n349 = call "Alligator Variables Storage.vi"("Get(F)/Set"=TRUE, "AlliGator Variable"=w756, "Error In"=w748, "Data in"=w757) -> ("Error Out"=w745:errorcluster)  [unwired: 5 in, 2 out]
        n350 = call "AlliGator Add Python Functions to Object Menu.vi"("error in (no error)"=w745, "Menu in"=w746, "Object Refnum"=w747) -> ("error out"=w744:errorcluster)  [unwired: 6 in, 2 out]
        n351 = event-data() -> ()  [unwired: 2 in, 1 out]
      }
      event "Parameter Map Image": Shortcut Menu Selection (User) {
        n352 = event-data() -> ("CtlRef"=w784:refnum<vi>, "ItemTag"=w780:string, "ItemPath"=w783:string, "Coords"=w778:T37)  [unwired: 1 in]
        n353 = call-poly <vilib>:"Acquire Input Data.vi"("device ID"=w776, "error in (no error)"=w777) -> ("device ID"=w774:refnum<k1>, "keys pressed"=w773:T52, "error out"=w775:errorcluster)  [unwired: 15 in]
        n354 = case shown="True" w772 {
          tunnel: w784 -> [_ w795]
          tunnel: w783 -> [_ w794]
          tunnel: w780 -> [_ w793]
          tunnel: [_ w792] -> w779
          tunnel: w778 -> [_ w791]
          tunnel: w773 -> [_ w787]
          tunnel: [_ w786] -> w771
          tunnel: [_ w785] -> w770
          frame False {
          }
          frame True {
            n355 = Index Array(array=w787) -> (element=w790:T34)  [unwired: 1 in]
            n356 = Equal?(x=w790, y=T34."H" ("element")) -> (x = y?=w788:bool)
            n357 = case shown="False" w788 {
              tunnel: w795 -> [w801 w807]
              tunnel: w794 -> [w799 _]
              tunnel: w793 -> [w800 w806]
              tunnel: [w803 _] -> w792
              tunnel: w791 -> [w798 _]
              tunnel: [_ w805] -> w786
              tunnel: [w796 w804] -> w785
              frame False {
                n358 = Bundle By Name(cluster=T35 {"Item Tag"="", "Image Control Refnum"=refnum, "Coords"={"Horizontal"=0, "Vertical"=0}, "Item Path"=""} ("Image Event Data"), "Image Control Refnum"=w801, "Item Tag"=w800, "Item Path"=w799, "Coords"=w798) -> (w797:T35)
                n359 = call "AlliGator Parameter Map Context Menu Handler.vi"("Image Event Data"=w797) -> ("Error Out"=w796:errorcluster, "AlliGator Actions"=w803:T26[])  [unwired: 9 in]
              }
              frame True {
                n360 = property class="ImageControl"(reference=w807) -> ("Label.Text"=w808:string)  [unwired: 1 in, 2 out]
                n361 = call "AlliGator Send Python Function Doc String to Notebook.vi"("Item Tag"=w806, "Target"=w808) -> ("Error Out"=w804:errorcluster, "Message"=w805:string)  [unwired: 8 in]
              }
            }
          }
        }
      }
      event "Parameter Map Set": Shortcut Menu Selection (User) {
        n362 = event-data() -> ("ItemTag"=w811:string)  [unwired: 1 in]
        n363 = case shown="True" w810 {
          tunnel: w811 -> [_ w817]
          tunnel: [_ w816] -> w809
          frame False {
          }
          frame True {
            n364 = case shown="\"Delete Parameter Map Set\"" w817 {
              tunnel: [_ T26[] [{"AlliGator Q Event"=enum."Parameter Map:Delete Parameter Map Set", "Data"=variant}] ("AlliGator Actions")] -> w816
              frame "", Default {
              }
              frame "Delete Parameter Map Set" {
              }
            }
          }
        }
      }
      event "Phasor Frame Slide": Value Change {
        n365 = event-data() -> ("CtlRef"=w825:refnum<vi>, "OldVal"=w824:i32, "NewVal"=w827:i32)  [unwired: 1 in]
        n366 = case shown="True" w826 {
          tunnel: w827 -> [_ w831]
          tunnel: w825 -> [w829 _]
          tunnel: w824 -> [w828 _]
          tunnel: [_ w830] -> w819
          frame False {
            n367 = property class="Slide (strict)"(reference=w829, "Value"=w828) -> ()  [unwired: 1 in, 2 out]
          }
          frame True {
            n368 = Bundle By Name(cluster=T26 {"AlliGator Q Event"=enum."Phasor Graph:Show Single Phasor", "Data"=variant} ("element"), "Data"=w831) -> (w832:T26)
            n369 = Build Array(w832) -> (w830:T26[])
          }
        }
      }
      event "Phasor Graph Active": Value Change {
        n370 = event-data() -> ("NewVal"=w841:bool)  [unwired: 1 in]
        n371 = call "AlliGator Settings Storage.vi"("Get(F)/Set"=TRUE, "AlliGator Settings List"=AlliGator_Settings_List."Phasor Graph:Phasor Graph Active", "Variant Data in"=w841) -> ("Error Out"=w834:errorcluster)  [unwired: 7 in, 1 out]
      }
      event "Phasor Graph Frequency", "Calibration Lifetime", "Save Phasor Plot", "Save Phasor Graph Image", "Phasor Plot Frequency", "Save Source Image", "Use Image Histogram for Contrast": Value Change {
        # "Each new control duplicated in the Settings Window needs to be added to this case\nunless it has its own event case\nThe labels of the controls need to be identical (in the Main AlliGator window and in the Settings window)"
        n372 = event-data() -> ("CtlRef"=w856:refnum<vi>)  [unwired: 1 in]
        n373 = property class="Ctl"(reference=w856) -> (reference out=w843:refnum<vi>, error out=w855:errorcluster, "Label.Text"=w842:string, "Value"=w850:variant)  [unwired: 1 in]
        n374 = case shown="\"Phasor Graph Frequency\"" w842 {
          tunnel: w855 -> [w857 w858 w860 w874 w895]
          tunnel: [w857 w858 w861 w878 w898] -> w854
          tunnel: [_ T26[] [{"AlliGator Q Event"=enum."Image:Image Histogram", "Data"=variant}, {"AlliGator Q Event"=enum."Image:Image Contrast", "Data"=variant}] ("AlliGator Actions") _ T26[] [{"AlliGator Q Event"=enum."Phasor Graph:Update SEPL Plot", "Data"=variant}] ("element") T26[] [{"AlliGator Q Event"=enum."Phasor Graph:Update SEPL Plot", "Data"=variant}] ("element")] -> w846
          tunnel: w851 -> [_ _ _ w881 w900]
          tunnel: w850 -> [_ _ _ w876 w896]
          frame "", Default {
            # "only updates the corresponding Settings window control"
          }
          frame "Use Image Histogram for Contrast" {
          }
          frame "Calibration Lifetime" {
            n375 = disable-structure shown="Disabled" {
              disable-tunnel: [w864 _] -> w861
              disable-tunnel: w860 -> [w863 _]
              frame Disabled {
                n376 = call "Alligator Variables Storage.vi"("AlliGator Variable"=AlliGator_Variables_List."Phasor Plot:Computed" ("Alligator Variable"), "Error In"=w863) -> ("Error Out"=w862:errorcluster, "Data out"=w866:variant)  [unwired: 7 in, 1 out]
                n377 = call-poly "Variant to Data.vi"("Variant"=w866) -> ("Value"=w865:bool)  [unwired: 8 in]
                n378 = case shown="True" w865 {
                  tunnel: w862 -> [w868 w871]
                  tunnel: [w868 w869] -> w864
                  frame False {
                  }
                  frame True {
                    n379 = call "AlliGator Set Phasor Plot Update LED.vi"("error in (no error)"=w871, "Off/On"=TRUE) -> ("error out"=w869:errorcluster)  [unwired: 9 in]
                  }
                }
              }
              frame Enabled {
              }
            }
          }
          frame "Phasor Plot Frequency" {
            # "Need to update TWO controls"
            n380 = Variant To Data(error in=w874, type=dbl[unit] 0.0 ("Calibration Phasor Frequency"), Variant=w876) -> (data=w872:dbl[unit], error out=w873:errorcluster)
            n381 = control-ref of="Phasor Graph Frequency"() -> (w880:refnum<vi>)
            n382 = call "Alligator Variables Storage.vi"("AlliGator Variable"=AlliGator_Variables_List."Phasor Plot:Computed" ("Alligator Variable"), "Error In"=w874) -> ("Error Out"=w879:errorcluster, "Data out"=w884:variant)  [unwired: 7 in, 1 out]
            n383 = local write "Phasor Graph Frequency"(w872) -> ()
            n384 = call "AlliGator Update Settings & Control.vi"("Error In"=w873, "Value"=w872, "Sender"=w881, "CtlRef"=w880) -> ("Error Out"=w877:errorcluster)  [unwired: 7 in]
            n385 = call-poly "Variant to Data.vi"("Variant"=w884) -> ("Value"=w883:bool)  [unwired: 8 in]
            n386 = case shown="True" w883 {
              tunnel: w879 -> [w887 w890]
              tunnel: [w887 w888] -> w886
              frame False {
              }
              frame True {
                n387 = call "AlliGator Set Phasor Plot Update LED.vi"("error in (no error)"=w890, "Off/On"=TRUE) -> ("error out"=w888:errorcluster)  [unwired: 9 in]
              }
            }
            n388 = Merge Errors(w886, w877) -> (w878:errorcluster)
          }
          frame "Phasor Graph Frequency" {
            # "Need to update TWO controls"
            n389 = control-ref of="Phasor Plot Frequency"() -> (w899:refnum<vi>)
            n390 = Variant To Data(error in=w895, type=dbl[unit] 0.0 ("Phasor Plot Frequency"), Variant=w896) -> (data=w891:dbl[unit], error out=w894:errorcluster)
            n391 = call "Alligator Variables Storage.vi"("AlliGator Variable"=AlliGator_Variables_List."Phasor Plot:Computed" ("Alligator Variable"), "Error In"=w895) -> ("Error Out"=w893:errorcluster, "Data out"=w903:variant)  [unwired: 7 in, 1 out]
            n392 = call-poly "Variant to Data.vi"("Variant"=w903) -> ("Value"=w902:bool)  [unwired: 8 in]
            n393 = local write "Phasor Plot Frequency"(w891) -> ()
            n394 = call "AlliGator Update Settings & Control.vi"("Error In"=w894, "Value"=w891, "Sender"=w900, "CtlRef"=w899) -> ("Error Out"=w897:errorcluster)  [unwired: 7 in]
            n395 = case shown="True" w902 {
              tunnel: w893 -> [w906 w909]
              tunnel: [w906 w907] -> w905
              frame False {
              }
              frame True {
                n396 = call "AlliGator Set Phasor Plot Update LED.vi"("error in (no error)"=w909, "Off/On"=TRUE) -> ("error out"=w907:errorcluster)  [unwired: 9 in]
              }
            }
            n397 = Merge Errors(w905, w897) -> (w898:errorcluster)
          }
        }
        n398 = call "AlliGator Update Settings & Control.vi"("Error In"=w854, "Value"=w850, "Sender"=w851, "CtlRef"=w843) -> ("Error Out"=w847:errorcluster)  [unwired: 7 in]
        n399 = call "AlliGator Get Control Notebook String.vi"("error in (no error)"=w847, "Value"=w850, "Control Label"=w842) -> ("error out"=w845:errorcluster, "Notebook String"=w844:string)  [unwired: 7 in]
      }
      event "Phasor Graph Frequency", "Phasor Plot Frequency": Shortcut Menu Selection (User) {
        n400 = event-data() -> ("CtlRef"=w916:refnum<vi>, "ItemTag"=w915:string)  [unwired: 1 in]
        n401 = case shown="\"f = 1/D\"" w915 {
          tunnel: w916 -> [_ w918 w921 w924 w928]
          tunnel: [_ w917 w919 w922 w925] -> w910
          frame "", Default {
          }
          frame "f = 1/T" {
            n402 = call "AlliGator Set Phasor Harmonic.vi"("Phasor Frequency Refnum"=w918) -> ("Error Out"=w917:errorcluster)  [unwired: 10 in]
          }
          frame "f = 1/D" {
            n403 = call "AlliGator Set Phasor Harmonic.vi"("Use n/D"=TRUE, "Phasor Frequency Refnum"=w921) -> ("Error Out"=w919:errorcluster)  [unwired: 9 in]
          }
          frame "f = n/T (n > 1)" {
            n404 = call "AlliGator Set Phasor Harmonic.vi"("Harmonic (1)"=0, "Phasor Frequency Refnum"=w924) -> ("Error Out"=w922:errorcluster)  [unwired: 9 in]
          }
          frame "f = n/D (n > 1)" {
            n405 = call "AlliGator Set Phasor Harmonic.vi"("Use n/D"=TRUE, "Harmonic (1)"=0, "Phasor Frequency Refnum"=w928) -> ("Error Out"=w925:errorcluster)  [unwired: 8 in]
          }
        }
      }
      event "Phasor Graph": Cursor Move {
        n406 = event-data() -> ("Time"=w929:u32)  [unwired: 1 in]
        n407 = case shown="True" w930 {
          tunnel: [_ w939] -> w931
          tunnel: w929 -> [_ w937]
          frame False {
          }
          frame True {
            w938 = T26 {"AlliGator Q Event"=enum."Phasor Graph:Cursor Move", "Data"=variant} ("Time-Gated Phasor Q Element")
            n408 = call "AlliGator Filter Event.vi"("Time"=w937, "Time-Gated Phasor Q Element"=w938) -> ("Filter Event?"=w936:bool)  [unwired: 8 in, 1 out]
            n409 = case shown="False" w936 {
              tunnel: w938 -> [w941 _]
              tunnel: [w940 _] -> w939
              frame False {
                n410 = Build Array(w941) -> (w940:T26[])
              }
              frame True {
              }
            }
          }
        }
      }
      event "Phasor Graph": Scale Range Change; "Phasor Graph": Autoscale Range Change; "Phasor Graph": Cursor Release {
        n411 = event-data() -> ()  [unwired: 1 in, 1 out]
        n412 = case shown="True" w947 {
          tunnel: [_ T26[] [{"AlliGator Q Event"=enum."Phasor Graph:Draw Cursor Connecting Line", "Data"=variant}] ("element")] -> w942
          frame False {
          }
          frame True {
          }
        }
      }
      event "Phasor Graph": Shortcut Menu Selection (User) {
        n413 = event-data() -> ("CtlRef"=w960:refnum<vi>, "Coords"=w959:T37, "ItemTag"=w958:string, "ItemPath"=w957:string)  [unwired: 1 in]
        n414 = call-poly <vilib>:"Acquire Input Data.vi"("device ID"=w955, "error in (no error)"=w956) -> ("device ID"=w954:refnum<k1>, "keys pressed"=w952:T52, "error out"=w953:errorcluster)  [unwired: 15 in]
        n415 = case shown="True" w961 {
          tunnel: w960 -> [_ w976]
          tunnel: w959 -> [_ w975]
          tunnel: w958 -> [_ w974]
          tunnel: w957 -> [_ w973]
          tunnel: w952 -> [_ w969]
          tunnel: [_ w966] -> w951
          tunnel: [_ w965] -> w950
          tunnel: [_ w964] -> w949
          frame False {
          }
          frame True {
            n416 = Index Array(array=w969) -> (element=w968:T34)  [unwired: 1 in]
            n417 = Equal?(x=w968, y=T34."H" ("element")) -> (x = y?=w967:bool)
            n418 = Bundle By Name(cluster=T39 {"Item Tag"="", "XY Graph Refnum"=refnum, "Coords"={"Horizontal"=0, "Vertical"=0}, "Item Path"=""} ("XY Graph Event"), "XY Graph Refnum"=w976, "Coords"=w975, "Item Tag"=w974, "Item Path"=w973) -> (w972:T39)
            n419 = call "AlliGator Phasor Graph Context Menu Handler.vi"("Help?"=w967, "XY Graph Event"=w972) -> ("Error Out"=w965:errorcluster, "Message"=w966:string, "AlliGator Actions"=w964:T26[])  [unwired: 7 in]
          }
        }
      }
      event "Phasor Plot Active": Value Change {
        n420 = event-data() -> ("NewVal"=w984:bool)  [unwired: 1 in]
        n421 = call "AlliGator Settings Storage.vi"("Get(F)/Set"=TRUE, "AlliGator Settings List"=AlliGator_Settings_List."Phasor Plot:Phasor Plot Active", "Variant Data in"=w984) -> ("Error Out"=w977:errorcluster)  [unwired: 7 in, 1 out]
      }
      event "Phasor Plot Color Scale", "Decay Fit Parameter Map Color Scale", "Image Color Scale": Shortcut Menu Activation? {
        w991 = string[] ["Copy Color Scale to Clipboard"] ("item names")
        n422 = event-data() -> ("MenuRef"=w993:refnum<k9>)  [unwired: 1 in]
        n423 = Delete Menu Items(9:w993) -> (0:w986:errorcluster, 3:w992:refnum<k9>)  [unwired: 3 in]
        n424 = Insert Menu Items(6:w986, 7:w991, 8:w991, 9:w992) -> (0:w985:errorcluster)  [unwired: 2 in, 2 out]
        n425 = event-data() -> ()  [unwired: 2 in, 1 out]
      }
      event "Phasor Plot Color Scale", "Image Color Scale", "Decay Fit Parameter Map Color Scale": Shortcut Menu Selection (User) {
        n426 = event-data() -> ("CtlRef"=w998:refnum<vi>, "ItemTag"=w999:string)  [unwired: 1 in]
        n427 = case shown="\"Copy Color Scale to Clipboard\"" w999 {
          tunnel: w998 -> [_ w1000]
          frame "", Default {
          }
          frame "Copy Color Scale to Clipboard" {
            n428 = call "Export Color Ramp to Clipboard.vi"("ColorRamp in"=w1000) -> ()  [unwired: 11 in]
          }
        }
      }
      event "Phasor Plot Color Scale": Mouse Up {
        n429 = event-data() -> ()  [unwired: 1 in, 1 out]
        n430 = case shown="True" w1006 {
          tunnel: [_ w1007] -> w1001
          frame False {
          }
          frame True {
            n431 = Bundle By Name(cluster=T26 {"AlliGator Q Event"=enum."Phasor Plot:Change Phasor Plot Color Palette", "Data"=variant} ("element"), "Data"="Refresh Image" ("String")) -> (w1009:T26)
            n432 = Build Array(w1009) -> (w1007:T26[])
          }
        }
      }
      event "Phasor Plot Image": Shortcut Menu Activation? {
        w1024 = AlliGator_Variables_List."Phasor Plot:Phasor Ratio Palette List" ("Alligator Variable")
        n433 = event-data() -> ("CtlRef"=w1012:refnum<vi>, "MenuRef"=w1038:refnum<k9>)  [unwired: 1 in]
        n434 = call "Alligator Variables Storage.vi"("Get(F)/Set"=FALSE, "AlliGator Variable"=AlliGator_Variables_List."Phasor Plot:Palette Information" ("Alligator Variable")) -> ("Error Out"=w1034:errorcluster, "Data out"=w1035:variant)  [unwired: 7 in, 1 out]
        n435 = call "Alligator Variables Storage.vi"("Get(F)/Set"=FALSE, "AlliGator Variable"=w1024) -> ("Error Out"=w1015:errorcluster, "Data out"=w1028:variant)  [unwired: 7 in, 1 out]
        n436 = Variant To Data(error in=w1034, type=T31 {"Palette Name [# Colors,int?,inv?]"="", "Palette Type"=0, "Palette Colors"=[], "Interpolate?"=FALSE} ("Image Display Palette Information"), Variant=w1035) -> (data=w1033:T31, error out=w1032:errorcluster)
        n437 = call-poly "Variant to Data.vi"("Variant"=w1028) -> ("String Array"=w1027:string[])  [unwired: 8 in]
        n438 = Unbundle By Name(w1033) -> ("Palette Name [# Colors,int?,inv?]"=w1030:string)
        n439 = Merge Errors(w1032, w1015) -> (w1016:errorcluster)
        n440 = call "Check Selected Palette in Menu.vi"("Error In"=w1016, "Palette List"=w1027, "Checked Palette"=w1030, "Menu in"=w1038) -> ("Error Out"=w1023:errorcluster, "Stored Palette List"=w1025:string[], "menu reference out"=w1022:refnum<k9>)  [unwired: 5 in]
        n441 = call "Alligator Variables Storage.vi"("Get(F)/Set"=TRUE, "AlliGator Variable"=w1024, "Error In"=w1023, "Data in"=w1025) -> ("Error Out"=w1021:errorcluster)  [unwired: 5 in, 2 out]
        n442 = call "AlliGator Show-Hide Phasor Plot Menu Items.vi"("error in (no error)"=w1021, "Menu in"=w1022) -> ("error out"=w1014:errorcluster, "Menu out"=w1011:refnum<k9>)  [unwired: 8 in]
        n443 = call "AlliGator Add Python Functions to Object Menu.vi"("error in (no error)"=w1014, "Menu in"=w1011, "Object Refnum"=w1012) -> ("error out"=w1013:errorcluster)  [unwired: 6 in, 2 out]
        n444 = event-data() -> ()  [unwired: 2 in, 1 out]
      }
      event "Phasor Plot Image": Shortcut Menu Selection (User) {
        n445 = event-data() -> ("CtlRef"=w1051:refnum<vi>, "ItemTag"=w1048:string, "ItemPath"=w1052:string, "Coords"=w1053:T37)  [unwired: 1 in]
        n446 = call-poly <vilib>:"Acquire Input Data.vi"("device ID"=w1044, "error in (no error)"=w1045) -> ("device ID"=w1043:refnum<k1>, "keys pressed"=w1042:T52, "error out"=w1041:errorcluster)  [unwired: 15 in]
        n447 = case shown="True" w1047 {
          tunnel: w1053 -> [_ w1064]
          tunnel: w1052 -> [_ w1063]
          tunnel: w1051 -> [_ w1062]
          tunnel: w1048 -> [_ w1061]
          tunnel: [_ w1060] -> w1046
          tunnel: w1042 -> [_ w1056]
          tunnel: [_ w1055] -> w1040
          tunnel: [_ w1054] -> w1039
          frame False {
          }
          frame True {
            n448 = Index Array(array=w1056) -> (element=w1059:T34)  [unwired: 1 in]
            n449 = Equal?(x=w1059, y=T34."H" ("element")) -> (x = y?=w1057:bool)
            n450 = case shown="False" w1057 {
              tunnel: w1064 -> [w1073 _]
              tunnel: w1063 -> [w1072 _]
              tunnel: w1062 -> [w1071 w1077]
              tunnel: w1061 -> [w1070 w1076]
              tunnel: [w1069 _] -> w1060
              tunnel: [w1066 w1075] -> w1055
              tunnel: [w1065 w1074] -> w1054
              frame False {
                n451 = Bundle By Name(cluster=T35 {"Item Tag"="", "Image Control Refnum"=refnum, "Coords"={"Horizontal"=0, "Vertical"=0}, "Item Path"=""} ("Image Event Data"), "Image Control Refnum"=w1071, "Item Tag"=w1070, "Item Path"=w1072, "Coords"=w1073) -> (w1067:T35)
                n452 = call "AlliGator Phasor Plot Context Menu Handler.vi"("Image Event"=w1067) -> ("Error Out"=w1065:errorcluster, "Message"=w1066:string, "AlliGator Actions"=w1069:T26[])  [unwired: 8 in]
              }
              frame True {
                n453 = property class="ImageControl"(reference=w1077) -> ("Label.Text"=w1078:string)  [unwired: 1 in, 2 out]
                n454 = call "AlliGator Send Python Function Doc String to Notebook.vi"("Item Tag"=w1076, "Target"=w1078) -> ("Error Out"=w1074:errorcluster, "Message"=w1075:string)  [unwired: 8 in]
              }
            }
          }
        }
      }
      event "Phasor Plot ROI Color": Value Change {
        n455 = event-data() -> ("NewVal"=w1079:u32)  [unwired: 1 in]
        n456 = call <vilib>:"Color to RGB.vi"("Color"=w1079) -> ("R"=w1082:u8, "G"=w1083:u8, "B"=w1084:u8)  [unwired: 1 out]
        n457 = Bundle By Name(cluster=cluster{"Red":u8, "Green":u8, "Blue":u8} {"Red"=0, "Green"=0, "Blue"=0} ("ROI Color"), "Red"=w1082, "Green"=w1083, "Blue"=w1084) -> (w1081:cluster{"Red":u8, "Green":u8, "Blue":u8})
        n458 = property on="Phasor Plot Image" class="ImageControl"("ROI Color"=w1081) -> ()  [unwired: 2 in, 2 out]
      }
      event "Phasor Ratio Graph", "Decay Graph", "Phasor Graph", "Lifetime & Other Parameters Graph", "Decay Statistics Graph": event #0x4e {
        # "Change style of new cursor to a more visible one"
        n459 = event-data() -> ("ItemTag"=w1091:string, "CtlRef"=w1090:refnum<vi>)  [unwired: 1 in]
        n460 = case shown="\"CURS_FREE\", \"CURS_MULTI\", \"CURS_SINGLE\"" w1091 {
          tunnel: w1090 -> [_ w1096]
          tunnel: [_ w1098] -> w1089
          frame "", Default {
          }
          frame "CURS_FREE", "CURS_MULTI", "CURS_SINGLE" {
            n461 = Bundle By Name(cluster=T26 {"AlliGator Q Event"=enum."Generic Graph:Set Last Cursor Style", "Data"=variant} ("AlliGator Actions"), "Data"=w1096) -> (w1097:T26)
            n462 = Build Array(w1097) -> (w1098:T26[])
          }
        }
      }
      event "Phasor Ratio Graph": Shortcut Menu Selection (User) {
        n463 = event-data() -> ("ItemPath"=w1101:string, "CtlRef"=w1111:refnum<vi>, "Coords"=w1110:T37, "ItemTag"=w1102:string)  [unwired: 1 in]
        n464 = Select(t=w1102, s=w1109, f=w1107) -> (s? t:f=w1108:string)
        n465 = case shown="\"New Plot\"" w1108 {
          selector: w1108 -> [_ w1114 _ _ _]
          tunnel: w1111 -> [_ w1116 _ _ w1135]
          tunnel: w1110 -> [_ w1115 _ _ w1134]
          tunnel: w1101 -> [_ w1113 _ _ _]
          tunnel: [_ w1112 _ w1122 w1133] -> w1100
          frame "", "Busy" {
          }
          frame Default {
            n466 = Bundle By Name(cluster=T39 {"Item Tag"="", "XY Graph Refnum"=refnum, "Coords"={"Horizontal"=0, "Vertical"=0}, "Item Path"=""} ("XY Graph Event"), "Item Path"=w1113, "XY Graph Refnum"=w1116, "Coords"=w1115, "Item Tag"=w1114) -> (w1119:T39)
            n467 = Bundle By Name(cluster=T26 {"AlliGator Q Event"=enum."Generic Graph:Generic XY Graph Event", "Data"=variant} ("element"), "Data"=w1119) -> (w1117:T26)
            n468 = Build Array(w1117) -> (w1112:T26[])
          }
          frame "-----------------" {
          }
          frame "New Plot" {
            w1121 = T53 {"Multiplot XY Graph"=refnum, "Plot Name"="", "Plot Scales"={"X Scale"=0, "Y Scale"=0}, "Plot Interpolation"=enum."Use Previous Plot's Style", "Point Style"=enum."not defined", "Plot Color"=15781887, "Plot Metadata"=variant} ("New Plot Information")
            w1126 = T26 {"AlliGator Q Event"=enum."Generic Graph:New Plot", "Data"=variant} ("Time-Gated Phasor Q Element")
            n469 = control-ref of="Lifetime & Other Parameters Graph"() -> (w1123:refnum<vi>)
            n470 = control-ref of="Phasor Ratio Graph"() -> (w1124:refnum<vi>)
            n471 = Bundle By Name(cluster=w1121, "Multiplot XY Graph"=w1124, "Plot Name"="Phasor Ratio") -> (w1130:T53)
            n472 = Bundle By Name(cluster=w1121, "Multiplot XY Graph"=w1123, "Plot Name"="Lifetime") -> (w1127:T53)
            n473 = Bundle By Name(cluster=w1126, "Data"=w1130) -> (w1131:T26)
            n474 = Bundle By Name(cluster=w1126, "Data"=w1127) -> (w1125:T26)
            n475 = Build Array(w1131, w1125) -> (w1122:T26[])
          }
          frame "Linear Fit" {
            n476 = Bundle(cluster=T41 {"Multiplot XY Graph"=refnum, "Mouse Coordinates"={"Horizontal"=0, "Vertical"=0}} ("Mouse Click Event Data"), "Multiplot XY Graph"=w1135, "Mouse Coordinates"=w1134) -> (w1137:T41)
            n477 = Bundle By Name(cluster=T26 {"AlliGator Q Event"=enum."Phasor Ratio:Fit Line to Phasor Ratio Plot", "Data"=variant} ("Time-Gated Phasor Q Element"), "Data"=w1137) -> (w1138:T26)
            n478 = Build Array(w1138) -> (w1133:T26[])
          }
        }
      }
      event "Phasor Reference 1 Control": Value Change {
        n479 = event-data() -> ("CtlRef"=w1145:refnum<vi>, "OldVal"=w1144:dbl, "NewVal"=w1147:dbl)  [unwired: 1 in]
        n480 = case shown="True" w1146 {
          tunnel: w1148 -> [_ _]
          tunnel: w1147 -> [_ w1153]
          tunnel: w1145 -> [w1150 _]
          tunnel: w1144 -> [w1149 _]
          tunnel: [_ w1151] -> w1139
          frame False {
            n481 = property class="Scroll (strict)"(reference=w1150, "Value"=w1149) -> ()  [unwired: 1 in, 2 out]
          }
          frame True {
            n482 = Bundle By Name(cluster=T26 {"AlliGator Q Event"=enum."Phasor Ratio:Update Phasor Reference 1", "Data"=variant} ("Time-Gated Phasor Q Element"), "Data"=w1153) -> (w1154:T26)
            n483 = Build Array(w1154, T26 {"AlliGator Q Event"=enum."Phasor Graph:Draw Cursor Connecting Line", "Data"=variant} ("Time-Gated Phasor Q Element")) -> (w1151:T26[])
          }
        }
      }
      event "Phasor Reference 2 Control": Value Change {
        n484 = event-data() -> ("CtlRef"=w1162:refnum<vi>, "OldVal"=w1161:dbl, "NewVal"=w1164:dbl)  [unwired: 1 in]
        n485 = case shown="True" w1163 {
          tunnel: w1165 -> [_ _]
          tunnel: w1164 -> [_ w1170]
          tunnel: w1162 -> [w1167 _]
          tunnel: w1161 -> [w1166 _]
          tunnel: [_ w1168] -> w1156
          frame False {
            n486 = property class="Scroll (strict)"(reference=w1167, "Value"=w1166) -> ()  [unwired: 1 in, 2 out]
          }
          frame True {
            n487 = Bundle By Name(cluster=T26 {"AlliGator Q Event"=enum."Phasor Ratio:Update Phasor Reference 2", "Data"=variant} ("Time-Gated Phasor Q Element"), "Data"=w1170) -> (w1171:T26)
            n488 = Build Array(w1171, T26 {"AlliGator Q Event"=enum."Phasor Graph:Draw Cursor Connecting Line", "Data"=variant} ("Time-Gated Phasor Q Element")) -> (w1168:T26[])
          }
        }
      }
      event "Phasor ROI Decay": Value Change {
        n489 = event-data() -> ()  [unwired: 1 in, 1 out]
        n490 = case shown="True" w1173 {
          tunnel: [_ T26[] [{"AlliGator Q Event"=enum."Phasor Plot:Compute Decay of Selected Phasors", "Data"=variant}] ("element")] -> w1174
          frame False {
          }
          frame True {
          }
        }
      }
      event "Refresh Decay Fit Parameter Map": Value Change {
        n491 = event-data() -> ()  [unwired: 1 in, 1 out]
        n492 = case shown="True" w1185 {
          tunnel: w1186 -> [_ _]
          tunnel: [_ w1187] -> w1180
          frame False {
          }
          frame True {
            w1190 = TRUE  # Parameter changed
            n493 = local read "Decay Fit Parameter"() -> (w1189:T11)
            n494 = Bundle(cluster=T38 {"Parameter"=enum."Offset", "Parameter changed"=FALSE} ("output cluster"), "Parameter"=w1189, "Parameter changed"=w1190) -> (w1188:T38)
            n495 = Bundle By Name(cluster=T26 {"AlliGator Q Event"=enum."Decay Fit Parameter Map:Build Decay Fit Parameter Map", "Data"=variant} ("Time-Gated Phasor Q Element"), "Data"=w1188) -> (w1192:T26)
            n496 = Build Array(w1192) -> (w1187:T26[])
          }
        }
      }
      event "Refresh Image": Value Change {
        n497 = event-data() -> ()  [unwired: 1 in, 1 out]
        n498 = case shown="True" w1199 {
          tunnel: w1200 -> [_ _]
          tunnel: [_ w1201] -> w1194
          frame False {
          }
          frame True {
            n499 = Build Array(T26 {"AlliGator Q Event"=enum."Files:New Folder Selected", "Data"=variant} ("Time-Gated Phasor Q Element")) -> (w1201:T26[])
          }
        }
      }
      event "Refresh Parameter Map": Value Change {
        n500 = event-data() -> ()  [unwired: 1 in, 1 out]
        n501 = case shown="True" w1208 {
          tunnel: w1209 -> [_ _]
          tunnel: [_ w1211] -> w1203
          frame False {
          }
          frame True {
            w1214 = TRUE  # Parameter changed
            n502 = local read "Parameter Map Set"() -> (w1210:u16)
            n503 = local read "Map Parameter"() -> (w1213:u16)
            n504 = Bundle By Name(cluster=T43 {"Parameter"=0, "Parameter changed"=FALSE, "Map Set"=0} ("output cluster"), "Parameter"=w1213, "Parameter changed"=w1214, "Map Set"=w1210) -> (w1212:T43)
            n505 = Bundle By Name(cluster=T26 {"AlliGator Q Event"=enum."Parameter Map:Build Parameter Map", "Data"=variant} ("Time-Gated Phasor Q Element"), "Data"=w1212) -> (w1216:T26)
            n506 = Build Array(w1216) -> (w1211:T26[])
          }
        }
      }
      event "Refresh Phasor Plot": Shortcut Menu Activation? {
        n507 = event-data() -> ("MenuRef"=w1223:refnum<k9>)  [unwired: 1 in]
        n508 = call "AlliGator Set Checks in Phasor Update Button.vi"("Menu in"=w1223) -> ("Error Out"=w1218:errorcluster)  [unwired: 10 in]
        n509 = event-data() -> ()  [unwired: 2 in, 1 out]
      }
      event "Refresh Phasor Plot": Shortcut Menu Selection (User) {
        n510 = event-data() -> ("ItemTag"=w1230:string, "CtlRef"=w1224:refnum<vi>)  [unwired: 1 in]
        n511 = call "AlliGator Update Phasor Image Elements to Update.vi"("CtlRef"=w1224, "Phasor Plot Element to Update"=w1230) -> ("Error Out"=w1225:errorcluster)  [unwired: 8 in, 1 out]
      }
      event "Refresh Phasor Plot": Value Change {
        n512 = event-data() -> ()  [unwired: 1 in, 1 out]
        n513 = case shown="True" w1236 {
          tunnel: [_ w1237] -> w1231
          frame False {
          }
          frame True {
            n514 = Build Array(T26 {"AlliGator Q Event"=enum."Phasor Plot:Build Phasor Plot", "Data"=variant} ("Time-Gated Phasor Q Element")) -> (w1237:T26[])
          }
        }
      }
      event "Refresh SEPL": Value Change {
        n515 = event-data() -> ()  [unwired: 1 in, 1 out]
        n516 = case shown="True" w1244 {
          tunnel: [_ w1245] -> w1239
          frame False {
          }
          frame True {
            n517 = Build Array(T26 {"AlliGator Q Event"=enum."Phasor Graph:Update SEPL Plot", "Data"=variant} ("element")) -> (w1245:T26[])
          }
        }
      }
      event "Scale Bar": Value Change {
        n518 = event-data() -> ()  [unwired: 1 in, 1 out]
        n519 = case shown="True" w1252 {
          tunnel: [_ w1253] -> w1247
          frame False {
          }
          frame True {
            n520 = Build Array(T26 {"AlliGator Q Event"=enum."Image:Add Scale Bar Overlay", "Data"=variant} ("element")) -> (w1253:T26[])
          }
        }
      }
      event "Show Line": Value Change {
        n521 = event-data() -> ("CtlRef"=w1265:refnum<vi>, "NewVal"=w1263:bool, "OldVal"=w1261:bool)  [unwired: 1 in]
        n522 = case shown="True" w1262 {
          tunnel: w1265 -> [w1268 _]
          tunnel: w1264 -> [_ _]
          tunnel: w1263 -> [_ w1271]
          tunnel: w1261 -> [w1267 _]
          tunnel: [w1266 w1270] -> w1256
          tunnel: [_ w1272] -> w1255
          frame False {
            n523 = property class="Bool (strict)"(reference=w1268, "Value"=w1267) -> (error out=w1266:errorcluster)  [unwired: 1 in, 1 out]
          }
          frame True {
            n524 = call "Alligator Variables Storage.vi"("AlliGator Variable"=AlliGator_Variables_List."Phasor Graph:Show Line", "Data in"=w1271) -> ("Error Out"=w1270:errorcluster)  [unwired: 7 in, 2 out]
            n525 = Build Array(T26 {"AlliGator Q Event"=enum."Phasor Graph:Draw Cursor Connecting Line", "Data"=variant} ("Time-Gated Phasor Q Element"), T26 {"AlliGator Q Event"=enum."Phasor Graph:Find UC Intersection", "Data"=variant} ("Time-Gated Phasor Q Element")) -> (w1274:T26[])
            n526 = Select(t=w1274, s=w1271, f=T26[] [{"AlliGator Q Event"=enum."Phasor Graph:Clear Cursor Connecting Line", "Data"=variant}] ("element")) -> (s? t:f=w1272:T26[])
          }
        }
      }
      event "Single Step Phasor": Value Change {
        n527 = event-data() -> ("CtlRef"=w1283:refnum<vi>, "NewVal"=w1285:bool, "OldVal"=w1282:bool)  [unwired: 1 in]
        n528 = case shown="True" w1284 {
          tunnel: w1285 -> [_ w1293]
          tunnel: w1283 -> [w1287 _]
          tunnel: w1282 -> [w1286 _]
          tunnel: [_ w1288] -> w1277
          frame False {
            n529 = property class="Bool (strict)"(reference=w1287, "Value"=w1286) -> ()  [unwired: 1 in, 2 out]
          }
          frame True {
            n530 = property on="Phasor Frame Slide" class="Slide (strict)"("Visible"=w1293) -> ("Value"=w1292:i32)  [unwired: 2 in, 2 out]
            n531 = Select(t=w1292, s=w1293, f=0) -> (s? t:f=w1290:i32)
            n532 = Decrement(x=w1290) -> (x-1=w1289:i32)
            n533 = Bundle By Name(cluster=T26 {"AlliGator Q Event"=enum."Phasor Graph:Show Single Phasor", "Data"=variant} ("element"), "Data"=w1289) -> (w1294:T26)
            n534 = Build Array(w1294) -> (w1288:T26[])
          }
        }
      }
      event "Source Image ROI Color": Value Change {
        n535 = event-data() -> ("NewVal"=w1296:u32)  [unwired: 1 in]
        n536 = call <vilib>:"Color to RGB.vi"("Color"=w1296) -> ("R"=w1299:u8, "G"=w1300:u8, "B"=w1301:u8)  [unwired: 1 out]
        n537 = Bundle By Name(cluster=cluster{"Red":u8, "Green":u8, "Blue":u8} {"Red"=0, "Green"=0, "Blue"=0} ("ROI Color"), "Red"=w1299, "Green"=w1300, "Blue"=w1301) -> (w1298:cluster{"Red":u8, "Green":u8, "Blue":u8})
        n538 = property on="Source Image" class="ImageControl"("ROI Color"=w1298) -> ()  [unwired: 2 in, 2 out]
      }
      event "Source Image ROI Selection": Value Change {
        n539 = event-data() -> ("CtlRef"=w1312:refnum<vi>, "OldVal"=w1311:i32, "NewVal"=w1315:i32)  [unwired: 1 in]
        n540 = Subtract(x=w1311, y=w1315) -> (x-y=w1314:i32)
        n541 = case shown="True" w1313 {
          tunnel: w1314 -> [_ w1319]
          tunnel: w1312 -> [w1317 _]
          tunnel: w1311 -> [w1316 _]
          tunnel: [_ w1318] -> w1306
          frame False {
            n542 = property class="Scroll (strict)"(reference=w1317, "Value"=w1316) -> ()  [unwired: 1 in, 2 out]
          }
          frame True {
            n543 = case shown="..-1" w1319 {
              tunnel: [_ w1320 w1326] -> w1318
              frame 0, Default {
              }
              frame 1.. {
                n544 = Bundle("Action"=AlliGator_ROI_Manager_Actions."Select Previous ROI", -1) -> (w1322:cluster{"Action":T44, i32})  [unwired: 1 in]
                n545 = Bundle By Name(cluster=T26 {"AlliGator Q Event"=enum."Image:Source Image ROI Selection", "Data"=variant} ("Time-Gated Phasor Q Element"), "Data"=w1322) -> (w1324:T26)
                n546 = Build Array(w1324) -> (w1320:T26[])
              }
              frame ..-1 {
                n547 = Bundle("Action"=AlliGator_ROI_Manager_Actions."Select Next ROI", -1) -> (w1328:cluster{"Action":T44, i32})  [unwired: 1 in]
                n548 = Bundle By Name(cluster=T26 {"AlliGator Q Event"=enum."Image:Source Image ROI Selection", "Data"=variant} ("Time-Gated Phasor Q Element"), "Data"=w1328) -> (w1330:T26)
                n549 = Build Array(w1330) -> (w1326:T26[])
              }
            }
          }
        }
      }
      event "Source Image", "Phasor Plot Image", "Decay Fit Parameter Map Image", "Parameter Map Image": Mouse Wheel {
        n550 = event-data() -> ("CtlRef"=w1337:refnum<vi>, "Delta"=w1336:i32)  [unwired: 1 in]
        n551 = call "Image Display Mouse Wheel Zoom.vi"("Mouse Wheel Delta"=w1336, "Image Control Refnum"=w1337) -> ()  [unwired: 9 in, 1 out]
      }
      event "Source Image": Shortcut Menu Activation? {
        w1349 = AlliGator_Variables_List."Source Image:Palette List" ("Alligator Variable")
        n552 = event-data() -> ("CtlRef"=w1340:refnum<vi>, "MenuRef"=w1363:refnum<k9>)  [unwired: 1 in]
        n553 = call "Alligator Variables Storage.vi"("Get(F)/Set"=FALSE, "AlliGator Variable"=AlliGator_Variables_List."X_Source Image:Palette Information" ("Alligator Variable")) -> ("Error Out"=w1359:errorcluster, "Data out"=w1360:variant)  [unwired: 7 in, 1 out]
        n554 = call "Alligator Variables Storage.vi"("Get(F)/Set"=FALSE, "AlliGator Variable"=w1349) -> ("Error Out"=w1342:errorcluster, "Data out"=w1353:variant)  [unwired: 7 in, 1 out]
        n555 = Variant To Data(error in=w1359, type=T31 {"Palette Name [# Colors,int?,inv?]"="", "Palette Type"=0, "Palette Colors"=[], "Interpolate?"=FALSE} ("Image Display Palette Information"), Variant=w1360) -> (data=w1358:T31, error out=w1357:errorcluster)
        n556 = call-poly "Variant to Data.vi"("Variant"=w1353) -> ("String Array"=w1352:string[])  [unwired: 8 in]
        n557 = Unbundle By Name(w1358) -> ("Palette Name [# Colors,int?,inv?]"=w1355:string)
        n558 = Merge Errors(w1357, w1342) -> (w1343:errorcluster)
        n559 = call "Check Selected Palette in Menu.vi"("Error In"=w1343, "Palette List"=w1352, "Checked Palette"=w1355, "Menu in"=w1363) -> ("Error Out"=w1344:errorcluster, "Stored Palette List"=w1350:string[], "menu reference out"=w1339:refnum<k9>)  [unwired: 5 in]
        n560 = call "Alligator Variables Storage.vi"("Get(F)/Set"=TRUE, "AlliGator Variable"=w1349, "Error In"=w1344, "Data in"=w1350) -> ("Error Out"=w1341:errorcluster)  [unwired: 5 in, 2 out]
        n561 = call "AlliGator Add Python Functions to Object Menu.vi"("error in (no error)"=w1341, "Menu in"=w1339, "Object Refnum"=w1340) -> ("error out"=w1338:errorcluster)  [unwired: 6 in, 2 out]
        n562 = event-data() -> ()  [unwired: 2 in, 1 out]
      }
      event "Source Image": Shortcut Menu Selection (User) {
        n563 = event-data() -> ("CtlRef"=w1378:refnum<vi>, "ItemTag"=w1374:string, "ItemPath"=w1377:string, "Coords"=w1372:T37)  [unwired: 1 in]
        n564 = call-poly <vilib>:"Acquire Input Data.vi"("device ID"=w1370, "error in (no error)"=w1368) -> ("device ID"=w1371:refnum<k1>, "keys pressed"=w1367:T52, "error out"=w1369:errorcluster)  [unwired: 15 in]
        n565 = case shown="True" w1373 {
          tunnel: w1378 -> [_ w1383]
          tunnel: w1377 -> [_ w1389]
          tunnel: w1374 -> [_ w1387]
          tunnel: w1372 -> [_ w1388]
          tunnel: w1367 -> [_ w1386]
          tunnel: [_ w1381] -> w1366
          tunnel: [_ w1380] -> w1365
          tunnel: [_ w1379] -> w1364
          frame False {
          }
          frame True {
            n566 = Index Array(array=w1386) -> (element=w1385:T34)  [unwired: 1 in]
            n567 = Equal?(x=w1385, y=T34."H" ("element")) -> (x = y?=w1382:bool)
            n568 = case shown="False" w1382 {
              tunnel: w1389 -> [w1397 _]
              tunnel: w1388 -> [w1396 _]
              tunnel: w1387 -> [w1394 w1400]
              tunnel: w1383 -> [w1393 w1402]
              tunnel: [w1391 _] -> w1381
              tunnel: [_ w1399] -> w1380
              tunnel: [w1390 w1398] -> w1379
              frame False {
                n569 = Bundle By Name(cluster=T35 {"Item Tag"="", "Image Control Refnum"=refnum, "Coords"={"Horizontal"=0, "Vertical"=0}, "Item Path"=""} ("Image Event"), "Image Control Refnum"=w1393, "Item Tag"=w1394, "Item Path"=w1397, "Coords"=w1396) -> (w1392:T35)
                n570 = call "AlliGator Source Image Context Menu Handler.vi"("Image Event Data"=w1392) -> ("Error Out"=w1390:errorcluster, "AlliGator Actions"=w1391:T26[])  [unwired: 9 in]
              }
              frame True {
                n571 = property class="ImageControl"(reference=w1402) -> ("Label.Text"=w1401:string)  [unwired: 1 in, 2 out]
                n572 = call "AlliGator Send Python Function Doc String to Notebook.vi"("Item Tag"=w1400, "Target"=w1401) -> ("Error Out"=w1398:errorcluster, "Message"=w1399:string)  [unwired: 8 in]
              }
            }
          }
        }
      }
      event "Time Point Slide": Value Change {
        # "Time Point Slider: Mouse Up, Mouse Leave"
        n573 = event-data() -> ("CtlRef"=w1410:refnum<vi>, "OldVal"=w1403:u16)  [unwired: 1 in]
        n574 = case shown="True" w1411 {
          tunnel: w1410 -> [w1414 w1418]
          tunnel: [w1412 w1415] -> w1405
          tunnel: [_ w1416] -> w1404
          tunnel: w1403 -> [w1413 _]
          frame False {
            n575 = property class="Slide (strict)"(reference=w1414, "Value"=w1413) -> (error out=w1412:errorcluster)  [unwired: 1 in, 1 out]
          }
          frame True {
            n576 = property class="Slide (strict)"(reference=w1418) -> (error out=w1415:errorcluster, "Value"=w1417:u16)  [unwired: 1 in, 1 out]
            n577 = Bundle By Name(cluster=T26 {"AlliGator Q Event"=enum."GUI:Time Series Slider Changed", "Data"=variant} ("Time-Gated Phasor Q Element"), "Data"=w1417) -> (w1419:T26)
            n578 = Build Array(w1419) -> (w1416:T26[])
          }
        }
      }
      event "Time Step": Value Change {
        n579 = event-data() -> ("CtlRef"=w1432:refnum<vi>)  [unwired: 1 in]
        n580 = property class="DigNum (strict)"(reference=w1432) -> (reference out=w1429:refnum<vi>, error out=w1424:errorcluster, "Label.Text"=w1435:string, "Value"=w1430:dbl[unit])  [unwired: 1 in]
        n581 = call "AlliGator Update Settings & Control.vi"("Error In"=w1424, "Value"=w1430, "Sender"=w1431, "CtlRef"=w1429) -> ("Error Out"=w1423:errorcluster)  [unwired: 7 in]
        n582 = node(w1430) -> (w1433:dbl)
        n583 = property on="Intensity Time Trace" class="XYGraph (strict)"(error in=w1423, "XScale.Multiplier"=w1433) -> (error out=w1422:errorcluster)  [unwired: 1 in, 1 out]
        n584 = call "AlliGator Get Control Notebook String.vi"("error in (no error)"=w1422, "Value"=w1430, "Control Label"=w1435) -> ("error out"=w1434:errorcluster, "Notebook String"=w1421:string)  [unwired: 7 in]
      }
      event "Use File Timestamp": Value Change {
        n585 = event-data() -> ("CtlRef"=w1443:refnum<vi>, "OldVal"=w1442:bool, "NewVal"=w1445:bool)  [unwired: 1 in]
        n586 = case shown="True" w1444 {
          tunnel: w1445 -> [_ w1450]
          tunnel: w1443 -> [w1448 _]
          tunnel: w1442 -> [w1447 _]
          tunnel: [w1446 _] -> w1437
          tunnel: [_ w1449] -> w1436
          frame False {
            n587 = property class="Bool (strict)"(reference=w1448, "Value"=w1447) -> (error out=w1446:errorcluster)  [unwired: 1 in, 1 out]
          }
          frame True {
            n588 = Bundle By Name(cluster=T26 {"AlliGator Q Event"=enum."Intensity Time Trace:Use File Timestamp", "Data"=variant} ("element"), "Data"=w1450) -> (w1451:T26)
            n589 = Build Array(w1451) -> (w1449:T26[])
          }
        }
      }
      event "Use Intensity Correction File": Value Change {
        n590 = event-data() -> ("NewVal"=w1462:bool, "CtlRef"=w1463:refnum<vi>, "OldVal"=w1460:bool)  [unwired: 1 in]
        n591 = case shown="True" w1461 {
          tunnel: w1464 -> [_ w1477]
          tunnel: w1463 -> [w1467 w1475]
          tunnel: w1462 -> [_ w1473]
          tunnel: w1460 -> [w1466 _]
          tunnel: [w1465 w1476] -> w1455
          tunnel: [_ w1469] -> w1454
          tunnel: [_ w1468] -> w1453
          frame False {
            n592 = property class="Bool (strict)"(reference=w1467, "Value"=w1466) -> (error out=w1465:errorcluster)  [unwired: 1 in, 1 out]
          }
          frame True {
            n593 = local read "Intensity Correction File"() -> (w1472:path)
            n594 = property class="Bool (strict)"(reference=w1475) -> (reference out=w1479:refnum<vi>, error out=w1471:errorcluster, "Label.Text"=w1480:string, "Value"=w1478:bool)  [unwired: 1 in]
            n595 = Empty String/Path?(string/path=w1472) -> (empty?=w1481:bool)
            n596 = Compound Arithmetic op=AND(w1473, invert w1481) -> (w1474:bool)
            n597 = case shown="True" w1474 {
              tunnel: w1472 -> [_ w1483]
              tunnel: [_ w1482] -> w1469
              frame False {
              }
              frame True {
                n598 = Bundle By Name(cluster=T26 {"AlliGator Q Event"=enum."Intensity Time Trace:Load Intensity Corrections File", "Data"=variant} ("Time-Gated Phasor Q Element"), "Data"=w1483) -> (w1484:T26)
                n599 = Build Array(w1484) -> (w1482:T26[])
              }
            }
            n600 = call "AlliGator Update Settings & Control.vi"("Error In"=w1471, "Value"=w1478, "Sender"=w1477, "CtlRef"=w1479) -> ("Error Out"=w1470:errorcluster)  [unwired: 7 in]
            n601 = call "AlliGator Get Control Notebook String.vi"("error in (no error)"=w1470, "Value"=w1478, "Control Label"=w1480) -> ("error out"=w1476:errorcluster, "Notebook String"=w1468:string)  [unwired: 7 in]
          }
        }
      }
      event "Use ROI as Search Area": Value Change {
        n602 = event-data() -> ("CtlRef"=w1492:refnum<vi>, "NewVal"=w1494:bool, "OldVal"=w1491:bool)  [unwired: 1 in]
        n603 = case shown="True" w1493 {
          tunnel: w1495 -> [_ _]
          tunnel: w1494 -> [_ w1499]
          tunnel: w1492 -> [w1497 _]
          tunnel: w1491 -> [w1496 _]
          tunnel: [_ T26[] [{"AlliGator Q Event"=enum."Image:Use ROI as Search Area", "Data"=variant}] ("element")] -> w1486
          frame False {
            n604 = property class="Bool (strict)"(reference=w1497, "Value"=w1496) -> ()  [unwired: 1 in, 2 out]
          }
          frame True {
            n605 = call "Alligator Variables Storage.vi"("Get(F)/Set"=TRUE, "AlliGator Variable"=AlliGator_Variables_List."GUI:Search ROI Used" ("Alligator Variable"), "Data in"=w1499) -> ()  [unwired: 6 in, 3 out]
          }
        }
      }
      event Mouse Enter {
        # "Decay Fit Parameter Map Display: Mouse Enter"
        n606 = event-data() -> ("CtlRef"=w1507:refnum<vi>)  [unwired: 1 in]
        n607 = case shown="True" w1508 {
          tunnel: [w1511 w1516] -> w1510
          tunnel: w1509 -> [w1511 w1515]
          tunnel: w1507 -> [_ w1512]
          tunnel: [_ w1513] -> w1502
          frame False {
          }
          frame True {
            n608 = Unbundle By Name(w1515) -> ("Decay Fit Parameter Map Display Event"=w1517:refnum<event-registration>)
            n609 = register-events(reference=w1517, T36 refnum ("event source"), w1512, w1512, w1512) -> (reference out=w1518:refnum<event-registration>, error out=w1513:errorcluster)  [unwired: 1 in]
            n610 = Bundle By Name(cluster=w1515, "Decay Fit Parameter Map Display Event"=w1518) -> (w1516:T27)
          }
        }
      }
      event Mouse Leave {
        # "Decay Fit Parameter Map Display: Mouse Leave"
        n611 = event-data() -> ("CtlRef"=w1524:refnum<vi>)  [unwired: 1 in]
        n612 = case shown="True" w1525 {
          tunnel: [w1528 w1533] -> w1527
          tunnel: w1526 -> [w1528 w1532]
          tunnel: w1524 -> [_ w1531]
          tunnel: [_ w1530] -> w1519
          frame False {
          }
          frame True {
            w1529 = refnum<vi> refnum ("event source")
            n613 = Unbundle By Name(w1532) -> ("Decay Fit Parameter Map Display Event"=w1534:refnum<event-registration>)
            n614 = register-events(reference=w1534, w1531, w1529, w1529, w1529) -> (reference out=w1535:refnum<event-registration>, error out=w1530:errorcluster)  [unwired: 1 in]
            n615 = Bundle By Name(cluster=w1532, "Decay Fit Parameter Map Display Event"=w1535) -> (w1533:T27)
          }
        }
      }
      event Mouse Move {
        # "Decay Fit Parameter Map Display: Mouse Move"
        n616 = event-data() -> ("CtlRef"=w1542:refnum<vi>)  [unwired: 1 in, 1 out]
        n617 = case shown="True" w1541 {
          tunnel: w1542 -> [_ w1544]
          tunnel: [_ w1543] -> w1538
          frame False {
          }
          frame True {
            n618 = Bundle By Name(cluster=T26 {"AlliGator Q Event"=enum."Decay Fit Parameter Map:Mouse Move", "Data"=variant} ("Array"), "Data"=w1544) -> (w1545:T26)
            n619 = Build Array(w1545) -> (w1543:T26[])
          }
        }
      }
      event Mouse Up {
        # "Decay Fit Parameter Map Display: Mouse Up"
        n620 = event-data() -> ("CtlRef"=w1554:refnum<vi>, "PlatMods.Alt"=w1547:bool)  [unwired: 1 in]
        n621 = case shown="True" w1553 {
          tunnel: w1554 -> [_ w1561]
          tunnel: [_ w1562] -> w1550
          tunnel: w1547 -> [_ w1556]
          frame False {
          }
          frame True {
            n622 = property class="ImageControl"(reference=w1561) -> (reference out=w1558:refnum<vi>, "ROI"=w1557:T57, "Current ROI Tool"=w1555:u32)  [unwired: 1 in, 1 out]
            n623 = Bundle By Name(cluster=T45 {"Current ROI Tool"=8, "ROI Descriptor"={"Global Rectangle"=[], "Contours"=[]}, "Shift"=FALSE, "Alt"=FALSE, "Image Display Refnum"=refnum} ("Phasor Plot Mouse Up Event Data"), "Image Display Refnum"=w1558, "ROI Descriptor"=w1557, "Current ROI Tool"=w1555, "Alt"=w1556) -> (w1559:T45)
            n624 = Bundle By Name(cluster=T26 {"AlliGator Q Event"=enum."Decay Fit Parameter Map:Mouse Up", "Data"=variant} ("Array"), "Data"=w1559) -> (w1563:T26)
            n625 = Build Array(w1563) -> (w1562:T26[])
          }
        }
      }
      event Mouse Down {
        w1569 = refnum<vi> refnum  # Decay Fit Parameter Map Display Range
        # "Decay Fit Parameter Map Display Range: Mouse Down"
        n626 = event-data() -> ("CtlRef"=w1568:refnum<vi>)  [unwired: 1 in]
        n627 = Unbundle By Name(w1574) -> ("Decay Fit Parameter Map Display Range Event"=w1572:refnum<event-registration>)
        n628 = register-events(reference=w1572, w1569, w1568, w1568, w1568) -> (reference out=w1573:refnum<event-registration>, error out=w1565:errorcluster)  [unwired: 1 in]
        n629 = Bundle By Name(cluster=w1574, "Decay Fit Parameter Map Display Range Event"=w1573) -> (w1575:T27)
      }
      event Mouse Leave {
        w1579 = refnum<vi> refnum  # Decay Fit Parameter Map Display Range
        # "Decay Fit Parameter Map Display Range: Mouse Up, Mouse Leave"
        n630 = event-data() -> ("CtlRef"=w1580:refnum<vi>)  [unwired: 1 in]
        n631 = Unbundle By Name(w1585) -> ("Decay Fit Parameter Map Display Range Event"=w1583:refnum<event-registration>)
        n632 = register-events(reference=w1583, w1580, w1579, w1579, w1579) -> (reference out=w1584:refnum<event-registration>, error out=w1576:errorcluster)  [unwired: 1 in]
        n633 = Bundle By Name(cluster=w1585, "Decay Fit Parameter Map Display Range Event"=w1584) -> (w1586:T27)
      }
      event Mouse Move {
        # "Decay Fit Parameter Map Display Range: Mouse Move"
        n634 = event-data() -> ("Time"=w1587:u32)  [unwired: 1 in]
        n635 = case shown="True" w1594 {
          tunnel: [_ w1598] -> w1588
          tunnel: w1587 -> [_ w1597]
          frame False {
          }
          frame True {
            w1596 = T26 {"AlliGator Q Event"=enum."Decay Fit Parameter Map:Display Range Mouse Move", "Data"=variant} ("Time-Gated Phasor Q Element")
            n636 = call "AlliGator Filter Event.vi"("Time"=w1597, "Time-Gated Phasor Q Element"=w1596) -> ("Filter Event?"=w1595:bool)  [unwired: 8 in, 1 out]
            n637 = case shown="False" w1595 {
              tunnel: [w1601 _] -> w1598
              tunnel: w1596 -> [w1599 _]
              frame False {
                n638 = local read "Decay Fit Parameter"() -> (w1600:T11)
                n639 = Bundle By Name(cluster=w1599, "Data"=w1600) -> (w1602:T26)
                n640 = Build Array(w1602) -> (w1601:T26[])
              }
              frame True {
              }
            }
          }
        }
      }
      event Mouse Enter {
        n641 = event-data() -> ("CtlRef"=w1603:refnum<vi>)  [unwired: 1 in]
        n642 = Unbundle By Name(w1606) -> ("Decay Graph Statistics TipStrip Event"=w1607:refnum<event-registration>)
        n643 = call "XY Graph Tipstrip Mouse Enter.vi"("Event Registration Refnum"=w1607, "XY Graph Refnum"=w1603) -> ("Event Registration Refnum"=w1605:refnum<event-registration>)  [unwired: 8 in, 1 out]
        n644 = Bundle By Name(cluster=w1606, "Decay Graph Statistics TipStrip Event"=w1605) -> (w1604:T27)
      }
      event Mouse Leave {
        n645 = event-data() -> ("CtlRef"=w1616:refnum<vi>)  [unwired: 1 in]
        n646 = Unbundle By Name(w1614) -> ("Decay Graph Statistics TipStrip Event"=w1615:refnum<event-registration>)
        n647 = call "XY Graph Tipstrip Mouse Leave.vi"("Event Registration Refnum"=w1615, "XY Graph Refnum"=w1616) -> ("Event Registration Refnum"=w1613:refnum<event-registration>)  [unwired: 8 in, 1 out]
        n648 = Bundle By Name(cluster=w1614, "Decay Graph Statistics TipStrip Event"=w1613) -> (w1612:T27)
      }
      event Mouse Move {
        n649 = event-data() -> ("CtlRef"=w1624:refnum<vi>, "Coords"=w1623:T37)  [unwired: 1 in]
        n650 = control-ref of="Decay Statistics TipStrip"() -> (w1621:refnum<vi>)
        n651 = call "XY Graph Set Plot TipStrip.vi"("TipStrip Refnum"=w1621, "Max Length (200)"=300, "Coords"=w1623, "XY Graph Refnum"=w1624) -> ()  [unwired: 5 in, 3 out]
      }
      event Mouse Enter {
        n652 = event-data() -> ("CtlRef"=w1629:refnum<vi>)  [unwired: 1 in]
        n653 = Unbundle By Name(w1632) -> ("Decay Graph TipStrip Event"=w1633:refnum<event-registration>)
        n654 = call "XY Graph Tipstrip Mouse Enter.vi"("Event Registration Refnum"=w1633, "XY Graph Refnum"=w1629) -> ("Event Registration Refnum"=w1631:refnum<event-registration>)  [unwired: 8 in, 1 out]
        n655 = Bundle By Name(cluster=w1632, "Decay Graph TipStrip Event"=w1631) -> (w1630:T27)
      }
      event Mouse Leave {
        n656 = event-data() -> ("CtlRef"=w1642:refnum<vi>)  [unwired: 1 in]
        n657 = Unbundle By Name(w1640) -> ("Decay Graph TipStrip Event"=w1641:refnum<event-registration>)
        n658 = call "XY Graph Tipstrip Mouse Leave.vi"("Event Registration Refnum"=w1641, "XY Graph Refnum"=w1642) -> ("Event Registration Refnum"=w1639:refnum<event-registration>)  [unwired: 8 in, 1 out]
        n659 = Bundle By Name(cluster=w1640, "Decay Graph TipStrip Event"=w1639) -> (w1638:T27)
      }
      event Mouse Move {
        n660 = event-data() -> ("CtlRef"=w1650:refnum<vi>, "Coords"=w1649:T37)  [unwired: 1 in]
        n661 = control-ref of="Decay Graph TipStrip"() -> (w1647:refnum<vi>)
        n662 = call "XY Graph Set Plot TipStrip.vi"("TipStrip Refnum"=w1647, "Max Length (200)"=300, "Coords"=w1649, "XY Graph Refnum"=w1650) -> ()  [unwired: 5 in, 3 out]
      }
      event Mouse Enter {
        n663 = event-data() -> ("CtlRef"=w1655:refnum<vi>)  [unwired: 1 in]
        n664 = Unbundle By Name(w1658) -> ("Intensity Time Trace TipStrip Event"=w1659:refnum<event-registration>)
        n665 = call "XY Graph Tipstrip Mouse Enter.vi"("Event Registration Refnum"=w1659, "XY Graph Refnum"=w1655) -> ("Event Registration Refnum"=w1657:refnum<event-registration>)  [unwired: 8 in, 1 out]
        n666 = Bundle By Name(cluster=w1658, "Intensity Time Trace TipStrip Event"=w1657) -> (w1656:T27)
      }
      event Mouse Leave {
        n667 = event-data() -> ("CtlRef"=w1668:refnum<vi>)  [unwired: 1 in]
        n668 = Unbundle By Name(w1666) -> ("Intensity Time Trace TipStrip Event"=w1667:refnum<event-registration>)
        n669 = call "XY Graph Tipstrip Mouse Leave.vi"("Event Registration Refnum"=w1667, "XY Graph Refnum"=w1668) -> ("Event Registration Refnum"=w1665:refnum<event-registration>)  [unwired: 8 in, 1 out]
        n670 = Bundle By Name(cluster=w1666, "Intensity Time Trace TipStrip Event"=w1665) -> (w1664:T27)
      }
      event Mouse Move {
        n671 = event-data() -> ("CtlRef"=w1676:refnum<vi>, "Coords"=w1675:T37)  [unwired: 1 in]
        n672 = control-ref of="Intensity Time Trace TipStrip"() -> (w1673:refnum<vi>)
        n673 = call "XY Graph Set Plot TipStrip.vi"("TipStrip Refnum"=w1673, "Max Length (200)"=300, "Coords"=w1675, "XY Graph Refnum"=w1676) -> ()  [unwired: 5 in, 3 out]
      }
      event Mouse Enter {
        n674 = event-data() -> ("CtlRef"=w1681:refnum<vi>)  [unwired: 1 in]
        n675 = Unbundle By Name(w1684) -> ("Lifetime Graph TipStrip Event"=w1685:refnum<event-registration>)
        n676 = call "XY Graph Tipstrip Mouse Enter.vi"("Event Registration Refnum"=w1685, "XY Graph Refnum"=w1681) -> ("Event Registration Refnum"=w1683:refnum<event-registration>)  [unwired: 8 in, 1 out]
        n677 = Bundle By Name(cluster=w1684, "Lifetime Graph TipStrip Event"=w1683) -> (w1682:T27)
      }
      event Mouse Leave {
        n678 = event-data() -> ("CtlRef"=w1694:refnum<vi>)  [unwired: 1 in]
        n679 = Unbundle By Name(w1692) -> ("Lifetime Graph TipStrip Event"=w1693:refnum<event-registration>)
        n680 = call "XY Graph Tipstrip Mouse Leave.vi"("Event Registration Refnum"=w1693, "XY Graph Refnum"=w1694) -> ("Event Registration Refnum"=w1691:refnum<event-registration>)  [unwired: 8 in, 1 out]
        n681 = Bundle By Name(cluster=w1692, "Lifetime Graph TipStrip Event"=w1691) -> (w1690:T27)
      }
      event Mouse Move {
        n682 = event-data() -> ("CtlRef"=w1702:refnum<vi>, "Coords"=w1701:T37)  [unwired: 1 in]
        n683 = control-ref of="Lifetime & Other Parameters Graph TipStrip"() -> (w1699:refnum<vi>)
        n684 = call "XY Graph Set Plot TipStrip.vi"("TipStrip Refnum"=w1699, "Max Length (200)"=300, "Coords"=w1701, "XY Graph Refnum"=w1702) -> ()  [unwired: 5 in, 3 out]
      }
      event User Event {
        # "AlliGator Settings: User Event"
        n685 = event-data() -> ("AlliGator Settings Message"=w1716:T58, "Sender"=w1714:string, "Control Label"=w1717:string, "Data"=w1715:variant)  [unwired: 1 in]
        n686 = Not Equal?(x=w1713, y=w1714) -> (x != y?=w1718:bool)
        n687 = case shown="True" w1718 {
          tunnel: w1717 -> [_ w1722]
          tunnel: w1716 -> [_ w1723]
          tunnel: w1707 -> [_ w1721]
          tunnel: w1715 -> [_ w1720]
          tunnel: [_ w1719] -> w1710
          frame False {
          }
          frame True {
            n688 = case shown="\"Refresh Parameter\"" w1723 {
              tunnel: w1722 -> [_ _ _ w1729 _]
              tunnel: w1721 -> [_ _ _ w1724 _]
              tunnel: w1720 -> [_ _ _ w1728 _]
              tunnel: [_ _ _ w1726 _] -> w1719
              frame "Idle", Default {
              }
              frame "Subscribe" {
              }
              frame "Unsubscribe" {
              }
              frame "Refresh Parameter" {
                n689 = call "AlliGator Refresh Single Setting.vi"("Data"=w1728, "Control Label"=w1729, "VI Ref in"=w1724) -> ("Error Out"=w1727:errorcluster, "VI Ref (dup)"=w1725:refnum<vi>)  [unwired: 7 in]
                n690 = case shown="\"\", Default" w1729 {
                  tunnel: w1725 -> [_ w1736 w1741 w1748]
                  tunnel: w1728 -> [_ w1734 w1739 w1747]
                  tunnel: w1727 -> [w1731 w1733 w1738 w1746]
                  tunnel: [w1730 w1732 w1737 w1743] -> w1726
                  frame "", Default {
                    n691 = call "Tiny Clear Error.vi"("Error In"=w1731) -> ("no Error Out"=w1730:errorcluster)  [unwired: 8 in]
                  }
                  frame "Phasor Graph Frequency" {
                    n692 = call "AlliGator Refresh Single Setting.vi"("Error In"=w1733, "Data"=w1734, "Control Label"="Phasor Plot Frequency", "VI Ref in"=w1736) -> ("Error Out"=w1732:errorcluster)  [unwired: 6 in, 1 out]
                  }
                  frame "Phasor Plot Frequency" {
                    n693 = call "AlliGator Refresh Single Setting.vi"("Error In"=w1738, "Data"=w1739, "Control Label"="Phasor Graph Frequency", "VI Ref in"=w1741) -> ("Error Out"=w1737:errorcluster)  [unwired: 6 in, 1 out]
                  }
                  frame "Phasor Frequency" {
                    n694 = call "Tiny Clear Error.vi"("Error In"=w1746) -> ("no Error Out"=w1742:errorcluster)  [unwired: 8 in]
                    n695 = call "AlliGator Refresh Single Setting.vi"("Error In"=w1742, "Data"=w1747, "Control Label"="Phasor Graph Frequency", "VI Ref in"=w1748) -> ("Error Out"=w1745:errorcluster)  [unwired: 6 in, 1 out]
                    n696 = call "AlliGator Refresh Single Setting.vi"("Error In"=w1742, "Data"=w1747, "Control Label"="Phasor Plot Frequency", "VI Ref in"=w1748) -> ("Error Out"=w1744:errorcluster)  [unwired: 6 in, 1 out]
                    n697 = Merge Errors(w1745, w1744) -> (w1743:errorcluster)
                  }
                }
              }
              frame "Refresh All Parameters" {
              }
            }
          }
        }
      }
      event User Event {
        # "Phasor Plot Color Map Picker: User Event"
        n698 = event-data() -> ("Phasor Color Map Picker Event"=w1757:T59)  [unwired: 1 in]
        n699 = case shown="True" w1756 {
          tunnel: w1757 -> [_ w1759]
          tunnel: [_ w1758] -> w1751
          frame False {
          }
          frame True {
            n700 = case shown="\"Vertex Update\"" w1759 {
              tunnel: [_ T26[] [{"AlliGator Q Event"=enum."Phasor Plot:Update Phasor Color Map Vertices", "Data"=variant}] ("element") _] -> w1758
              frame "Init", Default {
              }
              frame "Vertex Update" {
              }
              frame "Color Change" {
              }
            }
          }
        }
      }
      event Mouse Enter {
        # "Parameter Map Display: Mouse Enter"
        n701 = event-data() -> ("CtlRef"=w1766:refnum<vi>)  [unwired: 1 in]
        n702 = case shown="True" w1767 {
          tunnel: [w1770 w1775] -> w1769
          tunnel: w1768 -> [w1770 w1774]
          tunnel: w1766 -> [_ w1771]
          tunnel: [_ w1772] -> w1761
          frame False {
          }
          frame True {
            n703 = Unbundle By Name(w1774) -> ("Parameter Map Display Event"=w1776:refnum<event-registration>)
            n704 = register-events(reference=w1776, T36 refnum ("event source"), w1771, w1771, w1771) -> (reference out=w1777:refnum<event-registration>, error out=w1772:errorcluster)  [unwired: 1 in]
            n705 = Bundle By Name(cluster=w1774, "Parameter Map Display Event"=w1777) -> (w1775:T27)
          }
        }
      }
      event Mouse Leave {
        # "Parameter Map Display: Mouse Leave"
        n706 = event-data() -> ("CtlRef"=w1783:refnum<vi>)  [unwired: 1 in]
        n707 = case shown="True" w1784 {
          tunnel: [w1787 w1792] -> w1786
          tunnel: w1785 -> [w1787 w1791]
          tunnel: w1783 -> [_ w1790]
          tunnel: [_ w1789] -> w1778
          frame False {
          }
          frame True {
            w1788 = refnum<vi> refnum ("event source")
            n708 = Unbundle By Name(w1791) -> ("Parameter Map Display Event"=w1793:refnum<event-registration>)
            n709 = register-events(reference=w1793, w1790, w1788, w1788, w1788) -> (reference out=w1794:refnum<event-registration>, error out=w1789:errorcluster)  [unwired: 1 in]
            n710 = Bundle By Name(cluster=w1791, "Parameter Map Display Event"=w1794) -> (w1792:T27)
          }
        }
      }
      event Mouse Move {
        # "Parameter Map Display: Mouse Move"
        n711 = event-data() -> ("CtlRef"=w1801:refnum<vi>)  [unwired: 1 in, 1 out]
        n712 = case shown="True" w1800 {
          tunnel: w1801 -> [_ w1803]
          tunnel: [_ w1802] -> w1797
          frame False {
          }
          frame True {
            n713 = Bundle By Name(cluster=T26 {"AlliGator Q Event"=enum."Parameter Map:Mouse Move", "Data"=variant} ("Array"), "Data"=w1803) -> (w1804:T26)
            n714 = Build Array(w1804) -> (w1802:T26[])
          }
        }
      }
      event Mouse Up {
        # "Parameter Map Display: Mouse Up"
        n715 = event-data() -> ("CtlRef"=w1813:refnum<vi>, "PlatMods.Alt"=w1806:bool)  [unwired: 1 in]
        n716 = case shown="True" w1812 {
          tunnel: w1813 -> [_ w1815]
          tunnel: [_ w1821] -> w1809
          tunnel: w1806 -> [_ w1814]
          frame False {
          }
          frame True {
            n717 = property class="ImageControl"(reference=w1815) -> (reference out=w1820:refnum<vi>, "ROI"=w1819:T57, "Current ROI Tool"=w1818:u32)  [unwired: 1 in, 1 out]
            n718 = Bundle By Name(cluster=T45 {"Current ROI Tool"=8, "ROI Descriptor"={"Global Rectangle"=[], "Contours"=[]}, "Shift"=FALSE, "Alt"=FALSE, "Image Display Refnum"=refnum} ("Phasor Plot Mouse Up Event Data"), "Image Display Refnum"=w1820, "ROI Descriptor"=w1819, "Current ROI Tool"=w1818, "Alt"=w1814) -> (w1816:T45)
            n719 = Bundle By Name(cluster=T26 {"AlliGator Q Event"=enum."Parameter Map:Mouse Up", "Data"=variant} ("Array"), "Data"=w1816) -> (w1822:T26)
            n720 = Build Array(w1822) -> (w1821:T26[])
          }
        }
      }
      event Mouse Down {
        w1828 = refnum<vi> refnum  # Parameter Map Display Range
        # "Parameter Map Display Range: Mouse Down"
        n721 = event-data() -> ("CtlRef"=w1827:refnum<vi>)  [unwired: 1 in]
        n722 = Unbundle By Name(w1833) -> ("Parameter Map Display Range Event"=w1831:refnum<event-registration>)
        n723 = register-events(reference=w1831, w1828, w1827, w1827, w1827) -> (reference out=w1832:refnum<event-registration>, error out=w1824:errorcluster)  [unwired: 1 in]
        n724 = Bundle By Name(cluster=w1833, "Parameter Map Display Range Event"=w1832) -> (w1834:T27)
      }
      event Mouse Leave {
        w1838 = refnum<vi> refnum  # Parameter Map Display Range
        # "Parameter Map Display Range: Mouse Up, Mouse Leave"
        n725 = event-data() -> ("CtlRef"=w1839:refnum<vi>)  [unwired: 1 in]
        n726 = Unbundle By Name(w1844) -> ("Parameter Map Display Range Event"=w1842:refnum<event-registration>)
        n727 = register-events(reference=w1842, w1839, w1838, w1838, w1838) -> (reference out=w1843:refnum<event-registration>, error out=w1835:errorcluster)  [unwired: 1 in]
        n728 = Bundle By Name(cluster=w1844, "Parameter Map Display Range Event"=w1843) -> (w1845:T27)
      }
      event Mouse Move {
        # "Parameter Map Display Range: Mouse Move"
        n729 = event-data() -> ("Time"=w1846:u32)  [unwired: 1 in]
        n730 = case shown="True" w1853 {
          tunnel: [_ w1857] -> w1847
          tunnel: w1846 -> [_ w1855]
          frame False {
          }
          frame True {
            w1854 = T26 {"AlliGator Q Event"=enum."Parameter Map:Display Range Mouse Move", "Data"=variant} ("Time-Gated Phasor Q Element")
            n731 = call "AlliGator Filter Event.vi"("Time"=w1855, "Time-Gated Phasor Q Element"=w1854) -> ("Filter Event?"=w1856:bool)  [unwired: 8 in, 1 out]
            n732 = case shown="False" w1856 {
              tunnel: [w1863 _] -> w1857
              tunnel: w1854 -> [w1862 _]
              frame False {
                n733 = local read "Parameter Map Set"() -> (w1861:u16)
                n734 = local read "Map Parameter"() -> (w1860:u16)
                n735 = Bundle(cluster=T50 {"Parameter Map Set"=0, "Map Parameter"=0}, "Parameter Map Set"=w1861, "Map Parameter"=w1860) -> (w1859:T50)
                n736 = Bundle By Name(cluster=w1862, "Data"=w1859) -> (w1864:T26)
                n737 = Build Array(w1864) -> (w1863:T26[])
              }
              frame True {
              }
            }
          }
        }
      }
      event Mouse Down {
        w1870 = refnum<vi> refnum  # Phasor Plot Display Range
        # "Phasor Plot Display Range: Mouse Down"
        n738 = event-data() -> ("CtlRef"=w1871:refnum<vi>)  [unwired: 1 in]
        n739 = Unbundle By Name(w1874) -> ("Phasor Display Range Event"=w1872:refnum<event-registration>)
        n740 = register-events(reference=w1872, w1870, w1871, w1871, w1871) -> (reference out=w1873:refnum<event-registration>, error out=w1865:errorcluster)  [unwired: 1 in]
        n741 = Bundle By Name(cluster=w1874, "Phasor Display Range Event"=w1873) -> (w1875:T27)
      }
      event Mouse Move {
        # "Phasor Plot Display Range: Mouse Move"
        n742 = event-data() -> ("Time"=w1877:u32)  [unwired: 1 in]
        n743 = case shown="True" w1883 {
          tunnel: w1877 -> [_ w1886]
          tunnel: [_ w1887] -> w1876
          frame False {
          }
          frame True {
            w1884 = T26 {"AlliGator Q Event"=enum."Phasor Plot:Display Range Mouse Move", "Data"=variant} ("Time-Gated Phasor Q Element")
            n744 = call "AlliGator Filter Event.vi"("Time"=w1886, "Time-Gated Phasor Q Element"=w1884) -> ("Filter Event?"=w1885:bool)  [unwired: 8 in, 1 out]
            n745 = case shown="False" w1885 {
              tunnel: w1884 -> [w1889 _]
              tunnel: [w1888 _] -> w1887
              frame False {
                n746 = Build Array(w1889) -> (w1888:T26[])
              }
              frame True {
              }
            }
          }
        }
      }
      event Mouse Up; Mouse Leave {
        w1894 = refnum<vi> refnum  # Phasor Plot Display Range
        # "Phasor Plot Display Range: Mouse Up, Mouse Leave"
        n747 = event-data() -> ("CtlRef"=w1893:refnum<vi>)  [unwired: 1 in]
        n748 = Unbundle By Name(w1899) -> ("Phasor Display Range Event"=w1897:refnum<event-registration>)
        n749 = register-events(reference=w1897, w1893, w1894, w1894, w1894) -> (reference out=w1898:refnum<event-registration>, error out=w1890:errorcluster)  [unwired: 1 in]
        n750 = Bundle By Name(cluster=w1899, "Phasor Display Range Event"=w1898) -> (w1900:T27)
      }
      event Mouse Enter {
        n751 = event-data() -> ("CtlRef"=w1901:refnum<vi>)  [unwired: 1 in]
        n752 = Unbundle By Name(w1904) -> ("Phasor Graph TipStrip Event"=w1905:refnum<event-registration>)
        n753 = call "XY Graph Tipstrip Mouse Enter.vi"("Event Registration Refnum"=w1905, "XY Graph Refnum"=w1901) -> ("Event Registration Refnum"=w1903:refnum<event-registration>)  [unwired: 8 in, 1 out]
        n754 = Bundle By Name(cluster=w1904, "Phasor Graph TipStrip Event"=w1903) -> (w1902:T27)
      }
      event Mouse Leave {
        n755 = event-data() -> ("CtlRef"=w1914:refnum<vi>)  [unwired: 1 in]
        n756 = Unbundle By Name(w1912) -> ("Phasor Graph TipStrip Event"=w1913:refnum<event-registration>)
        n757 = call "XY Graph Tipstrip Mouse Leave.vi"("Event Registration Refnum"=w1913, "XY Graph Refnum"=w1914) -> ("Event Registration Refnum"=w1911:refnum<event-registration>)  [unwired: 8 in, 1 out]
        n758 = Bundle By Name(cluster=w1912, "Phasor Graph TipStrip Event"=w1911) -> (w1910:T27)
      }
      event Mouse Move {
        n759 = event-data() -> ("CtlRef"=w1922:refnum<vi>, "Coords"=w1921:T37)  [unwired: 1 in]
        n760 = control-ref of="Phasor Graph TipStrip"() -> (w1919:refnum<vi>)
        n761 = call "XY Graph Set Plot TipStrip.vi"("TipStrip Refnum"=w1919, "Max Length (200)"=300, "Coords"=w1921, "XY Graph Refnum"=w1922) -> ()  [unwired: 5 in, 3 out]
      }
      event Mouse Down {
        # "Phasor Plot Display: Mouse Down"
        n762 = event-data() -> ("CtlRef"=w1939:refnum<vi>, "Coords"=w1938:T37, "Button"=w1937:u16, "PlatMods.Shift"=w1934:bool, "PlatMods.Alt"=w1933:bool)  [unwired: 1 in]
        n763 = case shown="True" w1927 {
          tunnel: w1939 -> [_ w1948]
          tunnel: w1938 -> [_ w1947]
          tunnel: w1937 -> [_ w1946]
          tunnel: w1936 -> [w1940 w1945]
          tunnel: [w1940 w1944] -> w1935
          tunnel: w1934 -> [_ w1943]
          tunnel: w1933 -> [_ w1942]
          tunnel: [_ w1941] -> w1930
          frame False {
          }
          frame True {
            n764 = case shown="1" w1946 {
              tunnel: w1948 -> [_ w1954]
              tunnel: w1947 -> [_ _]
              tunnel: w1945 -> [w1949 w1955]
              tunnel: [w1949 w1956] -> w1944
              tunnel: w1943 -> [_ _]
              tunnel: w1942 -> [_ _]
              tunnel: [_ w1953] -> w1941
              frame 0, Default {
                # "right or middle button"
              }
              frame 1 {
                # "Left Button: look for mouse up"
                n765 = Unbundle By Name(w1955) -> ("Phasor Plot Display Event"=w1952:refnum<event-registration>)
                n766 = call "AlliGator Phasor Plot Display Mouse Down-Up Event Monitoring.vi"("Phasor Plot Display Event Registration"=w1952, "Phasor Plot Display Refnum"=w1954, "Look for Mouse Down(T)/Up(F)"=FALSE) -> ("Phasor Plot Display Event Registration"=w1951:refnum<event-registration>, "Error Out"=w1953:errorcluster)  [unwired: 11 in]
                n767 = Bundle By Name(cluster=w1955, "Phasor Plot Display Event"=w1951) -> (w1956:T27)
              }
            }
          }
        }
      }
      event Mouse Enter {
        # "Phasor Plot Display: Mouse Enter"
        n768 = event-data() -> ("CtlRef"=w1963:refnum<vi>)  [unwired: 1 in]
        n769 = case shown="True" w1957 {
          tunnel: [w1966 w1971] -> w1965
          tunnel: w1964 -> [w1966 w1970]
          tunnel: w1963 -> [_ w1967]
          tunnel: [_ w1968] -> w1958
          frame False {
          }
          frame True {
            n770 = Unbundle By Name(w1970) -> ("Phasor Plot Display Event"=w1972:refnum<event-registration>)
            n771 = register-events(reference=w1972, T36 refnum ("event source"), w1967, w1967, w1967, w1967) -> (reference out=w1973:refnum<event-registration>, error out=w1968:errorcluster)  [unwired: 1 in]
            n772 = Bundle By Name(cluster=w1970, "Phasor Plot Display Event"=w1973) -> (w1971:T27)
          }
        }
      }
      event Mouse Leave {
        # "Phasor Plot Display: Mouse Leave"
        n773 = event-data() -> ("CtlRef"=w1979:refnum<vi>)  [unwired: 1 in]
        n774 = case shown="True" w1980 {
          tunnel: [w1983 w1989] -> w1982
          tunnel: w1981 -> [w1983 w1988]
          tunnel: w1979 -> [_ w1987]
          tunnel: [_ w1985] -> w1974
          frame False {
          }
          frame True {
            w1986 = FALSE ("Visible")
            w1984 = refnum<vi> refnum ("event source")
            n775 = Unbundle By Name(w1988) -> ("Phasor Plot Display Event"=w1990:refnum<event-registration>)
            n776 = register-events(reference=w1990, w1987, w1984, w1984, w1984, w1984) -> (reference out=w1991:refnum<event-registration>, error out=w1985:errorcluster)  [unwired: 1 in]
            n777 = Bundle By Name(cluster=w1988, "Phasor Plot Display Event"=w1991) -> (w1989:T27)
            n778 = property on="Phasor Plot Phasor Ratio" class="DigNum (strict)"("Visible"=w1986) -> ()  [unwired: 2 in, 2 out]
            n779 = property on="Phasor at cursor (g, s)" class="Clust (strict)"("Visible"=w1986) -> ()  [unwired: 2 in, 2 out]
            n780 = property on="Phasor at cursor (m, phi)" class="Clust (strict)"("Visible"=w1986) -> ()  [unwired: 2 in, 2 out]
            n781 = property on="Phasor Plot Phase Lifetime" class="DigNum (strict)"("Visible"=w1986) -> ()  [unwired: 2 in, 2 out]
            n782 = property on="Phasor Plot Average Lifetime" class="DigNum (strict)"("Visible"=w1986) -> ()  [unwired: 2 in, 2 out]
            n783 = property on="Phasor Plot Modulus Lifetime" class="DigNum (strict)"("Visible"=w1986) -> ()  [unwired: 2 in, 2 out]
          }
        }
      }
      event Mouse Move {
        # "Phasor Plot Display: Mouse Move"
        n784 = event-data() -> ("Time"=w1992:u32, "CtlRef"=w2004:refnum<vi>, "Coords"=w2003:T37)  [unwired: 1 in]
        n785 = case shown="True" w1994 {
          tunnel: w2004 -> [_ w2016]
          tunnel: w2003 -> [_ _]
          tunnel: w2002 -> [w2007 w2023]
          tunnel: w2001 -> [w2008 w2024]
          tunnel: [w2008 w2022] -> w2000
          tunnel: [w2007 w2018] -> w1999
          tunnel: w1995 -> [w2006 w2021]
          tunnel: w1997 -> [w2005 w2020]
          tunnel: [w2005 w2017] -> w1998
          tunnel: [w2006 w2019] -> w1996
          tunnel: [_ w2015] -> w1993
          tunnel: w1992 -> [_ w2010]
          frame False {
          }
          frame True {
            w2009 = T26 {"AlliGator Q Event"=enum."Phasor Plot:Mouse Move", "Data"=variant} ("AlliGator Actions")
            n786 = call "AlliGator Filter Event.vi"("Time"=w2010, "Time-Gated Phasor Q Element"=w2009) -> ("Filter Event?"=w2011:bool)  [unwired: 8 in, 1 out]
            n787 = call "AlliGator Phasor Plot Mouse Move Flag.vi"("Read/Write"=Read-Write."Read") -> ("Flag (out)"=w2012:bool)  [unwired: 8 in]
            n788 = Compound Arithmetic op=OR(w2011, w2012) -> (w2013:bool)
            n789 = case shown="False" w2013 {
              tunnel: w2024 -> [w2044 w2048]
              tunnel: w2023 -> [w2043 w2047]
              tunnel: [w2042 w2048] -> w2022
              tunnel: w2021 -> [w2041 w2046]
              tunnel: w2020 -> [w2040 w2045]
              tunnel: [w2039 w2046] -> w2019
              tunnel: [w2038 w2047] -> w2018
              tunnel: [w2037 w2045] -> w2017
              tunnel: w2016 -> [w2033 _]
              tunnel: [w2030 _] -> w2015
              tunnel: w2009 -> [w2027 _]
              frame False {
                n790 = property class="ImageControl"(reference=w2033) -> (reference out=w2029:refnum<vi>, "Last Mouse Position"=w2028:cluster{"X":i32, "Y":i32})  [unwired: 1 in, 1 out]
                n791 = call "AlliGator Phasor Plot Mouse Move Flag.vi"("Flag (in)"=TRUE, "Read/Write"=Read-Write."Write") -> ()  [unwired: 7 in, 1 out]
                n792 = call-poly <vilib>:"Acquire Input Data.vi"("device ID"=w2044, "error in (no error)"=w2043) -> ("device ID"=w2042:refnum<k1>, "button info"=w2035:T60, "error out"=w2038:errorcluster)  [unwired: 14 in, 1 out]
                n793 = call-poly <vilib>:"Acquire Input Data.vi"("device ID"=w2041, "error in (no error)"=w2040) -> ("device ID"=w2039:refnum<k1>, "keys pressed"=w2034:T52, "error out"=w2037:errorcluster)  [unwired: 15 in]
                n794 = Bundle(cluster=T51 {"Image Control Refnum"=refnum, "Coords"={"Horizontal"=0, "Vertical"=0}, "button info"={"button 1"=FALSE, "button 2"=FALSE, "button 3"=FALSE, "button 4"=FALSE}, "keys pressed"=[]} ("Image User Event Data"), "Image Control Refnum"=w2029, "Coords"=w2028, "button info"=w2035, "keys pressed"=w2034) -> (w2031:T51)
                n795 = Bundle By Name(cluster=w2027, "Data"=w2031) -> (w2036:T26)
                n796 = Build Array(w2036) -> (w2030:T26[])
              }
              frame True {
              }
            }
          }
        }
      }
      event Mouse Up {
        n797 = event-data() -> ("CtlRef"=w2061:refnum<vi>, "Button"=w2056:u16, "PlatMods.Shift"=w2059:bool, "PlatMods.Alt"=w2053:bool)  [unwired: 1 in]
        n798 = case shown="True" w2060 {
          tunnel: w2061 -> [_ w2070]
          tunnel: w2059 -> [_ w2068]
          tunnel: w2056 -> [_ w2069]
          tunnel: w2058 -> [w2062 w2067]
          tunnel: [w2062 w2066] -> w2057
          tunnel: w2053 -> [_ w2065]
          tunnel: [_ w2064] -> w2052
          tunnel: [_ w2063] -> w2049
          frame False {
          }
          frame True {
            n799 = case shown="1" w2069 {
              tunnel: w2070 -> [_ w2085]
              tunnel: w2068 -> [_ w2074]
              tunnel: w2067 -> [w2071 w2083]
              tunnel: [w2071 w2088] -> w2066
              tunnel: w2065 -> [_ w2073]
              tunnel: [_ w2080] -> w2064
              tunnel: [_ w2076] -> w2063
              frame 0, Default {
              }
              frame 1 {
                # "Left Button"
                n800 = property class="ImageControl"(reference=w2085) -> (reference out=w2072:refnum<vi>, error out=w2080:errorcluster, "Current ROI Tool"=w2082:u32, "ROI"=w2075:T57)  [unwired: 1 in]
                n801 = Unbundle By Name(w2083) -> ("Phasor Plot Display Event"=w2087:refnum<event-registration>)
                n802 = Bundle By Name(cluster=T45 {"Current ROI Tool"=8, "ROI Descriptor"={"Global Rectangle"=[], "Contours"=[]}, "Shift"=FALSE, "Alt"=FALSE, "Image Display Refnum"=refnum} ("output cluster"), "Image Display Refnum"=w2072, "Current ROI Tool"=w2082, "ROI Descriptor"=w2075, "Shift"=w2074, "Alt"=w2073) -> (w2077:T45)
                n803 = call "AlliGator Phasor Plot Display Mouse Down-Up Event Monitoring.vi"("Phasor Plot Display Event Registration"=w2087, "Phasor Plot Display Refnum"=w2085, "Look for Mouse Down(T)/Up(F)"=TRUE) -> ("Phasor Plot Display Event Registration"=w2086:refnum<event-registration>)  [unwired: 11 in, 1 out]
                n804 = Bundle By Name(cluster=w2083, "Phasor Plot Display Event"=w2086) -> (w2088:T27)
                n805 = Bundle By Name(cluster=T26 {"AlliGator Q Event"=enum."Phasor Plot:Mouse Up", "Data"=variant} ("AlliGator Actions out"), "Data"=w2077) -> (w2078:T26)
                n806 = Build Array(w2078) -> (w2076:T26[])
              }
            }
          }
        }
      }
      event Mouse Down {
        # "Phasor Plot Display Range: Mouse Down"
        n807 = event-data() -> ("CtlRef"=w2093:refnum<vi>)  [unwired: 1 in]
        n808 = Unbundle By Name(w2098) -> ("Phasor Plot Display Range Event"=w2096:refnum<event-registration>)
        n809 = register-events(reference=w2096, refnum<vi> refnum ("event source"), w2093, w2093, w2093) -> (reference out=w2097:refnum<event-registration>, error out=w2090:errorcluster)  [unwired: 1 in]
        n810 = Bundle By Name(cluster=w2098, "Phasor Plot Display Range Event"=w2097) -> (w2099:T27)
      }
      event Mouse Leave {
        w2103 = refnum<vi> refnum ("event source")
        # "Phasor Plot Display Range: Mouse Up, Mouse Leave"
        n811 = event-data() -> ("CtlRef"=w2104:refnum<vi>)  [unwired: 1 in]
        n812 = Unbundle By Name(w2109) -> ("Phasor Plot Display Range Event"=w2107:refnum<event-registration>)
        n813 = register-events(reference=w2107, w2104, w2103, w2103, w2103) -> (reference out=w2108:refnum<event-registration>, error out=w2100:errorcluster)  [unwired: 1 in]
        n814 = Bundle By Name(cluster=w2109, "Phasor Plot Display Range Event"=w2108) -> (w2110:T27)
      }
      event Mouse Move {
        # "Phasor Plot Display Range: Mouse Move"
        n815 = event-data() -> ("Time"=w2111:u32)  [unwired: 1 in]
        n816 = case shown="True" w2118 {
          tunnel: [_ w2122] -> w2112
          tunnel: w2111 -> [_ w2120]
          frame False {
          }
          frame True {
            w2119 = T26 {"AlliGator Q Event"=enum."Phasor Plot:Display Range Mouse Move", "Data"=variant} ("Time-Gated Phasor Q Element")
            n817 = call "AlliGator Filter Event.vi"("Time"=w2120, "Time-Gated Phasor Q Element"=w2119) -> ("Filter Event?"=w2121:bool)  [unwired: 8 in, 1 out]
            n818 = case shown="False" w2121 {
              tunnel: [w2124 _] -> w2122
              tunnel: w2119 -> [w2123 _]
              frame False {
                n819 = Build Array(w2123) -> (w2124:T26[])
              }
              frame True {
              }
            }
          }
        }
      }
      event Mouse Enter {
        n820 = event-data() -> ("CtlRef"=w2125:refnum<vi>)  [unwired: 1 in]
        n821 = Unbundle By Name(w2128) -> ("Phasor Ratio Graph TipStrip Event"=w2129:refnum<event-registration>)
        n822 = call "XY Graph Tipstrip Mouse Enter.vi"("Event Registration Refnum"=w2129, "XY Graph Refnum"=w2125) -> ("Event Registration Refnum"=w2127:refnum<event-registration>)  [unwired: 8 in, 1 out]
        n823 = Bundle By Name(cluster=w2128, "Phasor Ratio Graph TipStrip Event"=w2127) -> (w2126:T27)
      }
      event Mouse Leave {
        n824 = event-data() -> ("CtlRef"=w2138:refnum<vi>)  [unwired: 1 in]
        n825 = Unbundle By Name(w2136) -> ("Phasor Ratio Graph TipStrip Event"=w2137:refnum<event-registration>)
        n826 = call "XY Graph Tipstrip Mouse Leave.vi"("Event Registration Refnum"=w2137, "XY Graph Refnum"=w2138) -> ("Event Registration Refnum"=w2135:refnum<event-registration>)  [unwired: 8 in, 1 out]
        n827 = Bundle By Name(cluster=w2136, "Phasor Ratio Graph TipStrip Event"=w2135) -> (w2134:T27)
      }
      event Mouse Move {
        n828 = event-data() -> ("CtlRef"=w2146:refnum<vi>, "Coords"=w2145:T37)  [unwired: 1 in]
        n829 = control-ref of="Phasor Ratio Graph TipStrip"() -> (w2143:refnum<vi>)
        n830 = call "XY Graph Set Plot TipStrip.vi"("TipStrip Refnum"=w2143, "Max Length (200)"=300, "Coords"=w2145, "XY Graph Refnum"=w2146) -> ()  [unwired: 5 in, 3 out]
      }
      event Mouse Down {
        # "Source Image Display: Mouse Down"
        n831 = event-data() -> ("CtlRef"=w2162:refnum<vi>, "PlatMods.Shift"=w2161:bool, "PlatMods.Alt"=w2160:bool, "Button"=w2157:u16)  [unwired: 1 in]
        n832 = case shown="True" w2152 {
          tunnel: w2162 -> [_ w2170]
          tunnel: w2161 -> [_ w2169]
          tunnel: w2160 -> [_ w2168]
          tunnel: [w2163 w2167] -> w2159
          tunnel: w2158 -> [w2163 w2166]
          tunnel: w2157 -> [_ w2165]
          tunnel: [_ w2164] -> w2151
          frame False {
          }
          frame True {
            n833 = case shown="1" w2165 {
              tunnel: w2170 -> [_ w2172]
              tunnel: w2169 -> [_ _]
              tunnel: w2168 -> [_ _]
              tunnel: [w2171 w2176] -> w2167
              tunnel: w2166 -> [w2171 w2175]
              tunnel: [_ w2174] -> w2164
              frame 2, Default {
                # "Right Button"
              }
              frame 1 {
                # "Left Button"
                n834 = Unbundle By Name(w2175) -> ("Source Image Display Event"=w2178:refnum<event-registration>)
                n835 = call "AlliGator Source Image Display Mouse Down-Up Event Monitoring.vi"("Source Image Display Event Registration"=w2178, "Source Image Display Refnum"=w2172, "Look for Mouse Down(T)/Up(F)"=FALSE) -> ("Source Image Display Event Registration"=w2177:refnum<event-registration>, "Error Out"=w2174:errorcluster)  [unwired: 11 in]
                n836 = Bundle By Name(cluster=w2175, "Source Image Display Event"=w2177) -> (w2176:T27)
              }
            }
          }
        }
      }
      event Mouse Enter {
        # "Soure Image Display: Mouse Enter"
        n837 = event-data() -> ("CtlRef"=w2185:refnum<vi>)  [unwired: 1 in]
        n838 = case shown="True" w2179 {
          tunnel: [w2188 w2193] -> w2187
          tunnel: w2186 -> [w2188 w2192]
          tunnel: w2185 -> [_ w2190]
          tunnel: [_ w2189] -> w2180
          frame False {
          }
          frame True {
            n839 = Unbundle By Name(w2192) -> ("Source Image Display Event"=w2194:refnum<event-registration>)
            n840 = register-events(reference=w2194, T36 refnum ("event source"), w2190, w2190, w2190) -> (reference out=w2195:refnum<event-registration>, error out=w2189:errorcluster)  [unwired: 2 in]
            n841 = Bundle By Name(cluster=w2192, "Source Image Display Event"=w2195) -> (w2193:T27)
          }
        }
      }
      event Mouse Leave {
        # "Source Image Display: Mouse Leave"
        n842 = event-data() -> ("CtlRef"=w2201:refnum<vi>)  [unwired: 1 in]
        n843 = case shown="True" w2202 {
          tunnel: [w2205 w2211] -> w2204
          tunnel: w2203 -> [w2205 w2210]
          tunnel: w2201 -> [_ w2209]
          tunnel: [_ w2207] -> w2196
          frame False {
          }
          frame True {
            w2208 = FALSE ("Visible")
            w2206 = refnum<vi> refnum ("event source")
            n844 = Unbundle By Name(w2210) -> ("Source Image Display Event"=w2212:refnum<event-registration>)
            n845 = register-events(reference=w2212, w2209, w2206, w2206, w2206, w2206) -> (reference out=w2213:refnum<event-registration>, error out=w2207:errorcluster)  [unwired: 1 in]
            n846 = Bundle By Name(cluster=w2210, "Source Image Display Event"=w2213) -> (w2211:T27)
            n847 = property on="Phasor Plot Phase Lifetime" class="DigNum (strict)"("Visible"=w2208) -> ()  [unwired: 2 in, 2 out]
            n848 = property on="Phasor Plot Phasor Ratio" class="DigNum (strict)"("Visible"=w2208) -> ()  [unwired: 2 in, 2 out]
            n849 = property on="Phasor at cursor (g, s)" class="Clust (strict)"("Visible"=w2208) -> ()  [unwired: 2 in, 2 out]
            n850 = property on="Phasor at cursor (m, phi)" class="Clust (strict)"("Visible"=w2208) -> ()  [unwired: 2 in, 2 out]
            n851 = property on="Phasor Plot Modulus Lifetime" class="DigNum (strict)"("Visible"=w2208) -> ()  [unwired: 2 in, 2 out]
            n852 = property on="Phasor Plot Average Lifetime" class="DigNum (strict)"("Visible"=w2208) -> ()  [unwired: 2 in, 2 out]
          }
        }
      }
      event Mouse Move {
        # "Source Image Display: Mouse Move"
        n853 = event-data() -> ("Time"=w2214:u32, "CtlRef"=w2225:refnum<vi>, "Coords"=w2224:T37)  [unwired: 1 in]
        n854 = call-poly <vilib>:"Acquire Input Data.vi"("device ID"=w2216, "error in (no error)"=w2219) -> ("device ID"=w2217:refnum<k1>, "keys pressed"=w2215:T52, "error out"=w2218:errorcluster)  [unwired: 15 in]
        n855 = case shown="True" w2220 {
          tunnel: w2225 -> [_ w2236]
          tunnel: w2224 -> [_ w2226]
          tunnel: [_ w2234] -> w2221
          tunnel: w2215 -> [_ w2235]
          tunnel: w2214 -> [_ w2228]
          frame False {
          }
          frame True {
            w2229 = T26 {"AlliGator Q Event"=enum."Image:Mouse Move", "Data"=variant} ("AlliGator Events")
            n856 = property on="Source Image" class="ImageControl"() -> (error out=w2233:errorcluster, "ROI"=w2238:T57)  [unwired: 2 in, 1 out]
            n857 = call "is ROI Empty.vi"("Current ROI Descriptor"=w2238) -> ("Empty ROI?"=w2237:bool)  [unwired: 8 in]
            n858 = case shown="False" w2237 {
              tunnel: w2238 -> [w2258 _]
              tunnel: w2233 -> [w2257 _]
              frame False {
                n859 = property on="Decay Fit Parameter Map Image" class="ImageControl"(error in=w2257, "ROI"=w2258) -> ()  [unwired: 1 in, 2 out]
              }
              frame True {
              }
            }
            n860 = call "AlliGator Source Image Display Mouse Move Flag.vi"("Read/Write"=Read-Write."Read") -> ("Flag (out)"=w2231:bool)  [unwired: 8 in]
            n861 = call "AlliGator Filter Event.vi"("Time"=w2228, "Time-Gated Phasor Q Element"=w2229) -> ("Filter Event?"=w2227:bool)  [unwired: 8 in, 1 out]
            n862 = Or(x=w2231, y=w2227) -> (x .or. y?=w2230:bool)
            n863 = case shown="False" w2230 {
              tunnel: w2236 -> [w2241 _]
              tunnel: w2235 -> [w2247 _]
              tunnel: [w2243 _] -> w2234
              tunnel: w2229 -> [w2245 _]
              tunnel: w2226 -> [_ _]
              frame False {
                n864 = local read "Tab Control"() -> (w2246:T3)
                n865 = property class="ImageControl"(reference=w2241) -> (reference out=w2240:refnum<vi>, "Last Mouse Position"=w2239:cluster{"X":i32, "Y":i32})  [unwired: 1 in, 1 out]
                n866 = case shown="\"Phasor Plot\"" w2246 {
                  tunnel: w2247 -> [_ w2255]
                  tunnel: w2245 -> [_ w2253]
                  tunnel: [_ w2250] -> w2244
                  tunnel: w2240 -> [_ w2249]
                  tunnel: w2239 -> [_ w2248]
                  frame "Image Histogram", Default {
                  }
                  frame "Phasor Plot" {
                    # "If the Phasor Plot Tab is visible, show phasor information there"
                    n867 = call "AlliGator Source Image Display Mouse Move Flag.vi"("Flag (in)"=TRUE, "Read/Write"=Read-Write."Write") -> ()  [unwired: 7 in, 1 out]
                    n868 = Bundle By Name(cluster=T51 {"Image Control Refnum"=refnum, "Coords"={"Horizontal"=0, "Vertical"=0}, "button info"={"button 1"=FALSE, "button 2"=FALSE, "button 3"=FALSE, "button 4"=FALSE}, "keys pressed"=[]} ("Image User Event Data"), "Image Control Refnum"=w2249, "Coords"=w2248, "keys pressed"=w2255) -> (w2254:T51)
                    n869 = Bundle By Name(cluster=w2253, "Data"=w2254) -> (w2250:T26)
                  }
                }
                n870 = Build Array(w2244, T26 {"AlliGator Q Event"=enum."Image:Update True Pixel Value", "Data"=variant} ("element")) -> (w2243:T26[])
              }
              frame True {
              }
            }
          }
        }
      }
      event Mouse Up {
        # "Source Image Display: Mouse Up"
        n871 = event-data() -> ("CtlRef"=w2270:refnum<vi>, "PlatMods.Shift"=w2261:bool, "PlatMods.Alt"=w2260:bool)  [unwired: 1 in]
        n872 = case shown="True" w2262 {
          tunnel: w2270 -> [_ w2272]
          tunnel: w2269 -> [w2271 w2276]
          tunnel: [w2271 w2277] -> w2268
          tunnel: [_ w2287] -> w2263
          tunnel: w2261 -> [_ w2283]
          tunnel: w2260 -> [_ w2282]
          tunnel: [_ w2274] -> w2259
          frame False {
          }
          frame True {
            n873 = Unbundle By Name(w2276) -> ("Source Image Display Event"=w2280:refnum<event-registration>)
            n874 = property class="ImageControl"(reference=w2272) -> (reference out=w2273:refnum<vi>, error out=w2275:errorcluster, "Current ROI Tool"=w2285:u32, "ROI"=w2284:T57)  [unwired: 1 in]
            n875 = Bundle By Name(cluster=T45 {"Current ROI Tool"=8, "ROI Descriptor"={"Global Rectangle"=[], "Contours"=[]}, "Shift"=FALSE, "Alt"=FALSE, "Image Display Refnum"=refnum} ("output cluster"), "Image Display Refnum"=w2273, "Current ROI Tool"=w2285, "ROI Descriptor"=w2284, "Shift"=w2283, "Alt"=w2282) -> (w2281:T45)
            n876 = call "AlliGator Source Image Display Mouse Down-Up Event Monitoring.vi"("Source Image Display Event Registration"=w2280, "Source Image Display Refnum"=w2273, "Error In"=w2275, "Look for Mouse Down(T)/Up(F)"=TRUE) -> ("Source Image Display Event Registration"=w2279:refnum<event-registration>, "Error Out"=w2274:errorcluster)  [unwired: 10 in]
            n877 = Bundle By Name(cluster=w2276, "Source Image Display Event"=w2279) -> (w2277:T27)
            n878 = Bundle By Name(cluster=T26 {"AlliGator Q Event"=enum."Image:Mouse Up", "Data"=variant} ("AlliGator Actions out"), "Data"=w2281) -> (w2288:T26)
            n879 = Build Array(w2288) -> (w2287:T26[])
          }
        }
      }
      event Mouse Down {
        # "Time Point Slider: Mouse Down"
        n880 = event-data() -> ("CtlRef"=w2295:refnum<vi>)  [unwired: 1 in]
        n881 = case shown="True" w2296 {
          tunnel: [w2299 w2304] -> w2298
          tunnel: w2297 -> [w2299 w2303]
          tunnel: w2295 -> [_ w2302]
          tunnel: [_ w2301] -> w2290
          frame False {
          }
          frame True {
            w2300 = refnum<vi> refnum ("event source")
            n882 = Unbundle By Name(w2303) -> ("Time Point Slider Event"=w2305:refnum<event-registration>)
            n883 = register-events(reference=w2305, w2300, w2302, w2302, w2300) -> (reference out=w2306:refnum<event-registration>, error out=w2301:errorcluster)  [unwired: 1 in]
            n884 = Bundle By Name(cluster=w2303, "Time Point Slider Event"=w2306) -> (w2304:T27)
          }
        }
      }
      event Mouse Move {
        # "Time Point Slider: Mouse Move"
        n885 = event-data() -> ("CtlRef"=w2311:refnum<vi>, "Time"=w2307:u32)  [unwired: 1 in]
        n886 = case shown="True" w2314 {
          tunnel: w2311 -> [_ w2319]
          tunnel: [_ w2318] -> w2308
          tunnel: w2307 -> [_ w2315]
          frame False {
          }
          frame True {
            w2316 = T26 {"AlliGator Q Event"=enum."GUI:Time Series Slider Moved", "Data"=variant} ("Time-Gated Phasor Q Element")
            n887 = call "AlliGator Filter Event.vi"("Time"=w2315, "Time-Gated Phasor Q Element"=w2316) -> ("Filter Event?"=w2317:bool)  [unwired: 8 in, 1 out]
            n888 = case shown="False" w2317 {
              tunnel: w2319 -> [w2323 _]
              tunnel: [w2321 _] -> w2318
              tunnel: w2316 -> [w2320 _]
              frame False {
                n889 = property class="Slide (strict)"(reference=w2323) -> ("Value"=w2322:u16)  [unwired: 1 in, 2 out]
                n890 = Bundle By Name(cluster=w2320, "Data"=w2322) -> (w2324:T26)
                n891 = Build Array(w2324) -> (w2321:T26[])
              }
              frame True {
              }
            }
          }
        }
      }
      event Mouse Up; Mouse Leave {
        # "Time Point Slider: Mouse Up, Mouse Leave"
        n892 = event-data() -> ("CtlRef"=w2331:refnum<vi>)  [unwired: 1 in]
        n893 = case shown="True" w2332 {
          tunnel: [w2335 w2346] -> w2334
          tunnel: w2333 -> [w2335 w2345]
          tunnel: w2331 -> [_ w2339]
          tunnel: [_ w2337] -> w2326
          tunnel: [_ w2336] -> w2325
          frame False {
          }
          frame True {
            w2342 = refnum<vi> refnum ("event source")
            n894 = property class="Slide (strict)"(reference=w2339) -> ("Value"=w2338:u16)  [unwired: 1 in, 2 out]
            n895 = Unbundle By Name(w2345) -> ("Time Point Slider Event"=w2344:refnum<event-registration>)
            n896 = register-events(reference=w2344, w2339, w2342, w2342, w2342) -> (reference out=w2343:refnum<event-registration>, error out=w2337:errorcluster)  [unwired: 1 in]
            n897 = Bundle By Name(cluster=T26 {"AlliGator Q Event"=enum."GUI:Time Series Slider Changed", "Data"=variant} ("Time-Gated Phasor Q Element"), "Data"=w2338) -> (w2340:T26)
            n898 = Build Array(w2340) -> (w2336:T26[])
            n899 = Bundle By Name(cluster=w2345, "Time Point Slider Event"=w2343) -> (w2346:T27)
          }
        }
      }
      event Menu Activation? {
        n900 = event-data() -> ("MenuRef"=w2355:refnum<k9>)  [unwired: 1 in]
        n901 = case shown="True" w2354 {
          tunnel: w2355 -> [_ w2362]
          tunnel: [_ w2361] -> w2349
          tunnel: w2348 -> [_ w2360]
          tunnel: w2347 -> [_ w2357]
          frame False {
          }
          frame True {
            n902 = Build Path(base path=w2357, name or relative path=path "AlliGator.rtm") -> (appended path=w2356:path)
            n903 = property class="VI"(reference=w2360, "RT Menu Path"=w2356) -> (error out=w2359:errorcluster)  [unwired: 1 in, 1 out]
            n904 = call "AlliGator Update Menu.vi"("Error In"=w2359, "Menu in"=w2362) -> ("Error Out"=w2361:errorcluster)  [unwired: 9 in]
          }
        }
        n905 = event-data() -> ()  [unwired: 2 in, 1 out]
      }
      event Menu Selection (User) {
        n906 = event-data() -> ("MenuRef"=w2374:refnum<k9>, "ItemPath"=w2373:string, "ItemTag"=w2368:string)  [unwired: 1 in]
        n907 = call-poly <vilib>:"Acquire Input Data.vi"("device ID"=w2387, "error in (no error)"=w2386) -> ("device ID"=w2384:refnum<k1>, "keys pressed"=w2383:T52, "error out"=w2385:errorcluster)  [unwired: 15 in]
        n908 = Index Array(array=w2383) -> (element=w2367:T34)  [unwired: 1 in]
        n909 = property on="Time Point Slide" class="Slide (strict)"() -> ("Visible"=w2372:bool)  [unwired: 2 in, 2 out]
        n910 = Select(t=w2368, s=w2378, f=w2391) -> (s? t:f=w2366:string)
        n911 = Equal?(x=w2367, y=T34."H" ("element")) -> (x = y?=w2365:bool)
        n912 = call "AlliGator Menu Items.vi"("Menu Item Tag"=w2368, "This VI"=w2371) -> ("Error Out"=w2376:errorcluster, "Message"=w2380:string, "Window opened?"=w2369:bool, "AlliGator Actions"=w2364:T26[])  [unwired: 6 in]
        n913 = call "AlliGator Conditional Menu Items.vi"("Dataset Series?"=w2372, "Help?"=w2365, "Menu Item Path"=w2373, "Menu Item Tag"=w2366, "menu reference"=w2374) -> ("Error Out"=w2377:errorcluster, "Quit?"=w2381:bool, "Message"=w2363:string, "AlliGator Actions"=w2382:T26[])  [unwired: 3 in]
        n914 = Concatenate Strings(w2363, w2380) -> (w2379:string)
        n915 = Build Array (concatenate)(w2382, w2364) -> (w2370:T26[])
        n916 = Select(t=w2377, s=w2378, f=w2376) -> (s? t:f=w2375:errorcluster)
        n917 = global write "AlliGator Globals.vi" "Window Just Opened"(w2369) -> ()
      }
      event Mouse Enter {
        # "Note: when dragging and dropping a file in the window, the \"Mouse Enter\" is not triggered, therefore this event is triggered for all other user actions, EXCEPT for drag & dropping"
        # "Makes File/Folder Path invisible to allow normal user interaction"
        n918 = event-data() -> ()  [unwired: 1 in, 1 out]
        n919 = call "AlliGator Hide Path Drop Boxes.vi"("Hide (F)/Show"=FALSE, "AlliGator Ctrl Refnums"=w2393) -> ()  [unwired: 9 in, 1 out]
      }
      event Mouse Leave {
        (unwired) FALSE
        # "If the user moves away from the window, we can show the (transparent) path control to allow the user to drag & drop a file in it."
        # "Makes File/Folder Path visible (but transparent) to allow the user to drop a file in the window"
        n920 = event-data() -> ()  [unwired: 1 in, 1 out]
        n921 = global read "AlliGator Globals.vi" "Window Just Opened"() -> (w2402:bool)
        n922 = Not(x=w2402) -> (.not. x?=w2399:bool)
        n923 = call "AlliGator Hide Path Drop Boxes.vi"("Hide (F)/Show"=w2399, "AlliGator Ctrl Refnums"=w2398) -> ()  [unwired: 9 in, 1 out]
        n924 = And(x=w2399, y=FALSE ("Mouse Leave")) -> (x .and. y?=w2400:bool)
        n925 = global write "AlliGator Globals.vi" "Window Just Opened"(w2400) -> ()
      }
      event Panel Close? {
        n926 = event-data() -> ()  [unwired: 1 in, 1 out]
        n927 = case shown="True" w2414 {
          tunnel: [_ w2419] -> w2408
          tunnel: w2413 -> [_ w2418]
          tunnel: [_ w2417] -> w2407
          frame False {
            n928 = One Button Dialog(message="First abort the current operation...") -> ()  [unwired: 1 in, 1 out]
            n929 = call "Play Error Sound.vi"() -> ()  [unwired: 27 in, 1 out]
          }
          frame True {
            n930 = call "AlliGator Quit Dialog.vi"("App name"=w2418) -> ("Quit?"=w2417:bool, "AlliGator Actions"=w2419:T26[])  [unwired: 9 in]
          }
        }
        n931 = event-data("Discard?"=TRUE) -> ()  [unwired: 1 in, 1 out]
      }
    }
    n932 = call "AlliGator Settings Storage.vi"("AlliGator Settings List"=AlliGator_Settings_List."Miscellaneous:Verbose Error Mode") -> ("Variant Data out"=w203:variant)  [unwired: 9 in, 1 out]
    n933 = call-poly "Variant to Data.vi"("Variant"=w203) -> ("Value"=w201:bool)  [unwired: 8 in]
    n934 = call "Get Current Message Text Format.vi"("Text Format"=Text_Format_List."Message") -> ("Message Formatting"=w197:T61)  [unwired: 8 in, 1 out]
    n935 = call "Send Message to Notebook.vi"("Text Formatting"=w197, "Error In"=w196, "Text"=w193, "Notebook Queue"=w189) -> ("Error Out"=w195:errorcluster, "Notebook Queue"=w194:refnum<queue>)  [unwired: 4 in]
    n936 = call "AlliGator Queue Non Empty Events.vi"("Actions"=w198, "AlliGator Q"=w190) -> ()  [unwired: 9 in, 1 out]
    n937 = call "Send Error to Notebook.vi"("error in (no error)"=w195, "Verbose Error Messages (T)"=w201, "State Machine Case Error Source"="Event Loop", "Notebook Q"=w194) -> ()  [unwired: 7 in, 1 out]
  }
  n938 = call <vilib>:"Simple Error Handler.vi"("error in (no error)"=w62) -> ()  [unwired: 4 in, 5 out]
  n939 = for {
    N: 10 -> [_]
    tunnel: [w2421] -> w76 mode=indexing
    tunnel: T16."Parameter Map" ("Tab Control") -> [w2420]
    i -> [w2422]
    n940 = Coerce To Type(0:w2422, 1:w2420) -> (2:w2421:T16)
  }
  n941 = call "Destroy Embedded Progress Bar.vi"("Error In"=w60, "Progress Bar Queue in"=w59) -> ()  [unwired: 9 in, 1 out]
  n942 = for {
    tunnel: w76 -> [w2423] mode=indexing
    n943 = case shown="\"Fluorescence Decay Statistics\"" w2423 {
      frame "Image Histogram" {
      }
      frame "Fluorescence Decay", Default {
      }
      frame "Fluorescence Decay Statistics" {
      }
      frame "Intensity Time Trace" {
      }
      frame "Phasor Plot" {
        n944 = property on="Phasor Plot ROI Color" class="ColBox"("Val(Sgnl)"="Phasor Plot ROI Color") -> ()  [unwired: 2 in, 2 out]
      }
      frame "Phasor Graph" {
      }
      frame "Phasor Ratio" {
      }
      frame "Lifetime & Other Parameters" {
      }
      frame "Decay Fit Parameters Map" {
        n945 = property on="Decay Fit Parameter Map Color Scale" class="ColRmp (strict)"("Scale.FormatString"="%.3g" ("Scale.Format String")) -> ()  [unwired: 2 in, 2 out]
        n946 = property on="Decay Fit Parameter Map ROI Color" class="ColBox"("Val(Sgnl)"="Decay Fit Parameter Map ROI Color") -> ()  [unwired: 2 in, 2 out]
      }
      frame "Parameter Map" {
        n947 = property on="Parameter Map Color Scale" class="ColRmp (strict)"("Scale.FormatString"="%.3g" ("Scale.Format String")) -> ()  [unwired: 2 in, 2 out]
        n948 = property on="Parameter Map ROI Color" class="ColBox"("Val(Sgnl)"="Parameter Map ROI Color") -> ()  [unwired: 2 in, 2 out]
      }
    }
  }
  n949 = flat-sequence {
    frame #0 {
      n950 = property on="Source Image ROI Color" class="ColBox"("Val(Sgnl)"="Source Image ROI Color") -> ()  [unwired: 2 in, 2 out]
      n951 = property on="Image Color Scale" class="ColRmp (strict)"("Scale.Format"=u8 8 ("Scale.Display Format:Format"), "Scale.Precision"=u8 1 ("Scale.Display Format:Precision")) -> ()  [unwired: 2 in, 2 out]
    }
  }
  n952 = call-poly <vilib>:"Close Input Device.vi"("error in (no error)"=w156, "device ID"=w157) -> ("error out"=w72:errorcluster)  [unwired: 8 in]
  n953 = call-poly <vilib>:"Close Input Device.vi"("error in (no error)"=w138, "device ID"=w137) -> ("error out"=w71:errorcluster)  [unwired: 8 in]
  n954 = Unregister For Events(event registration refnum=w175) -> (error out=w80:errorcluster)  [unwired: 1 in]
  n955 = Merge Errors(w80, w72, w71) -> (w67:errorcluster)
  n956 = call "Tiny Clear Error.vi"("Error In"=w67) -> ("no Error Out"=w66:errorcluster)  [unwired: 8 in]
  n957 = invoke class="VI" method="FP.Close"(reference=w18, error in=w66) -> ()  [unwired: 1 in, 3 out]
